vi "TestSequenceSubVI.vi"(0 "GuiRef":T2={"StringOut"=refnum, "AbortOnFail"=refnum, "SN"=refnum, "SN_Length"=refnum, "TestResult"=refnum, "CycleTime"=refnum, "ErrorCode"=refnum, "UUTStatus"=refnum, "DataBaseEnable?"=refnum, "DUTModel"=refnum, "FixtureID"=refnum, "OperatorID"=refnum, "SNReady"=refnum, "StopSlot"=refnum, "NextStep"=refnum, "PassYeild"=refnum, "Failed"=refnum, "Passed"=refnum, "Tested"=refnum, "TestItemsCtl"={"StepName"="", "TestEnable"=FALSE, "LoopCount"=0, "StopOnFail"=FALSE, "Index"=0, "TestName"="", "通道"="", "参数"="", "TimeStart"=0}, "ProcessBar"=refnum, "Slot"=enum."Slot1", "Row"=3, "States"=refnum, "TestMode"=refnum, "循环次数-DUT"=refnum, "波形图"=refnum, "产品型号"=refnum, "子面板"=refnum, "测试失败项目"=refnum, "测试结果"=refnum, "DUT"=refnum, "Starttime"=refnum, "SlotReady"=refnum, "版本信息"=refnum, "WIFI_1"=refnum, "WIFI_2"=refnum, "直通率"=refnum, "卡1开卡结果"=refnum, "卡2开卡结果"=refnum}, 7 "MSComm":refnum<k7>, 11 "error in":errorcluster, 14 "semaphore":T1 caption="信号量") -> (15 "error out":errorcluster)   [LabVIEW 2013]
uses:
  SystemCode/SysControl/Reference.ctl
  SystemCode/SysControl/TestItemsCTL.ctl
  SystemCode/SysControl/Slot.ctl
  SourceCode/PDINFO.ctl
  SystemCode/SysControl/LEDState.ctl
  <vilib>/measure/matone.llb/Extract Single Tone Information 1 Chan.vi
  SourceCode/GlobalValue.vi
  <vilib>/measure/madcrms.llb/Basic Averaged DC-RMS for 1 Chan.vi
  <vilib>/measure/matone.llb/SINAD Analyzer 1 Chan.vi
  <vilib>/addons/Sound and Vibration/svt_Distortion/SVT THD+N (Time) (1 Ch).vi
  <vilib>/ErrorRing/Error Ring.xnode
  <vilib>/measure/NI_MAPro.lvlib
  <vilib>/addons/Sound and Vibration/svt_Distortion/SoundVib_Distortion.lvlib
panel:
  out "错误输出":errorcluster
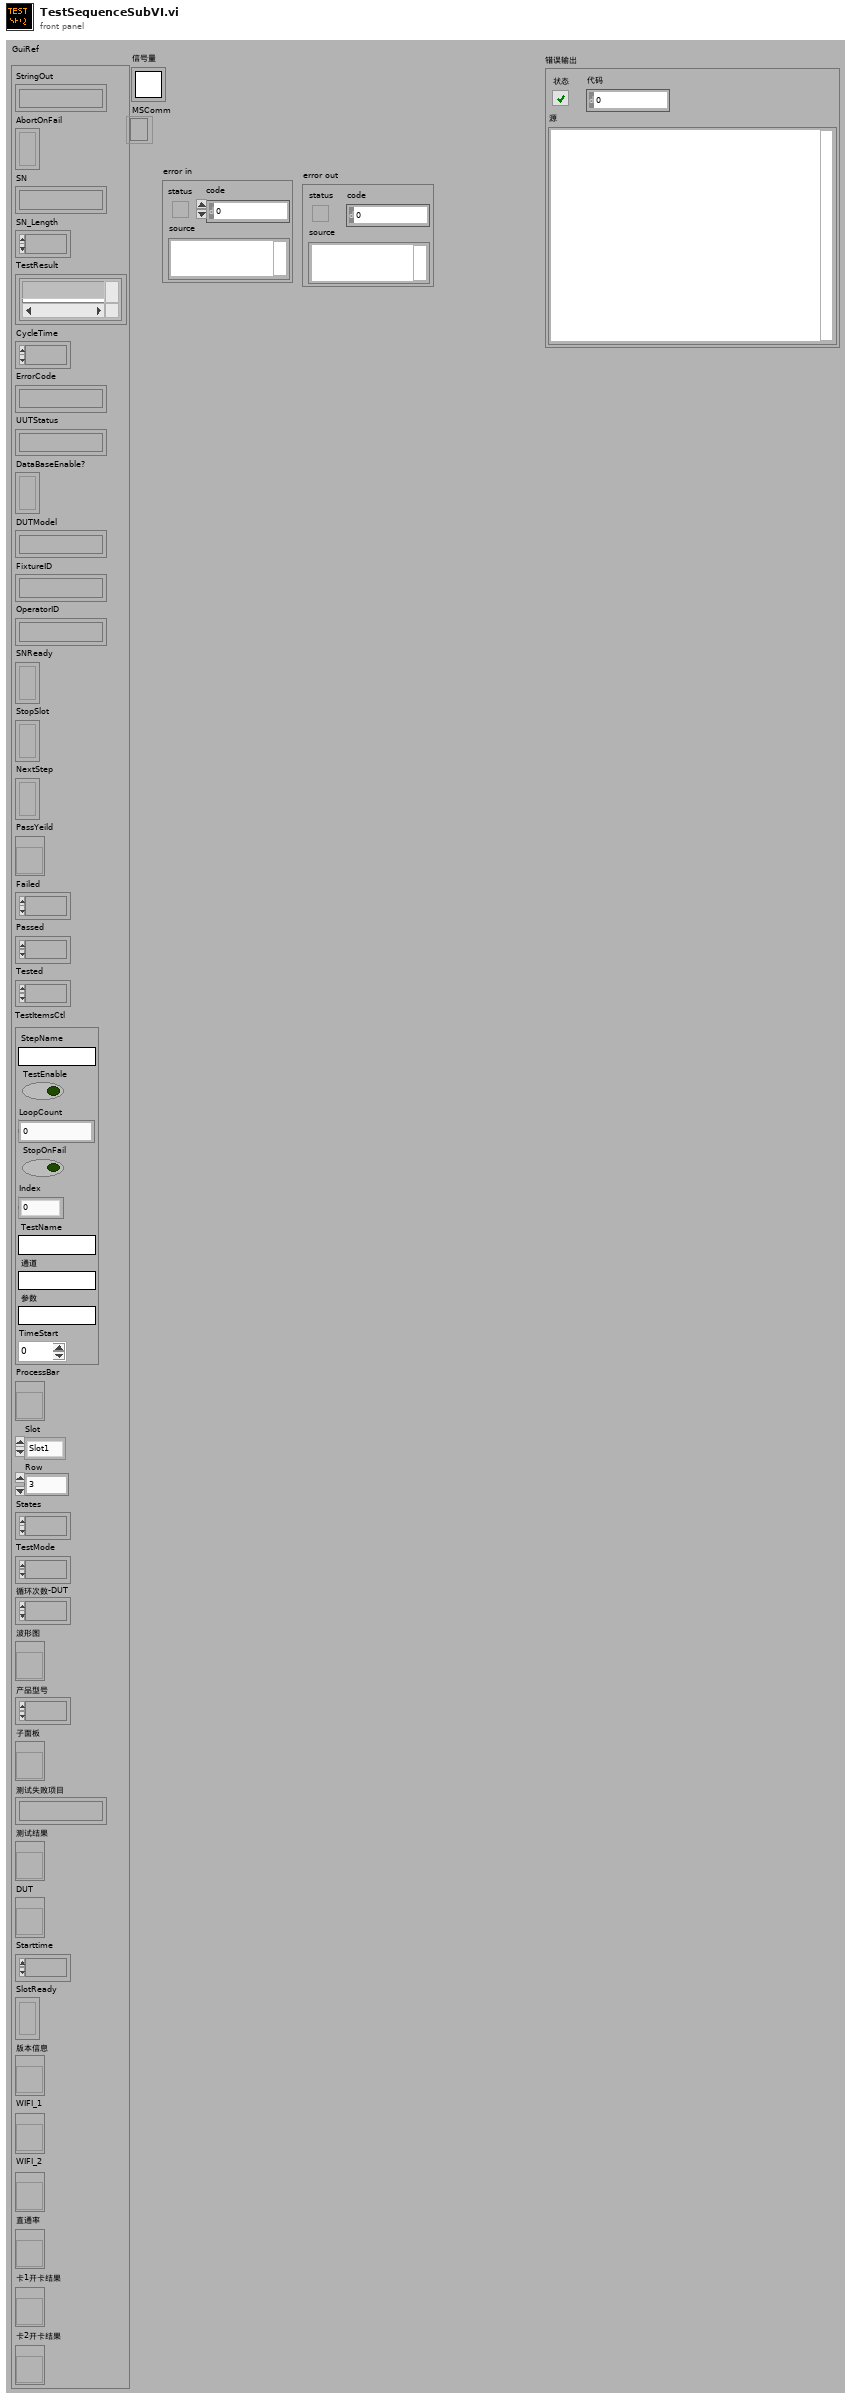
[diagram p1: front panel]
types:
  T1 = typedef "Semaphore RefNum" = refnum<k1>
  T2 = typedef "Reference.ctl" = cluster{"StringOut":refnum<vi>, "AbortOnFail":refnum<vi>, "SN":refnum<vi>, "SN_Length":refnum<vi>, "TestResult":refnum<vi>, "CycleTime":refnum<vi>, "ErrorCode":refnum<vi>, "UUTStatus":refnum<vi>, "DataBaseEnable?":refnum<vi>, "DUTModel":refnum<vi>, "FixtureID":refnum<vi>, "OperatorID":refnum<vi>, "SNReady":refnum<vi>, "StopSlot":refnum<vi>, "NextStep":refnum<vi>, "PassYeild":refnum<vi>, "Failed":refnum<vi>, "Passed":refnum<vi>, "Tested":refnum<vi>, "TestItemsCtl":T3, "ProcessBar":refnum<vi>, "Slot":T4, "Row":u32, "States":refnum<vi>, "TestMode":refnum<vi>, "循环次数-DUT":refnum<vi>, "波形图":refnum<vi>, "产品型号":refnum<vi>, "子面板":refnum<vi>, "测试失败项目":refnum<vi>, "测试结果":refnum<vi>, "DUT":refnum<vi>, "Starttime":refnum<vi>, "SlotReady":refnum<vi>, "版本信息":refnum<vi>, "WIFI_1":refnum<vi>, "WIFI_2":refnum<vi>, "直通率":refnum<vi>, "卡1开卡结果":refnum<vi>, "卡2开卡结果":refnum<vi>}
  T3 = typedef "TestItemsCTL.ctl" = cluster{"StepName":string, "TestEnable":bool, "LoopCount":i32, "StopOnFail":bool, "Index":u32, "TestName":string, "通道":string, "参数":string, "TimeStart":u32}
  T4 = typedef "Slot.ctl" = enum16{"Slot1", "Slot2", "Slot3", "Slot4"}
  T5 = typedef "PDINFO.ctl" = enum16{"Fw Ver", "HW Ver", "CCID", "WiFiName", "DevID", "SN", "TUID", "CertifID", "PdTime", "Provider", "WiFiPassword", "Imei", "AuthCode", "Reserved1", "Reserved2", "Reserved3"}
  T6 = cluster{"THD+N units":enum16{"dB", "linear ratio", "%"}, "detected fundamental amplitude units":enum16{"EU rms", "EU peak", "EU peak-peak"}}
  T7 = typedef "LEDState.ctl" = enum16{"默认", "闪烁", "停止闪烁", "真", "假"}
  T8 = cluster{"ID":u8, u8, u8, u8, "TimeStamp":u32, "TimeFlag":u8, "SendType":u8, "RemoteFlag":u8, "ExternFlag":u8, "DataLen":u8, "Byte0":u8, "Byte1":u8, "Byte2":u8, "Byte3":u8, "Byte4":u8, "Byte5":u8, "Byte6":u8, "Byte7":u8, "Channel":u8, u8, u8}
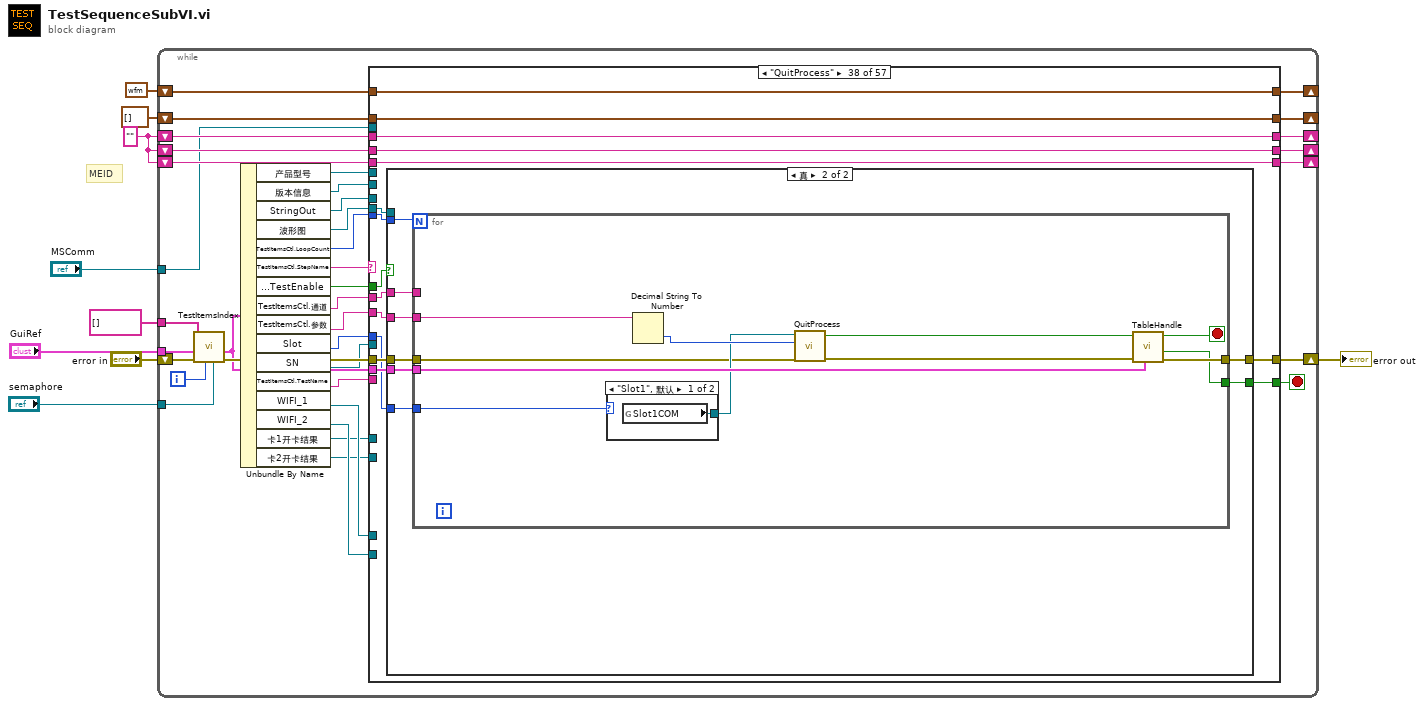
[diagram p0: block diagram]
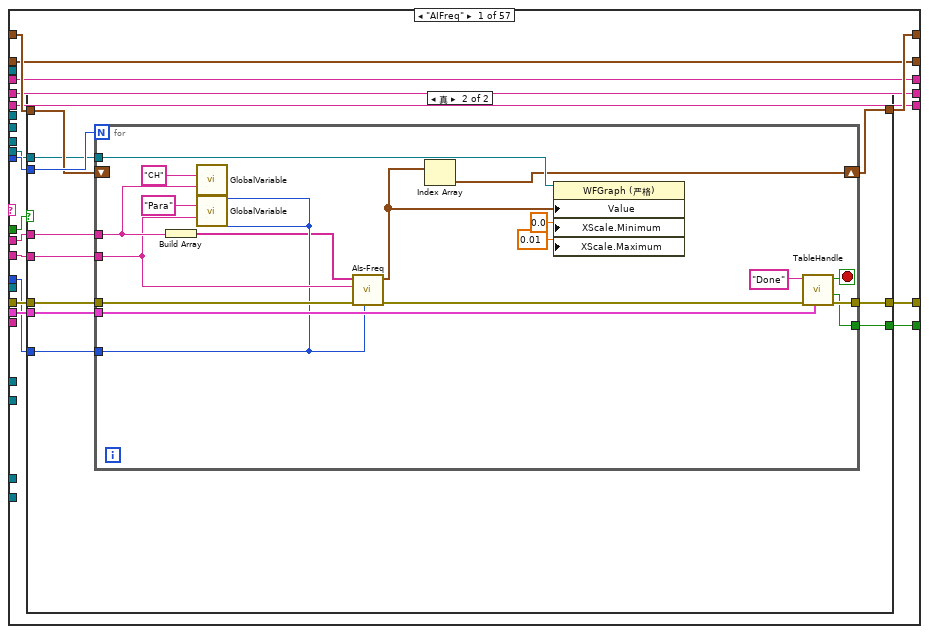
[diagram p2: hidden frame]
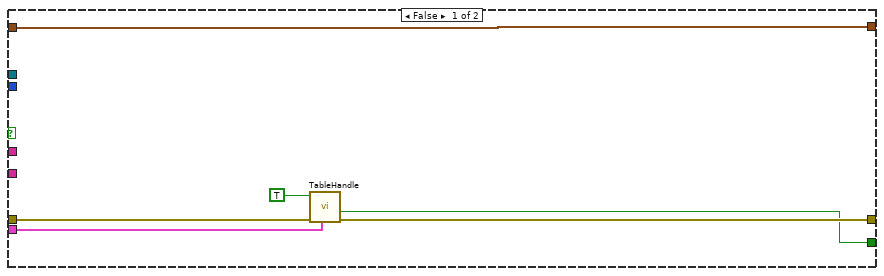
[diagram p3: hidden frame]
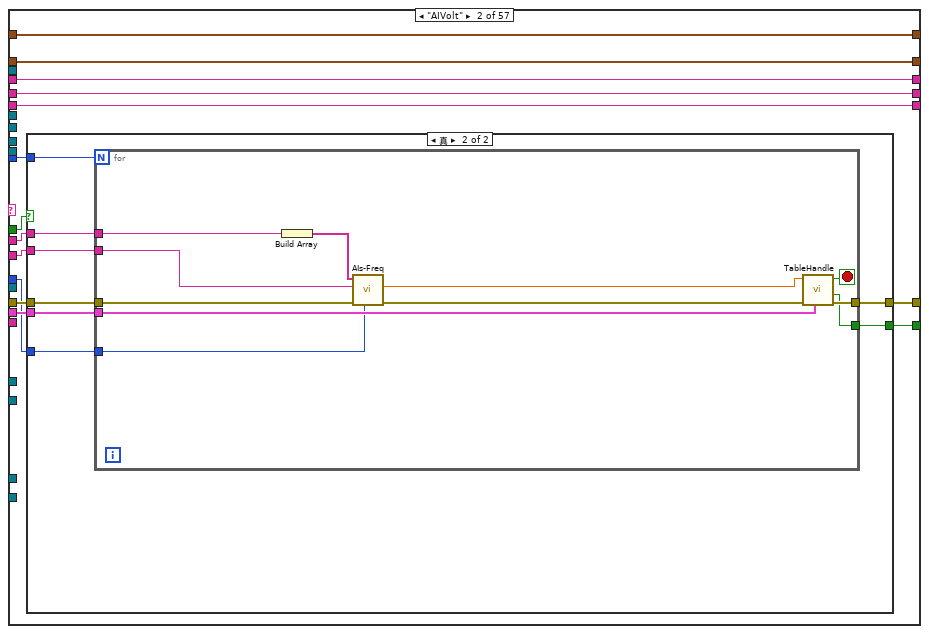
[diagram p4: hidden frame]
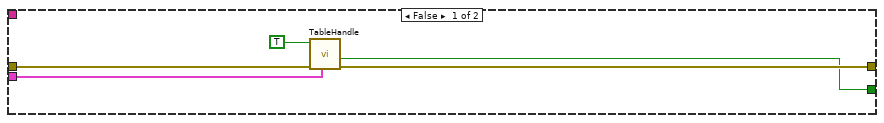
[diagram p5: hidden frame]
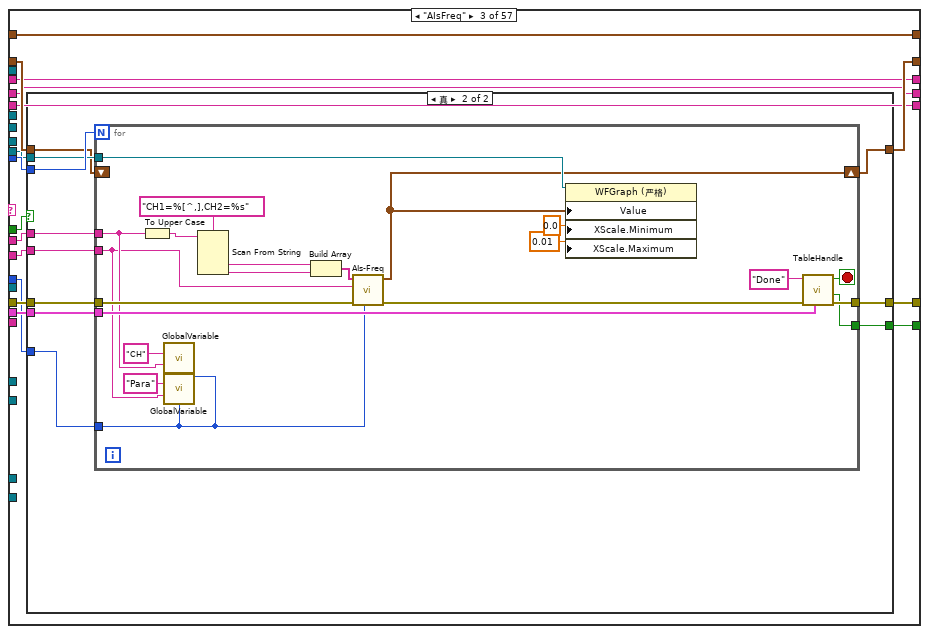
[diagram p6: hidden frame]
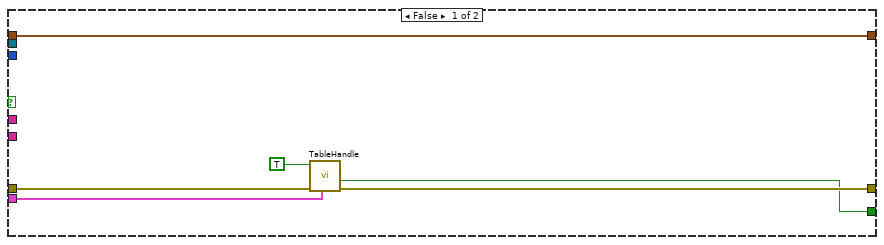
[diagram p7: hidden frame]
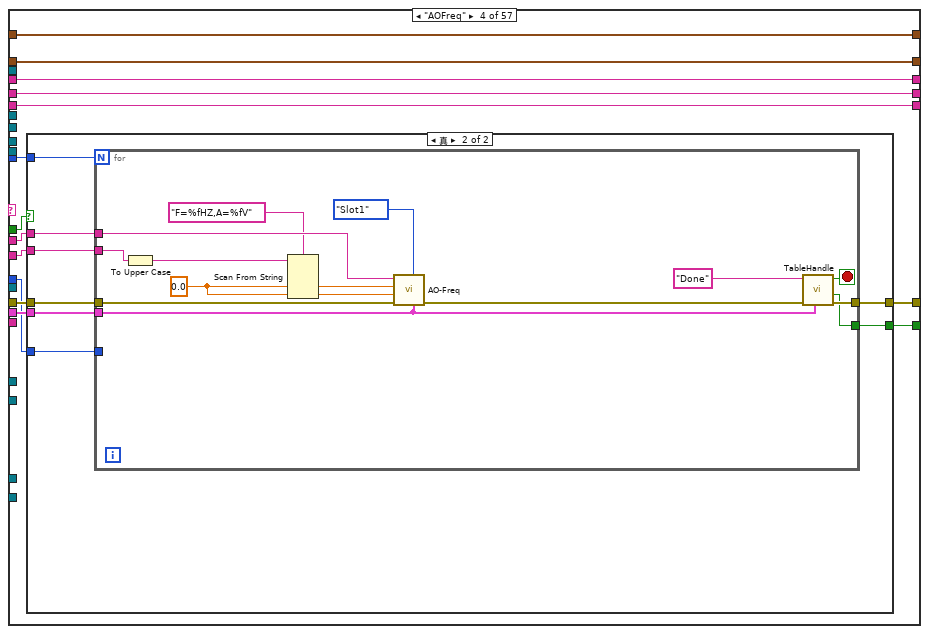
[diagram p8: hidden frame]
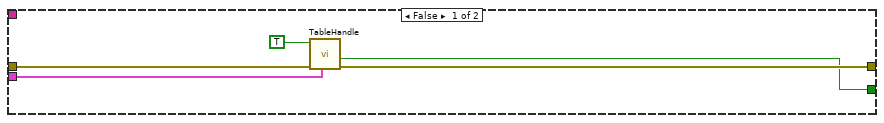
[diagram p9: hidden frame]
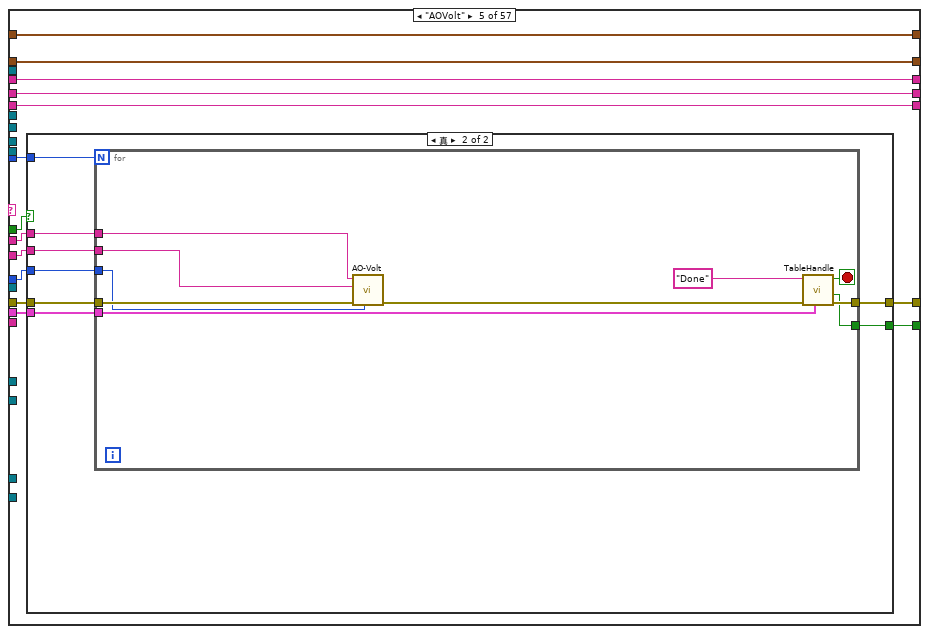
[diagram p10: hidden frame]
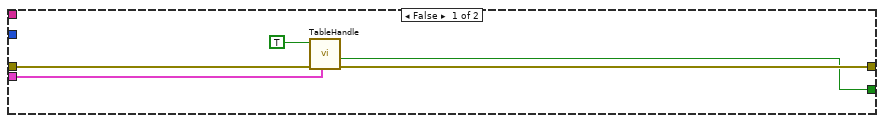
[diagram p11: hidden frame]
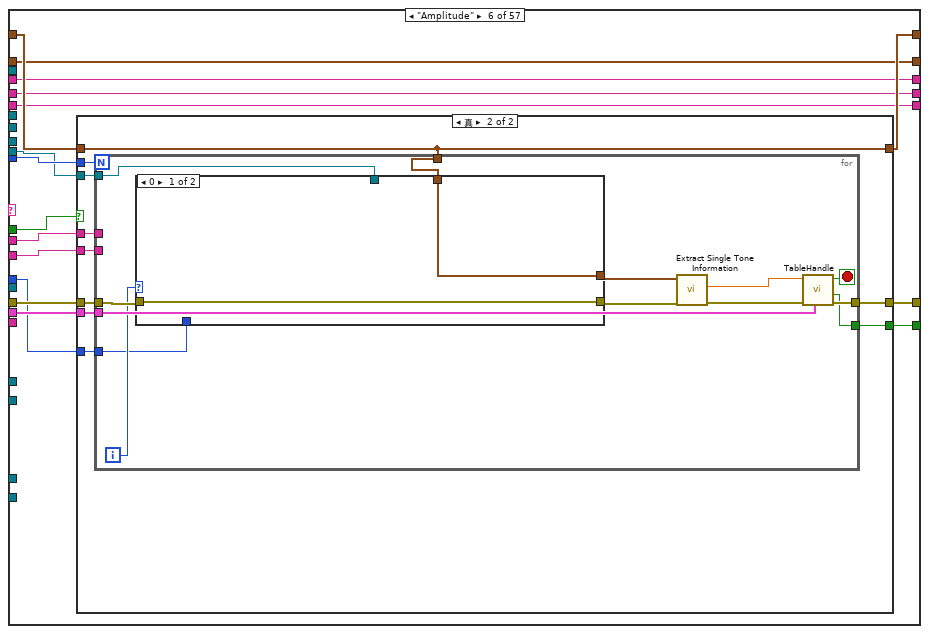
[diagram p12: hidden frame]
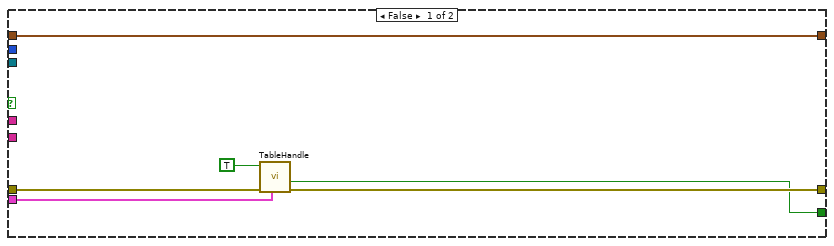
[diagram p13: hidden frame]
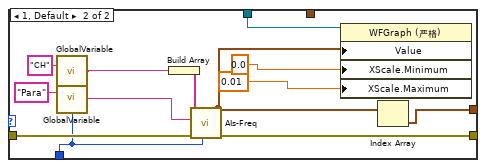
[diagram p14: hidden frame]
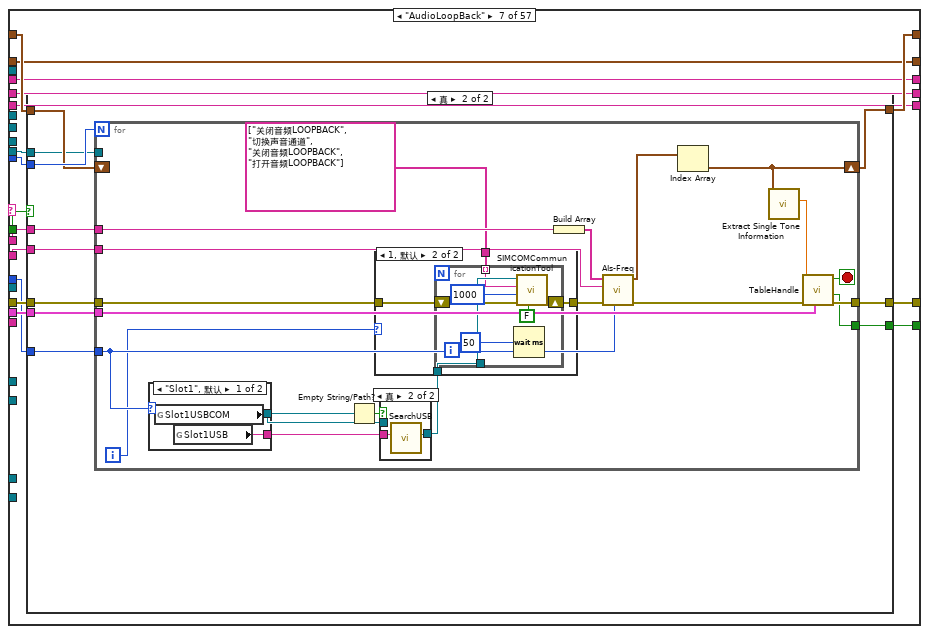
[diagram p15: hidden frame]
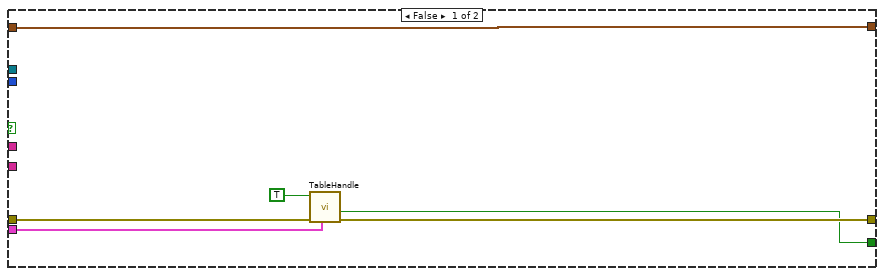
[diagram p16: hidden frame]
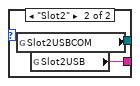
[diagram p19: hidden frame]
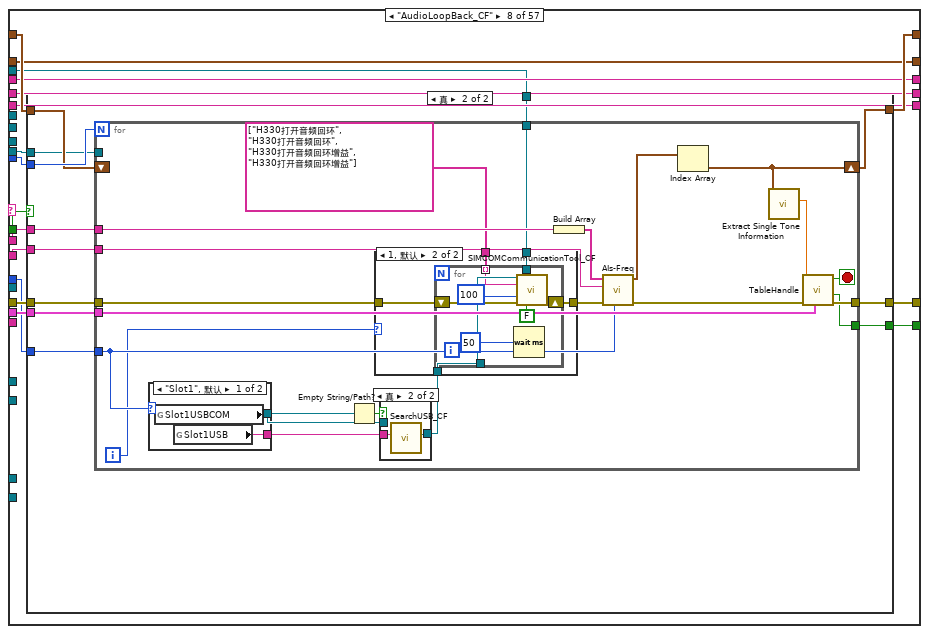
[diagram p20: hidden frame]
diagram:
  w2 = "" ("CMD")
  # "MEID"
  n1 = while {
    shift-right: [w41] -> w9
    shift-left: "error in" -> [w45]
    tunnel: "GuiRef" -> [w39]
    shift-right: [w33] -> _
    shift-left: waveform(dbl) {"t0"=timestamp(0 s since 1904-01-01), "dt"=1.0, "Y"=[]} ("Raw Data 3") -> [w32]
    shift-right: [w31] -> _
    shift-left: waveform(dbl)[] [] ("波形图") -> [w30]
    shift-right: [w27] -> _
    shift-left: w2 -> [w26]
    tunnel: string[] [] ("Fail项目") -> [w25]
    tunnel: "semaphore" -> [w23]
    shift-right: [w22] -> _
    shift-left: w2 -> [w21]
    shift-right: [w19] -> _
    shift-left: w2 -> [w20]
    tunnel: "MSComm" -> [w15]
    i -> [w24]
    stop <- w40 stop-if-true
    n2 = call "TestItemsIndex.vi"("semaphore"=w23, "TestItemIndexIn"=w24, "ErrorIn(NoError)"=w45, "GuiRef"=w39, "Fail项目"=w25) -> ("ErrorOut"=w44:errorcluster, "GuiRefOut"=w38:T2)  [unwired: 5 out]
    n3 = Unbundle By Name(w38) -> ("产品型号"=w16:refnum<vi>, "版本信息"=w18:refnum<vi>, "StringOut"=w28:refnum<vi>, "波形图"=w29:refnum<vi>, "TestItemsCtl.LoopCount"=w34:i32, "TestItemsCtl.StepName"=w43:string, "TestItemsCtl.TestEnable"=w42:bool, "TestItemsCtl.通道"=w35:string, "TestItemsCtl.参数"=w36:string, "Slot"=w37:T4, "SN"=w17:refnum<vi>, "TestItemsCtl.TestName"=w14:string, "WIFI_1"=w13:refnum<vi>, "WIFI_2"=w12:refnum<vi>, "卡1开卡结果"=w11:refnum<vi>, "卡2开卡结果"=w10:refnum<vi>)
    n4 = case shown="\"QuitProcess\"" w43 {
      selector: w43 -> [_ _ _ _ _ _ _ _ _ _ _ _ _ _ _ _ _ _ _ _ _ _ _ _ _ _ _ _ _ _ _ _ _ _ _ _ _ _ _ _ _ _ _ _ _ _ _ _ _ _ _ _ _ _ _ _ w3781]
      tunnel: [w59 w108 w148 w200 w242 w281 w341 w414 w491 w569 w647 w738 w825 w877 w929 w988 w1046 w1122 w1231 w1342 w1390 w1446 w1496 w1540 w1582 w1622 w1658 w1695 w1739 w1814 w1937 w2054 w2101 w2183 w2278 w2315 w2376 w2421 w2463 w2523 w2595 w2657 w2699 w2766 w2817 w2833 w2910 w2972 w3072 w3188 w3286 w3340 w3554 w3665 w3679 w3746 w3785] -> w41
      tunnel: w44 -> [w60 w109 w149 w201 w243 w282 w342 w415 w492 w570 w648 w739 w826 w878 w930 w989 w1047 w1123 w1232 w1343 w1391 w1447 w1497 w1541 w1583 w1623 w1659 w1696 w1740 w1815 w1938 w2055 w2105 w2184 w2279 w2316 w2377 w2422 w2464 w2524 w2596 w2658 w2700 w2770 w2817 w2834 w2911 w2973 w3073 w3189 w3287 w3331 w3555 w3665 w3680 w3747 _]
      tunnel: w38 -> [w61 w110 w150 w202 w244 w283 w343 w416 w493 w571 w649 w740 w827 w879 w931 w990 w1048 w1124 w1233 w1344 w1392 w1448 w1498 w1542 w1584 w1624 w1660 w1697 w1741 w1816 w1939 w2056 w2104 w2185 w2280 w2317 w2378 w2423 w2465 w2525 w2597 w2659 w2701 w2769 _ w2835 w2912 w2974 w3074 w3190 w3288 w3337 w3556 _ w3681 w3748 _]
      tunnel: w42 -> [w58 w107 w147 w199 w241 w280 w340 w413 w490 w568 w646 w737 w824 w876 w928 w987 w1045 w1121 w1230 w1341 w1389 w1445 w1495 w1539 w1581 w1621 w1657 w1694 w1738 w1813 w1936 w2053 w2108 w2182 w2277 w2314 w2375 w2420 w2462 w2522 w2594 w2656 w2698 w2764 _ w2832 w2909 w2971 w3071 w3187 w3285 w3332 w3553 _ w3678 w3745 _]
      tunnel: [w57 w106 w146 w198 w240 w279 w339 w412 w489 w567 w645 w736 w823 w875 w927 w986 w1044 w1120 w1229 w1340 w1388 w1444 w1494 w1538 w1580 w1620 w1656 w1693 w1737 w1812 w1935 w2052 w2100 w2181 w2276 w2313 w2374 w2419 w2461 w2521 w2593 w2655 w2697 w2767 TRUE ("StopOnFail?") w2831 w2908 w2970 w3070 w3186 w3284 w3339 w3552 FALSE ("StopOnFail?") w3677 w3744 TRUE ("StopOnFail?")] -> w40
      tunnel: w37 -> [w56 w105 w145 w197 w239 w278 w338 w411 w488 w566 w644 w735 w822 w874 w926 w985 w1043 w1119 w1228 w1339 w1387 w1443 w1493 w1537 w1579 w1619 w1655 w1692 w1736 w1811 w1934 w2051 w2103 w2180 w2275 w2312 w2373 w2418 w2460 w2520 w2592 w2654 w2696 w2768 _ w2830 w2907 w2969 w3069 w3185 w3283 w3341 w3551 _ w3676 w3743 w3776]
      tunnel: w36 -> [w54 w103 w143 w195 w237 w276 w336 w409 w486 w564 w642 w733 w820 w872 w924 w983 w1041 w1117 w1226 w1337 w1385 w1441 w1491 w1535 w1577 w1617 w1653 w1690 w1734 w1809 w1932 w2049 w2106 w2178 w2273 w2310 w2371 w2416 w2458 w2518 w2590 w2652 w2694 w2771 _ w2828 w2905 w2967 w3067 w3183 w3281 w3334 w3549 _ w3674 w3741 _]
      tunnel: w35 -> [w55 w104 w144 w196 w238 w277 w337 w410 w487 w565 w643 w734 w821 w873 w925 w984 w1042 w1118 w1227 w1338 w1386 w1442 w1492 w1536 w1578 w1618 w1654 w1691 w1735 w1810 w1933 w2050 w2107 w2179 w2274 w2311 w2372 w2417 w2459 w2519 w2591 w2653 w2695 w2772 _ w2829 w2906 w2968 w3068 w3184 w3282 w3342 w3550 _ w3675 w3742 _]
      tunnel: w34 -> [w53 w102 w142 w194 w236 w275 w335 w408 w485 w563 w641 w732 w819 w871 w923 w982 w1040 w1116 w1225 w1336 w1384 w1440 w1490 w1534 w1576 w1616 w1652 w1689 w1733 w1808 w1931 w2048 w2109 w2177 w2272 w2309 w2370 w2415 w2457 w2517 w2589 w2651 w2693 w2773 _ w2827 w2904 w2966 w3066 w3182 w3280 w3328 w3548 _ w3673 w3740 _]
      tunnel: [w52 w101 w141 w193 w235 w273 w334 w407 w484 w562 w640 w731 w818 w870 w922 w981 w1039 w1115 w1224 w1335 w1383 w1438 w1488 w1532 w1574 w1615 w1651 w1688 w1732 w1807 w1930 w2047 w2102 w2176 w2270 w2308 w2369 w2409 w2455 w2515 w2584 w2650 w2688 w2765 w2815 w2826 w2902 w2965 w3065 w3181 w3279 w3338 w3547 w3663 w3672 w3738 w3784] -> w33
      tunnel: w32 -> [w51 w101 w141 w193 w235 w274 w333 w406 w483 w561 w639 w730 w818 w870 w922 w981 w1039 w1115 w1224 w1335 w1383 w1439 w1489 w1533 w1575 w1615 w1651 w1688 w1732 w1807 w1930 w2047 w2102 w2176 w2271 w2308 w2369 w2409 w2456 w2516 w2584 w2650 w2688 w2765 w2815 w2826 w2903 w2965 w3065 w3181 w3279 w3338 w3547 w3663 w3672 w3739 w3784]
      tunnel: [w50 w100 w140 w192 w234 w272 w332 w405 w482 w560 w638 w729 w817 w869 w921 w980 w1038 w1114 w1223 w1334 w1382 w1437 w1487 w1531 w1573 w1614 w1650 w1687 w1731 w1806 w1929 w2046 w2112 w2175 w2269 w2307 w2368 w2414 w2454 w2514 w2588 w2649 w2692 w2777 w2814 w2825 w2901 w2964 w3064 w3180 w3278 w3345 w3546 w3662 w3671 w3737 w3783] -> w31
      tunnel: w30 -> [w50 w100 w139 w192 w234 w272 w332 w405 w482 w560 w638 w729 w817 w869 w921 w980 w1038 w1114 w1223 w1334 w1382 w1437 w1487 w1531 w1573 w1614 w1650 w1687 w1731 w1806 w1929 w2046 w2112 w2175 w2269 w2307 w2368 w2414 w2454 w2514 w2588 w2649 w2692 w2777 w2814 w2825 w2901 w2964 w3064 w3180 w3278 w3345 w3546 w3662 w3671 w3737 w3783]
      tunnel: w29 -> [w49 _ w138 _ _ w270 w331 w404 w481 w559 w637 w728 _ _ _ _ _ _ _ _ _ _ _ _ _ _ _ _ _ _ _ _ _ _ _ _ _ w2412 w2452 w2512 w2587 _ w2691 _ _ _ w2899 _ _ _ _ _ _ _ _ _ _]
      tunnel: w28 -> [_ _ _ _ _ _ _ _ _ _ w631 w722 w813 w868 w920 w979 w1037 w1113 w1222 w1333 w1381 _ _ _ _ _ _ _ w1730 w1805 w1928 _ w2099 _ _ _ _ _ _ _ w2583 _ w2687 _ _ w2824 _ w2963 w3063 w3179 _ w3330 w3542 _ w3667 _ _]
      tunnel: [w48 w97 w137 w191 w233 w271 w330 w403 w480 w558 w630 w721 w812 w867 w919 w978 w1036 w1112 w1221 w1331 w1379 w1436 w1486 w1530 w1572 w1613 w1649 w1686 w1729 w1804 w1927 w2045 w2096 w2174 w2268 w2306 w2367 w2413 w2453 w2513 w2580 w2648 w2684 w2776 w2813 w2823 w2900 w2962 w3062 w3178 w3277 w3329 w3541 w3661 w3666 w3736 w3778] -> w27
      tunnel: w26 -> [w48 w97 w137 w191 w233 w271 w330 w403 w480 w558 w632 w723 w814 w866 w918 w977 w1035 w1111 w1220 w1332 w1380 w1436 w1486 w1530 w1572 w1613 w1649 w1686 w1728 w1803 w1926 w2045 w2097 w2174 w2268 w2306 w2367 w2413 w2453 w2513 w2581 w2648 w2685 w2776 w2813 w2822 w2900 w2961 w3061 w3177 w3277 w3327 w3543 w3661 w3668 w3736 w3778]
      tunnel: [w47 w99 w136 w190 w232 w269 w329 w402 w479 w557 w636 w727 w816 w865 w917 w976 w1034 w1110 w1219 w1330 w1378 w1433 w1485 w1529 w1571 w1612 w1648 w1685 w1727 w1802 w1925 w2044 w2111 w2173 w2267 w2305 w2366 w2411 w2451 w2511 w2586 w2647 w2690 w2775 w2812 w2821 w2898 w2960 w3060 w3176 w3276 w3344 w3545 w3660 w3670 w3735 w3774] -> w22
      tunnel: w21 -> [w47 w99 w136 w190 w232 w269 w329 w402 w479 w557 w636 w727 w816 w865 w917 w976 w1034 w1110 w1219 w1330 w1378 w1433 w1485 w1529 w1571 w1612 w1648 w1685 w1727 w1802 w1925 w2044 w2111 w2173 w2267 w2305 w2366 w2411 w2451 w2511 w2586 w2647 w2690 w2775 w2812 w2821 w2898 w2959 w3059 w3175 w3276 w3344 w3545 w3660 w3670 w3735 w3774]
      tunnel: w20 -> [w46 w98 w135 w189 w231 w268 w328 w401 w478 w556 w635 w726 w815 w864 w916 w975 _ w1109 _ w1329 w1377 w1435 w1484 w1528 w1570 w1611 w1647 w1684 _ _ _ w2043 w2110 w2172 w2266 w2304 w2365 w2410 w2450 w2510 w2585 w2646 w2689 w2774 w2811 _ w2897 w2958 w3058 w3174 w3275 w3343 w3544 w3659 w3669 w3734 w3773]
      tunnel: [w46 w98 w135 w189 w231 w268 w328 w401 w478 w556 w635 w726 w815 w864 w916 w975 w1033 w1109 w1218 w1329 w1377 w1435 w1484 w1528 w1570 w1611 w1647 w1684 w1726 w1801 w1924 w2043 w2110 w2172 w2266 w2304 w2365 w2410 w2450 w2510 w2585 w2646 w2689 w2774 w2811 w2820 w2897 w2958 w3058 w3174 w3275 w3343 w3544 w3659 w3669 w3734 w3773] -> w19
      tunnel: w18 -> [_ _ _ _ _ _ _ _ _ _ _ _ _ _ _ _ w1032 _ w1217 _ _ _ _ _ _ _ _ _ w1725 w1800 w1923 _ _ _ _ _ _ _ _ _ _ _ _ _ _ w2819 _ _ _ _ _ _ _ _ _ _ _]
      tunnel: w17 -> [_ _ _ _ _ _ _ _ _ _ _ _ _ _ _ _ w1031 _ w1216 _ w1375 w1434 w1483 w1527 w1569 _ _ _ w1724 w1799 w1922 _ _ _ _ _ _ _ _ _ _ _ _ _ _ w2818 _ _ _ _ _ w3333 _ _ _ _ _]
      tunnel: w16 -> [_ _ _ _ _ _ _ _ _ w554 w633 w724 _ _ _ _ w1030 _ w1215 _ w1376 _ _ _ _ _ _ _ w1723 _ _ _ _ _ _ _ _ _ _ _ _ _ w2683 _ _ _ _ _ _ _ _ w3336 w3540 _ _ _ _]
      tunnel: w15 -> [_ _ _ _ _ _ _ w400 w477 w555 w634 w725 _ _ _ _ _ _ _ _ _ _ _ _ _ _ _ _ _ _ _ _ _ w2171 _ _ _ _ _ _ _ _ _ _ _ _ _ _ w3057 w3173 _ _ _ _ _ _ _]
      tunnel: w14 -> [_ _ _ _ _ _ _ _ _ _ _ _ _ _ _ _ _ _ _ _ _ _ _ _ _ _ _ _ _ w1798 w1921 _ w2098 _ _ _ _ _ _ _ w2582 _ w2686 _ _ _ _ _ _ _ _ w3335 _ _ _ _ _]
      tunnel: w13 -> [_ _ _ _ _ _ _ _ _ _ _ _ _ _ _ _ _ _ w1214 _ _ _ _ _ _ _ _ _ _ _ _ _ _ _ _ _ _ _ _ _ _ _ _ _ _ _ _ _ _ _ _ _ _ _ _ _ _]
      tunnel: w12 -> [_ _ _ _ _ _ _ _ _ _ _ _ _ _ _ _ _ _ w1213 _ _ _ _ _ _ _ _ _ _ _ _ _ _ _ _ _ _ _ _ _ _ _ _ _ _ _ _ _ _ _ _ _ _ _ _ _ _]
      tunnel: w11 -> [_ _ _ _ _ _ _ _ _ _ _ _ _ _ _ _ _ _ _ _ _ _ _ _ _ _ _ _ _ _ _ _ _ _ _ _ _ _ _ _ _ _ _ _ _ _ _ _ _ _ _ _ w3539 _ _ _ _]
      tunnel: w10 -> [_ _ _ _ _ _ _ _ _ _ _ _ _ _ _ _ _ _ _ _ _ _ _ _ _ _ _ _ _ _ _ _ _ _ _ _ _ _ _ _ _ _ _ _ _ _ _ _ _ _ _ _ w3538 _ _ _ _]
      frame "AIFreq" {
        n5 = case shown="真" w58 {
          tunnel: w61 -> [w65 w76]
          tunnel: w60 -> [w66 w78]
          tunnel: [w67 w77] -> w59
          tunnel: [w64 w75] -> w57
          tunnel: w56 -> [_ w74]
          tunnel: w55 -> [_ w73]
          tunnel: w54 -> [_ w72]
          tunnel: w53 -> [_ w71]
          tunnel: [w62 w70] -> w52
          tunnel: w51 -> [w62 w69]
          tunnel: w49 -> [_ w68]
          frame False {
            n6 = call "TableHandle.vi"("All"=w65, "error in (no error)"=w66, "DataIn"=TRUE) -> ("error out"=w67:errorcluster, "Stop?"=w64:bool)  [unwired: 3 in, 4 out]
          }
          frame True {
            n7 = for "For循环" {
              N: w71 -> [_]
              tunnel: w78 -> [w92]
              tunnel: [w96] -> w77
              tunnel: w76 -> [w93]
              tunnel: [w94] -> w75
              tunnel: w74 -> [w81]
              tunnel: w72 -> [w82]
              tunnel: w73 -> [w84]
              shift-right: [w86] -> w70
              shift-left: w69 -> [_]
              tunnel: w68 -> [w88]
              stop <- w95 stop-if-true
              n8 = Build Array(w84) -> (w80:string[])
              n9 = call "GlobalVariable.vi"("Name"="CH", "ValueIn"=w84, "Slot"=w81) -> ()  [unwired: 9 in, 4 out]
              n10 = call "GlobalVariable.vi"("Name"="Para", "ValueIn"=w82, "Slot"=w81) -> ()  [unwired: 9 in, 4 out]
              n11 = call "AIs-Freq.vi"("Slot"=w81, "error in"=w92, "Mode"=w82, "CHs"=w80) -> ("error out"=w91:errorcluster, "波形图"=w79:waveform(dbl)[])  [unwired: 5 in, 1 out]
              n12 = Index Array(array=w79) -> (element=w86:waveform(dbl))  [unwired: 1 in]
              n13 = property class="WFGraph (严格)"(reference=w88, "Value"=w79, "XScale.Minimum"=0.0 ("X标尺.范围:最小值"), "XScale.Maximum"=0.01 ("X标尺.范围:最大值")) -> ()  [unwired: 1 in, 2 out]
              n14 = call "TableHandle.vi"("All"=w93, "error in (no error)"=w91, "DataIn"="Done") -> ("error out"=w96:errorcluster, "Stop?"=w94:bool, "StopForLoop"=w95:bool)  [unwired: 4 in, 2 out]
            }
          }
        }
      }
      frame "AIVolt" {
        n15 = case shown="真" w107 {
          tunnel: w110 -> [w113 w121]
          tunnel: w109 -> [w114 w123]
          tunnel: [w115 w122] -> w108
          tunnel: [w112 w120] -> w106
          tunnel: w105 -> [_ w119]
          tunnel: w104 -> [_ w118]
          tunnel: w103 -> [_ w117]
          tunnel: w102 -> [_ w116]
          frame False {
            n16 = call "TableHandle.vi"("All"=w113, "error in (no error)"=w114, "DataIn"=TRUE) -> ("error out"=w115:errorcluster, "Stop?"=w112:bool)  [unwired: 3 in, 4 out]
          }
          frame True {
            n17 = for "For循环" {
              N: w116 -> [_]
              tunnel: w123 -> [w130]
              tunnel: [w134] -> w122
              tunnel: w121 -> [w131]
              tunnel: [w132] -> w120
              tunnel: w119 -> [w127]
              tunnel: w117 -> [w128]
              tunnel: w118 -> [w126]
              stop <- w133 stop-if-true
              n18 = Build Array(w126) -> (w125:string[])
              n19 = call "AIs-Freq.vi"("Slot"=w127, "error in"=w130, "Mode"=w128, "CHs"=w125) -> ("error out"=w129:errorcluster, "RMS value"=w124:dbl)  [unwired: 5 in, 1 out]
              n20 = call "TableHandle.vi"("All"=w131, "error in (no error)"=w129, "DataIn"=w124) -> ("error out"=w134:errorcluster, "Stop?"=w132:bool, "StopForLoop"=w133:bool)  [unwired: 4 in, 2 out]
            }
          }
        }
      }
      frame "AIsFreq" {
        n21 = case shown="真" w147 {
          tunnel: w150 -> [w154 w165]
          tunnel: w149 -> [w155 w167]
          tunnel: [w156 w166] -> w148
          tunnel: [w153 w164] -> w146
          tunnel: w145 -> [_ w163]
          tunnel: w144 -> [_ w162]
          tunnel: w143 -> [_ w161]
          tunnel: w142 -> [_ w160]
          tunnel: [w151 w159] -> w140
          tunnel: w139 -> [w151 w157]
          tunnel: w138 -> [_ w158]
          frame False {
            n22 = call "TableHandle.vi"("All"=w154, "error in (no error)"=w155, "DataIn"=TRUE) -> ("error out"=w156:errorcluster, "Stop?"=w153:bool)  [unwired: 3 in, 4 out]
          }
          frame True {
            n23 = for "For循环" {
              N: w160 -> [_]
              tunnel: w167 -> [w184]
              tunnel: [w188] -> w166
              tunnel: w165 -> [w185]
              tunnel: [w186] -> w164
              tunnel: w163 -> [w170]
              tunnel: w161 -> [w171]
              tunnel: w162 -> [w172]
              shift-right: [w168] -> w159
              shift-left: w157 -> [_]
              tunnel: w158 -> [w177]
              stop <- w187 stop-if-true
              n24 = To Upper Case(1:w172) -> (0:w181:string)
              n25 = call "GlobalVariable.vi"("Name"="CH", "ValueIn"=w172, "Slot"=w170) -> ()  [unwired: 9 in, 4 out]
              n26 = call "GlobalVariable.vi"("Name"="Para", "ValueIn"=w171, "Slot"=w170) -> ()  [unwired: 9 in, 4 out]
              n27 = Scan From String(format string="CH1=%[^,],CH2=%s" ("格式字符串"), input string=w181) -> (output 1=w179:string, output 2=w178:string)  [unwired: 4 in, 3 out]
              n28 = Build Array(w179, w178) -> (w169:string[])
              n29 = call "AIs-Freq.vi"("Slot"=w170, "error in"=w184, "Mode"=w171, "CHs"=w169) -> ("error out"=w183:errorcluster, "波形图"=w168:waveform(dbl)[])  [unwired: 5 in, 1 out]
              n30 = property class="WFGraph (严格)"(reference=w177, "Value"=w168, "XScale.Minimum"=0.0 ("X标尺.范围:最小值"), "XScale.Maximum"=0.01 ("X标尺.范围:最大值")) -> ()  [unwired: 1 in, 2 out]
              n31 = call "TableHandle.vi"("All"=w185, "error in (no error)"=w183, "DataIn"="Done") -> ("error out"=w188:errorcluster, "Stop?"=w186:bool, "StopForLoop"=w187:bool)  [unwired: 4 in, 2 out]
            }
          }
        }
      }
      frame "AOFreq" {
        n32 = case shown="真" w199 {
          tunnel: w202 -> [w205 w213]
          tunnel: w201 -> [w206 w215]
          tunnel: [w207 w214] -> w200
          tunnel: [w204 w212] -> w198
          tunnel: w197 -> [_ w211]
          tunnel: w196 -> [_ w210]
          tunnel: w195 -> [_ w209]
          tunnel: w194 -> [_ w208]
          frame False {
            n33 = call "TableHandle.vi"("All"=w205, "error in (no error)"=w206, "DataIn"=TRUE) -> ("error out"=w207:errorcluster, "Stop?"=w204:bool)  [unwired: 3 in, 4 out]
          }
          frame True {
            n34 = for "For循环" {
              N: w208 -> [_]
              tunnel: w215 -> [w227]
              tunnel: [w230] -> w214
              tunnel: w213 -> [w217]
              tunnel: [w228] -> w212
              tunnel: w211 -> [_]
              tunnel: w209 -> [w222]
              tunnel: w210 -> [w225]
              stop <- w229 stop-if-true
              w221 = 0.0 ("默认值 1")
              n35 = To Upper Case(1:w222) -> (0:w220:string)
              n36 = Scan From String(format string="F=%fHZ,A=%fV" ("格式字符串"), input string=w220, default 1=w221, default 2=w221) -> (output 1=w219:dbl, output 2=w218:dbl)  [unwired: 2 in, 3 out]
              n37 = call "AO-Freq.vi"("GuiRef"=w217, "Slot"=Slot."Slot1", "error in"=w227, "AMP"=w218, "Freq"=w219, "CH"=w225) -> ("error out"=w226:errorcluster)  [unwired: 5 in]
              n38 = call "TableHandle.vi"("All"=w217, "error in (no error)"=w226, "DataIn"="Done") -> ("error out"=w230:errorcluster, "Stop?"=w228:bool, "StopForLoop"=w229:bool)  [unwired: 4 in, 2 out]
            }
          }
        }
      }
      frame "AOVolt" {
        n39 = case shown="真" w241 {
          tunnel: w244 -> [w247 w255]
          tunnel: w243 -> [w248 w257]
          tunnel: [w249 w256] -> w242
          tunnel: [w246 w254] -> w240
          tunnel: w239 -> [_ w253]
          tunnel: w238 -> [_ w252]
          tunnel: w237 -> [_ w251]
          tunnel: w236 -> [_ w250]
          frame False {
            n40 = call "TableHandle.vi"("All"=w247, "error in (no error)"=w248, "DataIn"=TRUE) -> ("error out"=w249:errorcluster, "Stop?"=w246:bool)  [unwired: 3 in, 4 out]
          }
          frame True {
            n41 = for "For循环" {
              N: w250 -> [_]
              tunnel: w257 -> [w263]
              tunnel: [w267] -> w256
              tunnel: w255 -> [w264]
              tunnel: [w265] -> w254
              tunnel: w253 -> [w258]
              tunnel: w251 -> [w259]
              tunnel: w252 -> [w261]
              stop <- w266 stop-if-true
              n42 = call "AO-Volt.vi"("Slot"=w258, "error in"=w263, "Value"=w259, "CH"=w261) -> ("error out"=w262:errorcluster)  [unwired: 7 in]
              n43 = call "TableHandle.vi"("All"=w264, "error in (no error)"=w262, "DataIn"="Done") -> ("error out"=w267:errorcluster, "Stop?"=w265:bool, "StopForLoop"=w266:bool)  [unwired: 4 in, 2 out]
            }
          }
        }
      }
      frame "Amplitude" {
        n44 = case shown="真" w280 {
          tunnel: w283 -> [w287 w297]
          tunnel: w282 -> [w288 w299]
          tunnel: [w289 w298] -> w281
          tunnel: [w286 w296] -> w279
          tunnel: w278 -> [_ w295]
          tunnel: w277 -> [_ w294]
          tunnel: w276 -> [_ w293]
          tunnel: w275 -> [_ w292]
          tunnel: w274 -> [w284 w291]
          tunnel: [w284 w291] -> w273
          tunnel: w270 -> [_ w290]
          frame False {
            n45 = call "TableHandle.vi"("All"=w287, "error in (no error)"=w288, "DataIn"=TRUE) -> ("error out"=w289:errorcluster, "Stop?"=w286:bool)  [unwired: 3 in, 4 out]
          }
          frame True {
            n46 = for "For循环" {
              N: w292 -> [_]
              tunnel: w299 -> [w306]
              tunnel: [w312] -> w298
              tunnel: w297 -> [w309]
              tunnel: [w310] -> w296
              tunnel: w295 -> [w300]
              tunnel: w293 -> [_]
              tunnel: w294 -> [_]
              tunnel: w291 -> [w303]
              tunnel: w290 -> [w301]
              i -> [w304]
              stop <- w311 stop-if-true
              n47 = case shown="0" w304 {
                tunnel: w306 -> [w314 w325]
                tunnel: [w314 w324] -> w305
                tunnel: w301 -> [_ w323]
                tunnel: w300 -> [_ w319]
                tunnel: [w313 w320] -> w302
                tunnel: w303 -> [w313 _]
                frame 0 {
                }
                frame 1, Default {
                  n48 = call "GlobalVariable.vi"("Name"="CH", "Slot"=w319) -> ("String"=w318:string)  [unwired: 10 in, 3 out]
                  n49 = call "GlobalVariable.vi"("Name"="Para", "Slot"=w319) -> ("String"=w317:string)  [unwired: 10 in, 3 out]
                  n50 = Build Array(w318) -> (w322:string[])
                  n51 = call "AIs-Freq.vi"("Slot"=w319, "error in"=w325, "Mode"=w317, "CHs"=w322) -> ("error out"=w324:errorcluster, "波形图"=w321:waveform(dbl)[])  [unwired: 5 in, 1 out]
                  n52 = property class="WFGraph (严格)"(reference=w323, "Value"=w321, "XScale.Minimum"=0.0 ("X标尺.范围:最小值"), "XScale.Maximum"=0.01 ("X标尺.范围:最大值")) -> ()  [unwired: 1 in, 2 out]
                  n53 = Index Array(array=w321) -> (element=w320:waveform(dbl))  [unwired: 1 in]
                }
              }
              n54 = call-poly <vilib>:"Extract Single Tone Information.vi"("error in (no error)"=w305, "time signal in"=w302) -> ("error out"=w308:errorcluster, "detected amplitude"=w307:dbl)  [unwired: 4 in, 4 out]
              n55 = call "TableHandle.vi"("All"=w309, "error in (no error)"=w308, "DataIn"=w307) -> ("error out"=w312:errorcluster, "Stop?"=w310:bool, "StopForLoop"=w311:bool)  [unwired: 4 in, 2 out]
            }
          }
        }
      }
      frame "AudioLoopBack" {
        n56 = case shown="真" w340 {
          tunnel: w343 -> [w347 w358]
          tunnel: w342 -> [w348 w360]
          tunnel: [w349 w359] -> w341
          tunnel: [w346 w357] -> w339
          tunnel: w338 -> [_ w356]
          tunnel: w337 -> [_ w355]
          tunnel: w336 -> [_ w354]
          tunnel: w335 -> [_ w353]
          tunnel: [w344 w352] -> w334
          tunnel: w333 -> [w344 w351]
          tunnel: w331 -> [_ w350]
          frame False {
            n57 = call "TableHandle.vi"("All"=w347, "error in (no error)"=w348, "DataIn"=TRUE) -> ("error out"=w349:errorcluster, "Stop?"=w346:bool)  [unwired: 3 in, 4 out]
          }
          frame True {
            n58 = for "For循环" {
              N: w353 -> [_]
              tunnel: w360 -> [w371]
              tunnel: [w380] -> w359
              tunnel: w358 -> [w377]
              tunnel: [w378] -> w357
              tunnel: w356 -> [w367]
              tunnel: w354 -> [w374]
              tunnel: w355 -> [w375]
              shift-right: [w363] -> w352
              shift-left: w351 -> [_]
              tunnel: w350 -> [_]
              i -> [w361]
              stop <- w379 stop-if-true
              n59 = case shown="\"Slot1\", 默认" w367 {
                tunnel: [w396 w399] -> w364
                tunnel: [w397 w398] -> w368
                frame "Slot1", Default {
                  n60 = global read "GlobalValue.vi" "Slot1USBCOM"() -> (w396:refnum<visa-resource-name>)
                  n61 = global read "GlobalValue.vi" "Slot1USB"() -> (w397:string)
                }
                frame "Slot2" {
                  n62 = global read "GlobalValue.vi" "Slot2USBCOM"() -> (w399:refnum<visa-resource-name>)
                  n63 = global read "GlobalValue.vi" "Slot2USB"() -> (w398:string)
                }
              }
              n64 = Empty String/Path?(string/path=w364) -> (empty?=w369:bool)
              n65 = case shown="真" w369 {
                tunnel: [w393 w395] -> w366
                tunnel: w368 -> [_ w394]
                tunnel: w364 -> [w393 _]
                frame False {
                }
                frame True {
                  n66 = call "SearchUSB.vi"("USB"=w394) -> ("USBPort"=w395:refnum<visa-resource-name>)  [unwired: 9 in, 1 out]
                }
              }
              n67 = case shown="1, 默认" w361 {
                tunnel: w371 -> [w381 w385]
                tunnel: [w381 w384] -> w370
                tunnel: w366 -> [_ w383]
                tunnel: string[] ["关闭音频LOOPBACK", "切换声音通道", "关闭音频LOOPBACK", "打开音频LOOPBACK"] -> [_ w382]
                frame 0 {
                }
                frame 1, Default {
                  n68 = for {
                    tunnel: w383 -> [w390]
                    shift-right: [w391] -> w384
                    shift-left: w385 -> [w392]
                    tunnel: w382 -> [w387] mode=indexing
                    n69 = Wait (ms)(milliseconds to wait=u32 50 ("等待时间（毫秒）")) -> ()  [unwired: 1 out]
                    n70 = call "SIMCOMCommunicationTool.vi"("Debug"=FALSE, "error in"=w392, "DelayTime"=u32 1000, "通信协议名称"=w387, "VISA资源名称"=w390) -> ("error out"=w391:errorcluster)  [unwired: 2 in, 4 out]
                  }
                }
              }
              n71 = Build Array(w375) -> (w373:string[])
              n72 = call "AIs-Freq.vi"("Slot"=w367, "error in"=w370, "Mode"=w374, "CHs"=w373) -> ("error out"=w376:errorcluster, "波形图"=w372:waveform(dbl)[])  [unwired: 5 in, 1 out]
              n73 = Index Array(array=w372) -> (element=w363:waveform(dbl))  [unwired: 1 in]
              n74 = call-poly <vilib>:"Extract Single Tone Information.vi"("time signal in"=w363) -> ("detected amplitude"=w362:dbl)  [unwired: 5 in, 5 out]
              n75 = call "TableHandle.vi"("All"=w377, "error in (no error)"=w376, "DataIn"=w362) -> ("error out"=w380:errorcluster, "Stop?"=w378:bool, "StopForLoop"=w379:bool)  [unwired: 4 in, 2 out]
            }
          }
        }
      }
      frame "AudioLoopBack_CF" {
        n76 = case shown="真" w413 {
          tunnel: w416 -> [w420 w432]
          tunnel: w415 -> [w421 w434]
          tunnel: [w422 w433] -> w414
          tunnel: [w419 w431] -> w412
          tunnel: w411 -> [_ w430]
          tunnel: w410 -> [_ w429]
          tunnel: w409 -> [_ w428]
          tunnel: w408 -> [_ w427]
          tunnel: [w417 w426] -> w407
          tunnel: w406 -> [w417 w425]
          tunnel: w404 -> [_ w424]
          tunnel: w400 -> [_ w423]
          frame False {
            n77 = call "TableHandle.vi"("All"=w420, "error in (no error)"=w421, "DataIn"=TRUE) -> ("error out"=w422:errorcluster, "Stop?"=w419:bool)  [unwired: 3 in, 4 out]
          }
          frame True {
            n78 = for "For循环" {
              N: w427 -> [_]
              tunnel: w434 -> [w446]
              tunnel: [w455] -> w433
              tunnel: w432 -> [w452]
              tunnel: [w453] -> w431
              tunnel: w430 -> [w442]
              tunnel: w428 -> [w449]
              tunnel: w429 -> [w450]
              shift-right: [w438] -> w426
              shift-left: w425 -> [_]
              tunnel: w424 -> [_]
              tunnel: w423 -> [w435]
              i -> [w436]
              stop <- w454 stop-if-true
              n79 = case shown="\"Slot1\", 默认" w442 {
                tunnel: [w473 w476] -> w439
                tunnel: [w474 w475] -> w443
                frame "Slot1", Default {
                  n80 = global read "GlobalValue.vi" "Slot1USBCOM"() -> (w473:refnum<visa-resource-name>)
                  n81 = global read "GlobalValue.vi" "Slot1USB"() -> (w474:string)
                }
                frame "Slot2" {
                  n82 = global read "GlobalValue.vi" "Slot2USBCOM"() -> (w476:refnum<visa-resource-name>)
                  n83 = global read "GlobalValue.vi" "Slot2USB"() -> (w475:string)
                }
              }
              n84 = Empty String/Path?(string/path=w439) -> (empty?=w444:bool)
              n85 = case shown="真" w444 {
                tunnel: [w470 w472] -> w441
                tunnel: w443 -> [_ w471]
                tunnel: w439 -> [w470 _]
                frame False {
                }
                frame True {
                  n86 = call "SearchUSB_CF.vi"("USB"=w471) -> ("USBPort"=w472:refnum<visa-resource-name>)  [unwired: 9 in, 1 out]
                }
              }
              n87 = case shown="1, 默认" w436 {
                tunnel: w446 -> [w456 w461]
                tunnel: [w456 w460] -> w445
                tunnel: w441 -> [_ w459]
                tunnel: string[] ["H330打开音频回环", "H330打开音频回环", "H330打开音频回环增益", "H330打开音频回环增益"] -> [_ w458]
                tunnel: w435 -> [_ w457]
                frame 0 {
                }
                frame 1, Default {
                  n88 = for {
                    tunnel: w459 -> [w467]
                    shift-right: [w468] -> w460
                    shift-left: w461 -> [w469]
                    tunnel: w458 -> [w464] mode=indexing
                    tunnel: w457 -> [w462]
                    n89 = Wait (ms)(milliseconds to wait=u32 50 ("等待时间（毫秒）")) -> ()  [unwired: 1 out]
                    n90 = call "SIMCOMCommunicationTool_CF.vi"("VISA资源名称"=w467, "MSComm"=w462, "通信协议名称"=w464, "DelayTime"=u32 100, "error in"=w469, "Debug"=FALSE) -> ("error out"=w468:errorcluster)  [unwired: 5 in, 4 out]
                  }
                }
              }
              n91 = Build Array(w450) -> (w448:string[])
              n92 = call "AIs-Freq.vi"("Slot"=w442, "error in"=w445, "Mode"=w449, "CHs"=w448) -> ("error out"=w451:errorcluster, "波形图"=w447:waveform(dbl)[])  [unwired: 5 in, 1 out]
              n93 = Index Array(array=w447) -> (element=w438:waveform(dbl))  [unwired: 1 in]
              n94 = call-poly <vilib>:"Extract Single Tone Information.vi"("time signal in"=w438) -> ("detected amplitude"=w437:dbl)  [unwired: 5 in, 5 out]
              n95 = call "TableHandle.vi"("All"=w452, "error in (no error)"=w451, "DataIn"=w437) -> ("error out"=w455:errorcluster, "Stop?"=w453:bool, "StopForLoop"=w454:bool)  [unwired: 4 in, 2 out]
            }
          }
        }
      }
      frame "AudioLoopBack_CF_VB" {
        n96 = case shown="真" w490 {
          tunnel: w493 -> [w497 w509]
          tunnel: w492 -> [w498 w511]
          tunnel: [w499 w510] -> w491
          tunnel: [w496 w508] -> w489
          tunnel: w488 -> [_ w507]
          tunnel: w487 -> [_ w506]
          tunnel: w486 -> [_ w505]
          tunnel: w485 -> [_ w504]
          tunnel: [w494 w503] -> w484
          tunnel: w483 -> [w494 w502]
          tunnel: w481 -> [_ w501]
          tunnel: w477 -> [_ w500]
          frame False {
            n97 = call "TableHandle.vi"("All"=w497, "error in (no error)"=w498, "DataIn"=TRUE) -> ("error out"=w499:errorcluster, "Stop?"=w496:bool)  [unwired: 3 in, 4 out]
          }
          frame True {
            n98 = for "For循环" {
              N: w504 -> [_]
              tunnel: w511 -> [w523]
              tunnel: [w532] -> w510
              tunnel: w509 -> [w529]
              tunnel: [w530] -> w508
              tunnel: w507 -> [w519]
              tunnel: w505 -> [w526]
              tunnel: w506 -> [w527]
              shift-right: [w515] -> w503
              shift-left: w502 -> [_]
              tunnel: w501 -> [_]
              tunnel: w500 -> [w512]
              i -> [w513]
              stop <- w531 stop-if-true
              n99 = case shown="\"Slot1\", 默认" w519 {
                tunnel: [w550 w553] -> w516
                tunnel: [w551 w552] -> w520
                frame "Slot1", Default {
                  n100 = global read "GlobalValue.vi" "Slot1USBCOM"() -> (w550:refnum<visa-resource-name>)
                  n101 = global read "GlobalValue.vi" "Slot1USB"() -> (w551:string)
                }
                frame "Slot2" {
                  n102 = global read "GlobalValue.vi" "Slot2USBCOM"() -> (w553:refnum<visa-resource-name>)
                  n103 = global read "GlobalValue.vi" "Slot2USB"() -> (w552:string)
                }
              }
              n104 = Empty String/Path?(string/path=w516) -> (empty?=w521:bool)
              n105 = case shown="真" w521 {
                tunnel: [w547 w549] -> w518
                tunnel: w520 -> [_ w548]
                tunnel: w516 -> [w547 _]
                frame False {
                }
                frame True {
                  n106 = call "SearchUSB_CF.vi"("USB"=w548) -> ("USBPort"=w549:refnum<visa-resource-name>)  [unwired: 9 in, 1 out]
                }
              }
              n107 = case shown="1, 默认" w513 {
                tunnel: w523 -> [w533 w538]
                tunnel: [w533 w537] -> w522
                tunnel: w518 -> [_ w536]
                tunnel: string[] ["H330打开音频回环", "H330打开音频回环", "H330打开音频回环增益", "H330打开音频回环增益"] -> [_ w535]
                tunnel: w512 -> [_ w534]
                frame 0 {
                }
                frame 1, Default {
                  n108 = for {
                    tunnel: w536 -> [w544]
                    shift-right: [w545] -> w537
                    shift-left: w538 -> [w546]
                    tunnel: w535 -> [w541] mode=indexing
                    tunnel: w534 -> [w539]
                    n109 = Wait (ms)(milliseconds to wait=u32 50 ("等待时间（毫秒）")) -> ()  [unwired: 1 out]
                    n110 = call "SIMCOMCommunicationTool_CF_vb.vi"("VISA资源名称"=w544, "MSComm"=w539, "通信协议名称"=w541, "DelayTime"=u32 100, "error in"=w546, "Debug"=FALSE) -> ("error out"=w545:errorcluster)  [unwired: 5 in, 4 out]
                  }
                }
              }
              n111 = Build Array(w527) -> (w525:string[])
              n112 = call "AIs-Freq.vi"("Slot"=w519, "error in"=w522, "Mode"=w526, "CHs"=w525) -> ("error out"=w528:errorcluster, "波形图"=w524:waveform(dbl)[])  [unwired: 5 in, 1 out]
              n113 = Index Array(array=w524) -> (element=w515:waveform(dbl))  [unwired: 1 in]
              n114 = call-poly <vilib>:"Extract Single Tone Information.vi"("time signal in"=w515) -> ("detected amplitude"=w514:dbl)  [unwired: 5 in, 5 out]
              n115 = call "TableHandle.vi"("All"=w529, "error in (no error)"=w528, "DataIn"=w514) -> ("error out"=w532:errorcluster, "Stop?"=w530:bool, "StopForLoop"=w531:bool)  [unwired: 4 in, 2 out]
            }
          }
        }
      }
      frame "AudioLoopBack_JHCA" {
        n116 = case shown="真" w568 {
          tunnel: w571 -> [w575 w587]
          tunnel: w570 -> [w576 w589]
          tunnel: [w577 w588] -> w569
          tunnel: [w574 w586] -> w567
          tunnel: w566 -> [_ w585]
          tunnel: w565 -> [_ w584]
          tunnel: w564 -> [_ w583]
          tunnel: w563 -> [_ w582]
          tunnel: [w572 w581] -> w562
          tunnel: w561 -> [w572 w580]
          tunnel: w559 -> [_ w579]
          tunnel: w555 -> [_ _]
          tunnel: w554 -> [_ w578]
          frame False {
            n117 = call "TableHandle.vi"("All"=w575, "error in (no error)"=w576, "DataIn"=TRUE) -> ("error out"=w577:errorcluster, "Stop?"=w574:bool)  [unwired: 3 in, 4 out]
          }
          frame True {
            n118 = for "For循环" {
              N: w582 -> [_]
              tunnel: w589 -> [w600]
              tunnel: [w609] -> w588
              tunnel: w587 -> [w606]
              tunnel: [w607] -> w586
              tunnel: w585 -> [w591]
              tunnel: w583 -> [w603]
              tunnel: w584 -> [w604]
              shift-right: [w598] -> w581
              shift-left: w580 -> [_]
              tunnel: w579 -> [_]
              tunnel: w578 -> [w593]
              i -> [w596]
              stop <- w608 stop-if-true
              n119 = property class="Ring (严格)"(reference=w593) -> ("RingText.Text"=w592:string)  [unwired: 1 in, 2 out]
              n120 = case shown="\"Slot1\", 默认" w591 {
                tunnel: [w610 w611] -> w590
                frame "Slot1", Default {
                  n121 = global read "GlobalValue.vi" "Slot1COM"() -> (w610:refnum<visa-resource-name>)
                }
                frame "Slot2" {
                  n122 = global read "GlobalValue.vi" "Slot2COM"() -> (w611:refnum<visa-resource-name>)
                }
              }
              n123 = for {
                tunnel: string[] ["关闭测试回环", "启动测试回环Speak\n", "MIC_CTL输出低电平"] -> [w613] mode=indexing
                tunnel: [w612] -> w595 mode=indexing
                n124 = call <vilib>:"Trim Whitespace.vi"("string"=w613) -> ("trimmed string"=w612:string)  [unwired: 1 in]
              }
              n125 = case shown="1, 默认" w596 {
                tunnel: w600 -> [w614 w620]
                tunnel: [w614 w619] -> w599
                tunnel: w590 -> [_ w617]
                tunnel: w595 -> [_ w618]
                tunnel: w591 -> [_ w616]
                tunnel: w592 -> [_ w615]
                frame 0 {
                }
                frame 1, Default {
                  n126 = for {
                    shift-right: [w624] -> w619
                    shift-left: w620 -> [w626]
                    tunnel: w618 -> [w628] mode=indexing
                    tunnel: w617 -> [w627]
                    tunnel: w616 -> [w625]
                    tunnel: w615 -> [w621]
                    n127 = call "CommunicationTool-Ver1.vi"("VISA资源名称"=w627, "ModelNumber"=w621, "通信协议名称"=w628, "Slot"=w625, "DelayTime"=u32 2000 ("等待时间（毫秒）"), "error in"=w626, "Debug"=FALSE) -> ("error out"=w624:errorcluster)  [unwired: 3 in, 5 out]
                    n128 = Wait (ms)(milliseconds to wait=u32 50 ("等待时间（毫秒）")) -> ()  [unwired: 1 out]
                  }
                }
              }
              n129 = Build Array(w604) -> (w602:string[])
              n130 = call "AIs-Freq.vi"("Slot"=w591, "error in"=w599, "Mode"=w603, "CHs"=w602) -> ("error out"=w605:errorcluster, "波形图"=w601:waveform(dbl)[])  [unwired: 5 in, 1 out]
              n131 = Index Array(array=w601) -> (element=w598:waveform(dbl))  [unwired: 1 in]
              n132 = call-poly <vilib>:"Extract Single Tone Information.vi"("time signal in"=w598) -> ("detected amplitude"=w597:dbl)  [unwired: 5 in, 5 out]
              n133 = call "TableHandle.vi"("All"=w606, "error in (no error)"=w605, "DataIn"=w597) -> ("error out"=w609:errorcluster, "Stop?"=w607:bool, "StopForLoop"=w608:bool)  [unwired: 4 in, 2 out]
            }
          }
        }
      }
      frame "AudioLoopBack_JHCA_N_A" {
        n134 = case shown="真" w646 {
          tunnel: w649 -> [w654 w669]
          tunnel: w648 -> [w655 w671]
          tunnel: [w656 w670] -> w647
          tunnel: [w653 w668] -> w645
          tunnel: w644 -> [_ w667]
          tunnel: w643 -> [_ w666]
          tunnel: w642 -> [_ w665]
          tunnel: w641 -> [_ w664]
          tunnel: [w651 w663] -> w640
          tunnel: w639 -> [w651 w662]
          tunnel: w637 -> [_ w661]
          tunnel: w634 -> [_ _]
          tunnel: w633 -> [_ w660]
          tunnel: w632 -> [w650 w659]
          tunnel: w631 -> [_ w658]
          tunnel: [w650 w657] -> w630
          frame False {
            n135 = call "TableHandle.vi"("All"=w654, "error in (no error)"=w655, "DataIn"=TRUE) -> ("error out"=w656:errorcluster, "Stop?"=w653:bool)  [unwired: 3 in, 4 out]
          }
          frame True {
            n136 = for "For循环" {
              N: w664 -> [_]
              tunnel: w671 -> [w692]
              tunnel: [w700] -> w670
              tunnel: w669 -> [w697]
              tunnel: [w698] -> w668
              tunnel: w667 -> [w684]
              tunnel: w665 -> [w695]
              tunnel: w666 -> [w681]
              shift-right: [w690] -> w663
              shift-left: w662 -> [_]
              tunnel: w661 -> [_]
              tunnel: w660 -> [w686]
              shift-right: [w672] -> w657
              shift-left: w659 -> [w676]
              tunnel: w658 -> [w673]
              i -> [w689]
              stop <- w699 stop-if-true
              n137 = property class="Ring (严格)"(reference=w686) -> ("RingText.Text"=w685:string)  [unwired: 1 in, 2 out]
              n138 = case shown="\"Slot1\", 默认" w684 {
                tunnel: [w701 w702] -> w683
                frame "Slot1", Default {
                  n139 = global read "GlobalValue.vi" "Slot1COM"() -> (w701:refnum<visa-resource-name>)
                }
                frame "Slot2" {
                  n140 = global read "GlobalValue.vi" "Slot2COM"() -> (w702:refnum<visa-resource-name>)
                }
              }
              n141 = call "StrDimantle.vi"("StrIn"=w681) -> ("上限值"=w677:dbl, "下限值"=w678:dbl, "循环次数"=w679:i32, "Audio"=w680:string)  [unwired: 7 in]
              n142 = for {
                tunnel: string[] ["关闭测试回环", "MIC_CTL输出高电平\n", "启动测试回环Aux", "MIC_CTL输出低电平"] -> [w704] mode=indexing
                tunnel: [w703] -> w688 mode=indexing
                n143 = call <vilib>:"Trim Whitespace.vi"("string"=w704) -> ("trimmed string"=w703:string)  [unwired: 1 in]
              }
              n144 = case shown="1, 默认" w689 {
                tunnel: w692 -> [w705 w711]
                tunnel: [w705 w710] -> w691
                tunnel: w683 -> [_ w708]
                tunnel: w688 -> [_ w709]
                tunnel: w684 -> [_ w707]
                tunnel: w685 -> [_ w706]
                frame 0 {
                }
                frame 1, Default {
                  n145 = for {
                    shift-right: [w715] -> w710
                    shift-left: w711 -> [w717]
                    tunnel: w709 -> [w719] mode=indexing
                    tunnel: w708 -> [w718]
                    tunnel: w707 -> [w716]
                    tunnel: w706 -> [w712]
                    n146 = call "CommunicationTool-Ver1.vi"("VISA资源名称"=w718, "ModelNumber"=w712, "通信协议名称"=w719, "Slot"=w716, "DelayTime"=u32 2000 ("等待时间（毫秒）"), "error in"=w717, "Debug"=FALSE) -> ("error out"=w715:errorcluster)  [unwired: 3 in, 5 out]
                    n147 = Wait (ms)(milliseconds to wait=u32 50 ("等待时间（毫秒）")) -> ()  [unwired: 1 out]
                  }
                }
              }
              n148 = Build Array(w680) -> (w694:string[])
              n149 = call "AIs-Freq_CA.vi"("下限值"=w678, "Slot"=w684, "上限值"=w677, "error in"=w691, "循环次数"=w679, "Mode"=w695, "CHs"=w694) -> ("error out"=w696:errorcluster, "幅值"=w682:dbl, "波形图"=w693:waveform(dbl)[], "Strout"=w675:string)  [unwired: 1 out]
              n150 = Concatenate Strings(w676, w675) -> (w672:string)
              n151 = Index Array(array=w693) -> (element=w690:waveform(dbl))  [unwired: 1 in]
              n152 = String Length(string=w672) -> (length=w674:i32)
              n153 = property class="Str"(reference=w673, "Text.Text"=w672, "Text.Scroll Position"=w674) -> ()  [unwired: 1 in, 2 out]
              n154 = call "TableHandle.vi"("All"=w697, "error in (no error)"=w696, "DataIn"=w682) -> ("error out"=w700:errorcluster, "Stop?"=w698:bool, "StopForLoop"=w699:bool)  [unwired: 4 in, 2 out]
            }
          }
        }
      }
      frame "AudioLoopBack_JHCA_N" {
        n155 = case shown="真" w737 {
          tunnel: w740 -> [w745 w760]
          tunnel: w739 -> [w746 w762]
          tunnel: [w747 w761] -> w738
          tunnel: [w744 w759] -> w736
          tunnel: w735 -> [_ w758]
          tunnel: w734 -> [_ w757]
          tunnel: w733 -> [_ w756]
          tunnel: w732 -> [_ w755]
          tunnel: [w742 w754] -> w731
          tunnel: w730 -> [w742 w753]
          tunnel: w728 -> [_ w752]
          tunnel: w725 -> [_ _]
          tunnel: w724 -> [_ w751]
          tunnel: w723 -> [w741 w750]
          tunnel: w722 -> [_ w749]
          tunnel: [w741 w748] -> w721
          frame False {
            n156 = call "TableHandle.vi"("All"=w745, "error in (no error)"=w746, "DataIn"=TRUE) -> ("error out"=w747:errorcluster, "Stop?"=w744:bool)  [unwired: 3 in, 4 out]
          }
          frame True {
            n157 = for "For循环" {
              N: w755 -> [_]
              tunnel: w762 -> [w783]
              tunnel: [w791] -> w761
              tunnel: w760 -> [w788]
              tunnel: [w789] -> w759
              tunnel: w758 -> [w775]
              tunnel: w756 -> [w786]
              tunnel: w757 -> [w772]
              shift-right: [w781] -> w754
              shift-left: w753 -> [_]
              tunnel: w752 -> [_]
              tunnel: w751 -> [w777]
              shift-right: [w763] -> w748
              shift-left: w750 -> [w767]
              tunnel: w749 -> [w764]
              i -> [w780]
              stop <- w790 stop-if-true
              n158 = property class="Ring (严格)"(reference=w777) -> ("RingText.Text"=w776:string)  [unwired: 1 in, 2 out]
              n159 = case shown="\"Slot1\", 默认" w775 {
                tunnel: [w792 w793] -> w774
                frame "Slot1", Default {
                  n160 = global read "GlobalValue.vi" "Slot1COM"() -> (w792:refnum<visa-resource-name>)
                }
                frame "Slot2" {
                  n161 = global read "GlobalValue.vi" "Slot2COM"() -> (w793:refnum<visa-resource-name>)
                }
              }
              n162 = call "StrDimantle.vi"("StrIn"=w772) -> ("上限值"=w768:dbl, "下限值"=w769:dbl, "循环次数"=w770:i32, "Audio"=w771:string)  [unwired: 7 in]
              n163 = for {
                tunnel: string[] ["关闭测试回环", "MIC_CTL输出高电平\n", "启动测试回环Speak", "MIC_CTL输出低电平"] -> [w795] mode=indexing
                tunnel: [w794] -> w779 mode=indexing
                n164 = call <vilib>:"Trim Whitespace.vi"("string"=w795) -> ("trimmed string"=w794:string)  [unwired: 1 in]
              }
              n165 = case shown="1, 默认" w780 {
                tunnel: w783 -> [w796 w802]
                tunnel: [w796 w801] -> w782
                tunnel: w774 -> [_ w799]
                tunnel: w779 -> [_ w800]
                tunnel: w775 -> [_ w798]
                tunnel: w776 -> [_ w797]
                frame 0 {
                }
                frame 1, Default {
                  n166 = for {
                    shift-right: [w806] -> w801
                    shift-left: w802 -> [w808]
                    tunnel: w800 -> [w810] mode=indexing
                    tunnel: w799 -> [w809]
                    tunnel: w798 -> [w807]
                    tunnel: w797 -> [w803]
                    n167 = call "CommunicationTool-Ver1.vi"("VISA资源名称"=w809, "ModelNumber"=w803, "通信协议名称"=w810, "Slot"=w807, "DelayTime"=u32 2000 ("等待时间（毫秒）"), "error in"=w808, "Debug"=FALSE) -> ("error out"=w806:errorcluster)  [unwired: 3 in, 5 out]
                    n168 = Wait (ms)(milliseconds to wait=u32 50 ("等待时间（毫秒）")) -> ()  [unwired: 1 out]
                  }
                }
              }
              n169 = Build Array(w771) -> (w785:string[])
              n170 = call "AIs-Freq_CA.vi"("下限值"=w769, "Slot"=w775, "上限值"=w768, "error in"=w782, "循环次数"=w770, "Mode"=w786, "CHs"=w785) -> ("error out"=w787:errorcluster, "幅值"=w773:dbl, "波形图"=w784:waveform(dbl)[], "Strout"=w766:string)  [unwired: 1 out]
              n171 = Concatenate Strings(w767, w766) -> (w763:string)
              n172 = Index Array(array=w784) -> (element=w781:waveform(dbl))  [unwired: 1 in]
              n173 = String Length(string=w763) -> (length=w765:i32)
              n174 = property class="Str"(reference=w764, "Text.Text"=w763, "Text.Scroll Position"=w765) -> ()  [unwired: 1 in, 2 out]
              n175 = call "TableHandle.vi"("All"=w788, "error in (no error)"=w787, "DataIn"=w773) -> ("error out"=w791:errorcluster, "Stop?"=w789:bool, "StopForLoop"=w790:bool)  [unwired: 4 in, 2 out]
            }
          }
        }
      }
      frame "AutoRecord" {
        n176 = case shown="真" w824 {
          tunnel: w827 -> [w831 w842]
          tunnel: w826 -> [w832 w844]
          tunnel: [w833 w843] -> w825
          tunnel: [w830 w841] -> w823
          tunnel: w822 -> [_ w840]
          tunnel: w821 -> [_ w839]
          tunnel: w820 -> [_ w838]
          tunnel: w819 -> [_ w837]
          tunnel: w814 -> [w828 w836]
          tunnel: w813 -> [_ w835]
          tunnel: [w828 w834] -> w812
          frame False {
            n177 = call "TableHandle.vi"("All"=w831, "error in (no error)"=w832, "DataIn"=TRUE) -> ("error out"=w833:errorcluster, "Stop?"=w830:bool)  [unwired: 3 in, 4 out]
          }
          frame True {
            n178 = for "For循环" {
              N: w837 -> [_]
              tunnel: w844 -> [w859]
              tunnel: [w863] -> w843
              tunnel: w842 -> [w860]
              tunnel: [w861] -> w841
              tunnel: w840 -> [w856]
              tunnel: w838 -> [w851]
              tunnel: w839 -> [_]
              shift-right: [w846] -> w834
              shift-left: w836 -> [w852]
              tunnel: w835 -> [w848]
              stop <- w862 stop-if-true
              n179 = Decimal String To Number(string=w851) -> (number=w850:i32)  [unwired: 2 in, 1 out]
              n180 = call "ccidinfo-r.vi"("Data Type"=PDINFO."WiFiName", "Slot"=w856) -> ("Data"=w855:string)
              n181 = call "ccidinfo-r.vi"("Data Type"=PDINFO."WiFiPassword", "Slot"=w856) -> ("Data"=w854:string)
              n182 = call "web.vi"("error in"=w859, "Password"=w854, "Delay"=w850, "WIFIName"=w855) -> ("错误输出"=w845:errorcluster, "TotalOut"=w849:string, "PASS？"=w853:bool)  [unwired: 4 in, 1 out]
              n183 = Concatenate Strings(w852, w849) -> (w846:string)
              n184 = String Length(string=w846) -> (length=w847:i32)
              n185 = property class="Str"(reference=w848, "Text.Text"=w846, "Text.Scroll Position"=w847) -> ()  [unwired: 1 in, 2 out]
              n186 = call "TableHandle.vi"("All"=w860, "error in (no error)"=w845, "DataIn"=w853) -> ("error out"=w863:errorcluster, "Stop?"=w861:bool, "StopForLoop"=w862:bool)  [unwired: 4 in, 2 out]
            }
          }
        }
      }
      frame "CANReceive" {
        n187 = case shown="真" w876 {
          tunnel: w879 -> [w883 w894]
          tunnel: w878 -> [w884 w896]
          tunnel: [w885 w895] -> w877
          tunnel: [w882 w893] -> w875
          tunnel: w874 -> [_ w886]
          tunnel: w873 -> [_ w887]
          tunnel: w872 -> [_ w892]
          tunnel: w871 -> [_ w891]
          tunnel: w868 -> [_ w890]
          tunnel: [w880 w889] -> w867
          tunnel: w866 -> [w880 w888]
          frame False {
            n188 = call "TableHandle.vi"("All"=w883, "error in (no error)"=w884, "DataIn"=TRUE) -> ("error out"=w885:errorcluster, "Stop?"=w882:bool)  [unwired: 3 in, 4 out]
          }
          frame True {
            n189 = for "For循环" {
              N: w891 -> [_]
              tunnel: w896 -> [w902]
              tunnel: [w913] -> w895
              tunnel: w894 -> [w910]
              tunnel: [w911] -> w893
              tunnel: w892 -> [w897]
              tunnel: w887 -> [w899]
              tunnel: w890 -> [w909]
              shift-right: [w907] -> w889
              shift-left: w888 -> [w908]
              tunnel: w886 -> [w905]
              stop <- w912 stop-if-true
              n190 = case shown="\"Slot2\"" w905 {
                tunnel: [u32 0 ("CANChannel") u32 1 ("CANChannel")] -> w904
                frame "Slot1", Default {
                }
                frame "Slot2" {
                }
              }
              n191 = call "Clear-Receive.vi"("错误输入"=w902, "CANChannel"=w904) -> ("错误输出"=w903:errorcluster)  [unwired: 2 in, 7 out]
              n192 = Concatenate Strings(w908, "CAN接收:" ("字符串"), "ID:" ("字符串"), w899, "DATA:" ("字符串"), w897) -> (w907:string)
              n193 = String Length(string=w907) -> (length=w906:i32)
              n194 = call "TableHandle.vi"("All"=w910, "error in (no error)"=w903) -> ("error out"=w913:errorcluster, "Stop?"=w911:bool, "StopForLoop"=w912:bool)  [unwired: 5 in, 2 out]
              n195 = property class="Str"(reference=w909, "Text.Text"=w907, "Text.Scroll Position"=w906) -> ()  [unwired: 1 in, 2 out]
            }
          }
        }
      }
      frame "CANTest" {
        n196 = case shown="真" w928 {
          tunnel: w931 -> [w935 w946]
          tunnel: w930 -> [w936 w948]
          tunnel: [w937 w947] -> w929
          tunnel: [w934 w945] -> w927
          tunnel: w926 -> [_ w938]
          tunnel: w925 -> [_ w939]
          tunnel: w924 -> [_ w944]
          tunnel: w923 -> [_ w943]
          tunnel: w920 -> [_ w942]
          tunnel: [w932 w941] -> w919
          tunnel: w918 -> [w932 w940]
          frame False {
            n197 = call "TableHandle.vi"("All"=w935, "error in (no error)"=w936, "DataIn"=TRUE) -> ("error out"=w937:errorcluster, "Stop?"=w934:bool)  [unwired: 3 in, 4 out]
          }
          frame True {
            n198 = for "For循环" {
              N: w943 -> [_]
              tunnel: w948 -> [w958]
              tunnel: [w972] -> w947
              tunnel: w946 -> [w969]
              tunnel: [w970] -> w945
              tunnel: w944 -> [w959]
              tunnel: w939 -> [w961]
              tunnel: w942 -> [w968]
              shift-right: [w966] -> w941
              shift-left: w940 -> [w967]
              tunnel: w938 -> [w964]
              stop <- w971 stop-if-true
              w949 = "\r\n"
              n199 = call "WaitTimes.vi"("WaitTimes"=u32 1000, "error in (no error)"=w958) -> ("error out"=w956:errorcluster)  [unwired: 9 in]
              n200 = case shown="\"Slot2\"" w964 {
                tunnel: [u32 0 ("CANChannel") u32 1 ("CANChannel")] -> w955
                frame "Slot1", Default {
                }
                frame "Slot2" {
                }
              }
              n201 = call "CANTEST.vi"("Data Input(Hex)"=w959, "错误输入"=w956, "ID(Hex 高位有效)"=w961, "CANChannel"=w955) -> ("错误输出"=w954:errorcluster, "ErrorSource"=w950:string, "帧数据"=w952:string)  [unwired: 5 in]
              n202 = Concatenate Strings(w967, "CAN发送:" ("字符串"), "ID:" ("字符串"), w961, "DATA:" ("字符串"), w959, w949, "CAN接收:" ("字符串"), w952, w949, "错误报告:" ("字符串"), w950, w949) -> (w966:string)
              n203 = String Length(string=w966) -> (length=w965:i32)
              n204 = call "TableHandle.vi"("All"=w969, "error in (no error)"=w954, "DataIn"=w952) -> ("error out"=w972:errorcluster, "Stop?"=w970:bool, "StopForLoop"=w971:bool)  [unwired: 4 in, 2 out]
              n205 = property class="Str"(reference=w968, "Text.Text"=w966, "Text.Scroll Position"=w965) -> ()  [unwired: 1 in, 2 out]
            }
          }
        }
      }
      frame "CANTransmit" {
        n206 = case shown="真" w987 {
          tunnel: w990 -> [w994 w1005]
          tunnel: w989 -> [w995 w1007]
          tunnel: [w996 w1006] -> w988
          tunnel: [w993 w1004] -> w986
          tunnel: w985 -> [_ w997]
          tunnel: w984 -> [_ w998]
          tunnel: w983 -> [_ w1003]
          tunnel: w982 -> [_ w1002]
          tunnel: w979 -> [_ w1001]
          tunnel: [w991 w1000] -> w978
          tunnel: w977 -> [w991 w999]
          frame False {
            n207 = call "TableHandle.vi"("All"=w994, "error in (no error)"=w995, "DataIn"=TRUE) -> ("error out"=w996:errorcluster, "Stop?"=w993:bool)  [unwired: 3 in, 4 out]
          }
          frame True {
            n208 = for "For循环" {
              N: w1002 -> [_]
              tunnel: w1007 -> [w1010]
              tunnel: [w1027] -> w1006
              tunnel: w1005 -> [w1024]
              tunnel: [w1025] -> w1004
              tunnel: w1003 -> [w1011]
              tunnel: w998 -> [w1013]
              tunnel: w1001 -> [w1023]
              shift-right: [w1021] -> w1000
              shift-left: w999 -> [w1022]
              tunnel: w997 -> [w1019]
              stop <- w1026 stop-if-true
              n209 = case shown="\"Slot2\"" w1019 {
                tunnel: [u32 0 ("CANChannel") u32 1 ("CANChannel")] -> w1018
                frame "Slot1", Default {
                }
                frame "Slot2" {
                }
              }
              n210 = call "WaitTimes.vi"("WaitTimes"=u32 1000, "error in (no error)"=w1010) -> ("error out"=w1008:errorcluster)  [unwired: 9 in]
              n211 = Concatenate Strings(w1022, "CAN发送:" ("字符串"), "ID:" ("字符串"), w1013, "DATA:" ("字符串"), w1011) -> (w1021:string)
              n212 = call "T.vi"("Data Input(Hex)"=w1011, "错误输入（无错误）"=w1008, "ID(Hex 高位有效)"=w1013, "CANChannel"=w1018) -> ("错误输出"=w1017:errorcluster, "Result"=w1016:bool)  [unwired: 6 in]
              n213 = String Length(string=w1021) -> (length=w1020:i32)
              n214 = call "TableHandle.vi"("All"=w1024, "error in (no error)"=w1017, "DataIn"=w1016) -> ("error out"=w1027:errorcluster, "Stop?"=w1025:bool, "StopForLoop"=w1026:bool)  [unwired: 4 in, 2 out]
              n215 = property class="Str"(reference=w1023, "Text.Text"=w1021, "Text.Scroll Position"=w1020) -> ()  [unwired: 1 in, 2 out]
            }
          }
        }
      }
      frame "CMD" {
        n216 = case shown="真" w1045 {
          tunnel: w1048 -> [w1052 w1068]
          tunnel: w1047 -> [w1053 w1070]
          tunnel: [w1054 w1069] -> w1046
          tunnel: [w1051 w1067] -> w1044
          tunnel: w1043 -> [_ w1060]
          tunnel: w1042 -> [_ w1061]
          tunnel: w1041 -> [_ w1066]
          tunnel: w1040 -> [_ w1065]
          tunnel: w1037 -> [_ w1064]
          tunnel: [w1049 w1063] -> w1036
          tunnel: w1035 -> [w1049 w1062]
          tunnel: [w1049 w1059] -> w1033
          tunnel: w1032 -> [_ w1058]
          tunnel: w1031 -> [_ w1057]
          tunnel: w1030 -> [_ w1056]
          frame False {
            n217 = call "TableHandle.vi"("All"=w1052, "error in (no error)"=w1053, "DataIn"=TRUE) -> ("error out"=w1054:errorcluster, "Stop?"=w1051:bool)  [unwired: 3 in, 4 out]
          }
          frame True {
            n218 = property class="Ring (严格)"(reference=w1056) -> ("RingText.Text"=w1055:string)  [unwired: 1 in, 2 out]
            n219 = for "For循环" {
              N: w1065 -> [_]
              tunnel: w1070 -> [w1083]
              tunnel: [w1096] -> w1069
              tunnel: w1068 -> [w1093]
              tunnel: [w1094] -> w1067
              tunnel: w1066 -> [w1091]
              tunnel: w1061 -> [w1071]
              tunnel: w1064 -> [w1089]
              shift-right: [w1087] -> w1063
              shift-left: w1062 -> [w1088]
              tunnel: w1060 -> [w1073]
              tunnel: [w1071] -> w1059
              tunnel: w1058 -> [w1077]
              tunnel: w1057 -> [w1075]
              tunnel: w1055 -> [w1072]
              i -> [w1084]
              stop <- w1095 stop-if-true
              n220 = Decimal String To Number(string=w1091, default (0L)=u32 0 ("默认(0 I32)")) -> (number=w1081:u32)  [unwired: 1 in, 1 out]
              n221 = property class="Str"(reference=w1075) -> ("Value"=w1074:string)  [unwired: 1 in, 2 out]
              n222 = case shown="\"Slot2\"" w1073 {
                tunnel: [w1103 w1104] -> w1080
                frame "Slot1", Default {
                  n223 = global read "GlobalValue.vi" "Slot1COM"() -> (w1103:refnum<visa-resource-name>)
                }
                frame "Slot2" {
                  n224 = global read "GlobalValue.vi" "Slot2COM"() -> (w1104:refnum<visa-resource-name>)
                }
              }
              n225 = case shown="1, 默认" w1084 {
                tunnel: w1083 -> [w1105 w1108]
                tunnel: [w1105 w1107] -> w1082
                tunnel: w1081 -> [_ w1106]
                frame 0 {
                }
                frame 1, Default {
                  n226 = call "WaitTimes.vi"("WaitTimes"=w1106, "error in (no error)"=w1108) -> ("error out"=w1107:errorcluster)  [unwired: 9 in]
                }
              }
              n227 = call "CommunicationTool.vi"("VISA资源名称"=w1080, "SN"=w1074, "ModelNumber"=w1072, "通信协议名称"=w1071, "Slot"=w1073, "DelayTime"=w1081, "error in"=w1082, "Debug"=FALSE) -> ("字符串数值"=w1078:bool, "CMD"=w1079:string, "data"=w1076:string, "error out"=w1092:errorcluster)  [unwired: 2 in, 2 out]
              n228 = Concatenate Strings(w1088, w1079) -> (w1087:string)
              n229 = String Length(string=w1087) -> (length=w1086:i32)
              n230 = call "TableHandle.vi"("All"=w1093, "error in (no error)"=w1092, "字符串数值"=w1078, "DataIn"=w1076) -> ("error out"=w1096:errorcluster, "Stop?"=w1094:bool, "StopForLoop"=w1095:bool)  [unwired: 3 in, 2 out]
              n231 = case shown="\"查询版本\", \"查询版本(长丰)\"" w1071 {
                tunnel: w1077 -> [_ w1098 _]
                tunnel: w1076 -> [_ w1097 w1099]
                tunnel: w1073 -> [_ _ w1100]
                frame "假", Default {
                }
                frame "查询版本", "查询版本(长丰)" {
                  n232 = property class="Str"(reference=w1098, "Value"=w1097) -> ()  [unwired: 1 in, 2 out]
                }
                frame "查询CCID" {
                  n233 = case shown="\"Slot2\"" w1100 {
                    tunnel: w1099 -> [w1101 w1102]
                    frame "Slot1", Default {
                      n234 = global write "GlobalValue.vi" "Slot1CCID"(w1101) -> ()
                    }
                    frame "Slot2" {
                      n235 = global write "GlobalValue.vi" "Slot2CCID"(w1102) -> ()
                    }
                  }
                }
              }
              n236 = property class="Str"(reference=w1089, "Text.Text"=w1087, "Text.Scroll Position"=w1086) -> ()  [unwired: 1 in, 2 out]
            }
          }
        }
      }
      frame "CMD-CAN" {
        n237 = case shown="真" w1121 {
          tunnel: w1124 -> [w1128 w1139]
          tunnel: w1123 -> [w1129 w1141]
          tunnel: [w1130 w1140] -> w1122
          tunnel: [w1127 w1138] -> w1120
          tunnel: w1119 -> [_ w1131]
          tunnel: w1118 -> [_ w1132]
          tunnel: w1117 -> [_ w1137]
          tunnel: w1116 -> [_ w1136]
          tunnel: w1113 -> [_ w1135]
          tunnel: [w1125 w1134] -> w1112
          tunnel: w1111 -> [w1125 w1133]
          frame False {
            n238 = call "TableHandle.vi"("All"=w1128, "error in (no error)"=w1129, "DataIn"=TRUE) -> ("error out"=w1130:errorcluster, "Stop?"=w1127:bool)  [unwired: 3 in, 4 out]
          }
          frame True {
            n239 = for "For循环" {
              N: w1136 -> [_]
              tunnel: w1141 -> [w1174]
              tunnel: [w1186] -> w1140
              tunnel: w1139 -> [w1183]
              tunnel: [w1184] -> w1138
              tunnel: w1137 -> [w1145]
              tunnel: w1132 -> [w1152]
              tunnel: w1135 -> [w1180]
              shift-right: [w1177] -> w1134
              shift-left: w1133 -> [w1179]
              tunnel: w1131 -> [w1173]
              i -> [w1175]
              stop <- w1185 stop-if-true
              w1156 = i16 2 ("宽度(-)")
              n240 = Match Pattern(string=w1145, regular expression=";" ("正则表达式")) -> (before substring=w1143:string, after substring=w1142:string)  [unwired: 1 in, 2 out]
              n241 = Decimal String To Number(string=w1142, default (0L)=u32 0 ("默认(0 I32)")) -> (number=w1150:u32)  [unwired: 1 in, 1 out]
              n242 = case shown="\"Slot1\", 默认" w1173 {
                tunnel: [w1207 w1208] -> w1153
                frame "Slot1", Default {
                  n243 = global read "GlobalValue.vi" "Slot1COM"() -> (w1207:refnum<visa-resource-name>)
                }
                frame "Slot2" {
                  n244 = global read "GlobalValue.vi" "Slot2COM"() -> (w1208:refnum<visa-resource-name>)
                }
              }
              n245 = case shown="1, 默认" w1175 {
                tunnel: w1174 -> [w1209 w1212]
                tunnel: [w1209 w1211] -> w1149
                tunnel: w1150 -> [_ w1210]
                frame 0 {
                }
                frame 1, Default {
                  n246 = call "WaitTimes.vi"("WaitTimes"=w1210, "error in (no error)"=w1212) -> ("error out"=w1211:errorcluster)  [unwired: 9 in]
                }
              }
              n247 = case shown="\"Slot2\"" w1173 {
                tunnel: [u32 0 ("CANChannel") u32 1 ("CANChannel")] -> w1151
                frame "Slot1", Default {
                }
                frame "Slot2" {
                }
              }
              n248 = call "R.vi"("ID(Hex 高位有效)"=w1143, "通信协议名称"=w1152, "错误输入（无错误）"=w1149, "DelayTime"=w1150, "CANChannel"=w1151, "VISA资源名称"=w1153) -> ("错误输出"=w1147:errorcluster, "VCI_CAN_OBJ_R"=w1146:T8, "CMD"=w1148:string)  [unwired: 3 in]
              n249 = disable-structure shown="启用" {
                disable-tunnel: [w1188 w1195] -> w1154
                disable-tunnel: w1151 -> [w1187 _]
                disable-tunnel: w1146 -> [_ w1195]
                frame Disabled {
                  n250 = for {
                    N: 100 -> [_]
                    tunnel: w1187 -> [w1194]
                    tunnel: _ -> [w1193]
                    tunnel: [w1191] -> w1188
                    tunnel: [w1190] -> _
                    stop <- w1192 stop-if-true
                    n251 = call "Clear-Receive.vi"("错误输入"=w1193, "CANChannel"=w1194) -> ("错误输出"=w1190:errorcluster, "VCI_CAN_OBJ_R"=w1191:T8, "Result"=w1192:bool)  [unwired: 2 in, 5 out]
                  }
                }
                frame Enabled {
                }
              }
              n252 = disable-structure shown="禁用" {
                disable-tunnel: [w1202 w1203] -> w1182
                disable-tunnel: [w1201 w1204] -> w1178
                disable-tunnel: w1153 -> [w1199 _]
                disable-tunnel: w1152 -> [w1198 _]
                disable-tunnel: w1150 -> [w1197 _]
                disable-tunnel: w1149 -> [w1196 _]
                disable-tunnel: w1148 -> [_ w1204]
                disable-tunnel: w1147 -> [_ w1203]
                frame Disabled {
                  n253 = call "CommunicationTool.vi"("VISA资源名称"=w1199, "通信协议名称"=w1198, "DelayTime"=w1197, "error in"=w1196, "Debug"=FALSE) -> ("CMD"=w1201:string, "error out"=w1202:errorcluster)  [unwired: 5 in, 4 out]
                }
                frame Enabled {
                }
              }
              n254 = Concatenate Strings(w1179, w1178) -> (w1177:string)
              n255 = Unbundle By Name(w1154) -> ("Byte0"=w1171:u8, "Byte1"=w1172:u8, "Byte2"=w1170:u8, "Byte3"=w1169:u8, "Byte4"=w1168:u8, "Byte5"=w1167:u8, "Byte6"=w1166:u8, "Byte7"=w1165:u8)
              n256 = String Length(string=w1177) -> (length=w1176:i32)
              n257 = Number To Hexadecimal String(1:w1156, 2:w1171) -> (0:w1164:string)
              n258 = Number To Hexadecimal String(1:w1156, 2:w1172) -> (0:w1163:string)
              n259 = Number To Hexadecimal String(1:w1156, 2:w1170) -> (0:w1162:string)
              n260 = Number To Hexadecimal String(1:w1156, 2:w1169) -> (0:w1161:string)
              n261 = Number To Hexadecimal String(1:w1156, 2:w1168) -> (0:w1160:string)
              n262 = Number To Hexadecimal String(1:w1156, 2:w1167) -> (0:w1159:string)
              n263 = Number To Hexadecimal String(1:w1156, 2:w1166) -> (0:w1158:string)
              n264 = Number To Hexadecimal String(1:w1156, 2:w1165) -> (0:w1157:string)
              n265 = property class="Str"(reference=w1180, "Text.Text"=w1177, "Text.Scroll Position"=w1176) -> ()  [unwired: 1 in, 2 out]
              n266 = Concatenate Strings(w1164, w1163, w1162, w1161, w1160, w1159, w1158, w1157) -> (w1155:string)
              n267 = call "TableHandle.vi"("All"=w1183, "error in (no error)"=w1182, "DataIn"=w1155) -> ("error out"=w1186:errorcluster, "Stop?"=w1184:bool, "StopForLoop"=w1185:bool)  [unwired: 4 in, 2 out]
            }
          }
        }
      }
      frame "CMD_CF" {
        n268 = case shown="真" w1230 {
          tunnel: w1233 -> [w1237 w1255]
          tunnel: w1232 -> [w1238 w1257]
          tunnel: [w1239 w1256] -> w1231
          tunnel: [w1236 w1254] -> w1229
          tunnel: w1228 -> [_ w1247]
          tunnel: w1227 -> [_ w1248]
          tunnel: w1226 -> [_ w1253]
          tunnel: w1225 -> [_ w1252]
          tunnel: w1222 -> [_ w1251]
          tunnel: [w1234 w1250] -> w1221
          tunnel: w1220 -> [w1234 w1249]
          tunnel: [w1234 w1246] -> w1218
          tunnel: w1217 -> [_ w1245]
          tunnel: w1216 -> [_ w1244]
          tunnel: w1215 -> [_ w1243]
          tunnel: w1214 -> [_ w1241]
          tunnel: w1213 -> [_ w1240]
          frame False {
            n269 = call "TableHandle.vi"("All"=w1237, "error in (no error)"=w1238, "DataIn"=TRUE) -> ("error out"=w1239:errorcluster, "Stop?"=w1236:bool)  [unwired: 3 in, 4 out]
          }
          frame True {
            n270 = property class="Ring (严格)"(reference=w1243) -> ("RingText.Text"=w1242:string)  [unwired: 1 in, 2 out]
            n271 = for "For循环" {
              N: w1252 -> [_]
              tunnel: w1257 -> [w1278]
              tunnel: [w1290] -> w1256
              tunnel: w1255 -> [w1287]
              tunnel: [w1288] -> w1254
              tunnel: w1253 -> [w1286]
              tunnel: w1248 -> [w1268]
              tunnel: w1251 -> [w1284]
              shift-right: [w1282] -> w1250
              shift-left: w1249 -> [w1283]
              tunnel: w1247 -> [w1264]
              tunnel: [w1268] -> w1246
              tunnel: w1245 -> [w1272]
              tunnel: w1244 -> [w1270]
              tunnel: w1242 -> [w1261]
              tunnel: w1241 -> [w1267]
              tunnel: w1240 -> [w1266]
              i -> [w1279]
              stop <- w1289 stop-if-true
              n272 = Decimal String To Number(string=w1286, default (0L)=u32 0 ("默认(0 I32)")) -> (number=w1276:u32)  [unwired: 1 in, 1 out]
              n273 = property class="Str"(reference=w1270) -> ("Value"=w1269:string)  [unwired: 1 in, 2 out]
              n274 = case shown="\"Slot2\"" w1264 {
                tunnel: [w1323 w1324] -> w1275
                frame "Slot1", Default {
                  n275 = global read "GlobalValue.vi" "Slot1COM"() -> (w1323:refnum<visa-resource-name>)
                }
                frame "Slot2" {
                  n276 = global read "GlobalValue.vi" "Slot2COM"() -> (w1324:refnum<visa-resource-name>)
                }
              }
              n277 = case shown="1, 默认" w1279 {
                tunnel: w1278 -> [w1325 w1328]
                tunnel: [w1325 w1327] -> w1277
                tunnel: w1276 -> [_ w1326]
                frame 0 {
                }
                frame 1, Default {
                  n278 = call "WaitTimes.vi"("WaitTimes"=w1326, "error in (no error)"=w1328) -> ("error out"=w1327:errorcluster)  [unwired: 9 in]
                }
              }
              n279 = call "CommunicationTool-Ver1.vi"("VISA资源名称"=w1275, "SN"=w1269, "ModelNumber"=w1261, "通信协议名称"=w1268, "Slot"=w1264, "DelayTime"=w1276, "error in"=w1277, "Debug"=FALSE) -> ("字符串数值"=w1273:bool, "响应"=w1265:string, "CMD"=w1274:string, "data"=w1271:string, "error out"=w1263:errorcluster)  [unwired: 2 in, 1 out]
              n280 = case shown="\"写入WIFI名称\"" w1268 {
                tunnel: w1264 -> [_ w1304]
                tunnel: w1267 -> [_ w1303]
                tunnel: w1263 -> [w1299 w1302]
                tunnel: [w1299 w1301] -> w1258
                tunnel: w1266 -> [_ w1300]
                frame "假", Default {
                }
                frame "写入WIFI名称" {
                  n281 = case shown="\"Slot2\"" w1304 {
                    selector: w1304 -> [w1309 w1315]
                    tunnel: w1303 -> [w1308 _]
                    tunnel: w1302 -> [w1306 w1313]
                    tunnel: [w1305 w1312] -> w1301
                    tunnel: w1300 -> [_ w1311]
                    frame "Slot1", Default {
                      n282 = call "ccidinfo-r.vi"("Data Type"=PDINFO."WiFiName", "Slot"=w1309) -> ("Data"=w1307:string)
                      n283 = property class="Str"(reference=w1308, error in=w1306, "Value"=w1307) -> (error out=w1305:errorcluster)  [unwired: 1 out]
                    }
                    frame "Slot2" {
                      n284 = call "ccidinfo-r.vi"("Data Type"=PDINFO."WiFiName", "Slot"=w1315) -> ("Data"=w1314:string)
                      n285 = property class="Str"(reference=w1311, error in=w1313, "Value"=w1314) -> (error out=w1312:errorcluster)  [unwired: 1 out]
                    }
                  }
                }
              }
              n286 = case shown="\"1878\", \"1892\"" w1261 {
                tunnel: w1265 -> [_ w1297]
                tunnel: w1264 -> [_ w1296]
                tunnel: w1263 -> [w1291 w1295]
                tunnel: ["" w1294] -> w1262
                tunnel: [w1291 w1293] -> w1260
                frame "假", Default {
                }
                frame "1878", "1892" {
                  n287 = call "SpecialProcess.vi"("error in"=w1295, "Slot"=w1296, "StrIn"=w1297, "N"=2) -> ("error out"=w1293:errorcluster, "data"=w1294:string)  [unwired: 6 in]
                }
              }
              n288 = Concatenate Strings(w1283, w1274, w1262) -> (w1282:string)
              n289 = String Length(string=w1282) -> (length=w1281:i32)
              n290 = Merge Errors(w1260, w1258) -> (w1259:errorcluster)
              n291 = case shown="\"假\", 默认" w1268 {
                tunnel: w1272 -> [_ w1318 _]
                tunnel: w1271 -> [_ w1317 w1319]
                tunnel: w1264 -> [_ _ w1320]
                frame "假", Default {
                }
                frame "查询版本", "查询版本(长丰)" {
                  n292 = property class="Str"(reference=w1318, "Value"=w1317) -> ()  [unwired: 1 in, 2 out]
                }
                frame "查询CCID" {
                  n293 = case shown="\"Slot2\"" w1320 {
                    tunnel: w1319 -> [w1321 w1322]
                    frame "Slot1", Default {
                      n294 = global write "GlobalValue.vi" "Slot1CCID"(w1321) -> ()
                    }
                    frame "Slot2" {
                      n295 = global write "GlobalValue.vi" "Slot2CCID"(w1322) -> ()
                    }
                  }
                }
              }
              n296 = property class="Str"(reference=w1284, "Text.Text"=w1282, "Text.Scroll Position"=w1281) -> ()  [unwired: 1 in, 2 out]
              n297 = call "TableHandle.vi"("All"=w1287, "error in (no error)"=w1259, "字符串数值"=w1273, "DataIn"=w1271) -> ("error out"=w1290:errorcluster, "Stop?"=w1288:bool, "StopForLoop"=w1289:bool)  [unwired: 3 in, 2 out]
            }
          }
        }
      }
      frame "Check" {
        n298 = case shown="真" w1341 {
          tunnel: w1344 -> [w1348 w1359]
          tunnel: w1343 -> [w1349 w1361]
          tunnel: [w1350 w1360] -> w1342
          tunnel: [w1347 w1358] -> w1340
          tunnel: w1339 -> [_ w1357]
          tunnel: w1338 -> [_ w1356]
          tunnel: w1337 -> [_ w1355]
          tunnel: w1336 -> [_ w1354]
          tunnel: w1333 -> [_ w1353]
          tunnel: w1332 -> [w1345 w1352]
          tunnel: [w1345 w1351] -> w1331
          frame False {
            n299 = call "TableHandle.vi"("All"=w1348, "error in (no error)"=w1349, "DataIn"=TRUE) -> ("error out"=w1350:errorcluster, "Stop?"=w1347:bool)  [unwired: 3 in, 4 out]
          }
          frame True {
            n300 = for "For循环" {
              N: w1354 -> [_]
              tunnel: w1361 -> [w1367]
              tunnel: [w1374] -> w1360
              tunnel: w1359 -> [w1365]
              tunnel: [w1372] -> w1358
              tunnel: w1357 -> [_]
              tunnel: w1355 -> [_]
              tunnel: w1356 -> [w1364]
              tunnel: w1353 -> [w1370]
              shift-right: [w1368] -> w1351
              shift-left: w1352 -> [w1369]
              stop <- w1373 stop-if-true
              n301 = call "VisualCheckSubPanel.vi"("GuiRef"=w1365, "error in (no error)"=w1367, "测试项"=w1364) -> ("error out"=w1366:errorcluster, "StringOut"=w1362:string, "Result"=w1363:bool)  [unwired: 6 in]
              n302 = Concatenate Strings(w1369, w1362) -> (w1368:string)
              n303 = String Length(string=w1368) -> (length=w1371:i32)
              n304 = property class="Str"(reference=w1370, "Text.Text"=w1368, "Text.Scroll Position"=w1371) -> ()  [unwired: 1 in, 2 out]
              n305 = call "TableHandle.vi"("All"=w1365, "error in (no error)"=w1366, "DataIn"=w1363) -> ("error out"=w1374:errorcluster, "Stop?"=w1372:bool, "StopForLoop"=w1373:bool)  [unwired: 4 in, 2 out]
            }
          }
        }
      }
      frame "CheckDB" {
        n306 = case shown="真" w1389 {
          tunnel: w1392 -> [w1396 w1409]
          tunnel: w1391 -> [w1397 w1411]
          tunnel: [w1398 w1410] -> w1390
          tunnel: [w1395 w1408] -> w1388
          tunnel: w1387 -> [_ w1407]
          tunnel: w1386 -> [_ w1406]
          tunnel: w1385 -> [_ w1405]
          tunnel: w1384 -> [_ w1404]
          tunnel: w1381 -> [_ w1403]
          tunnel: w1380 -> [w1393 w1402]
          tunnel: [w1393 w1401] -> w1379
          tunnel: w1376 -> [_ w1400]
          tunnel: w1375 -> [_ w1399]
          frame False {
            n307 = call "TableHandle.vi"("All"=w1396, "error in (no error)"=w1397, "DataIn"=TRUE) -> ("error out"=w1398:errorcluster, "Stop?"=w1395:bool)  [unwired: 3 in, 4 out]
          }
          frame True {
            n308 = for "For循环" {
              N: w1404 -> [_]
              tunnel: w1411 -> [w1428]
              tunnel: [w1432] -> w1410
              tunnel: w1409 -> [w1429]
              tunnel: [w1430] -> w1408
              tunnel: w1407 -> [_]
              tunnel: w1405 -> [_]
              tunnel: w1406 -> [_]
              tunnel: w1403 -> [w1417]
              shift-right: [w1412] -> w1401
              shift-left: w1402 -> [w1416]
              tunnel: w1400 -> [w1425]
              tunnel: w1399 -> [w1423]
              stop <- w1431 stop-if-true
              w1420 = ","
              w1421 = "'"
              n309 = property class="Str"(reference=w1423) -> ("Value"=w1422:string)  [unwired: 1 in, 2 out]
              n310 = property class="Ring (严格)"(reference=w1425) -> ("RingText.Text"=w1424:string)  [unwired: 1 in, 2 out]
              n311 = Concatenate Strings(w1421, w1424, w1421, w1420, w1421, w1422, w1421, w1420, "@b") -> (w1418:string)
              n312 = call "WtriteDataTOCheckSNTab.vi"("error in"=w1428, "SQL"=w1418) -> ("error out"=w1427:errorcluster, "DataOut"=w1414:string)  [unwired: 8 in]
              n313 = Concatenate Strings(w1416, "短路检测结果：", w1414) -> (w1412:string)
              n314 = String Length(string=w1412) -> (length=w1413:i32)
              n315 = property class="Str"(reference=w1417, "Text.Text"=w1412, "Text.Scroll Position"=w1413) -> ()  [unwired: 1 in, 2 out]
              n316 = call "TableHandle.vi"("All"=w1429, "error in (no error)"=w1427, "字符串数值"=FALSE, "DataIn"=w1414) -> ("error out"=w1432:errorcluster, "Stop?"=w1430:bool, "StopForLoop"=w1431:bool)  [unwired: 3 in, 2 out]
            }
          }
        }
      }
      frame "CheckMEID" {
        n317 = case shown="真" w1445 {
          tunnel: w1448 -> [w1452 w1463]
          tunnel: w1447 -> [w1453 w1465]
          tunnel: [w1454 w1464] -> w1446
          tunnel: [w1451 w1462] -> w1444
          tunnel: w1443 -> [_ w1461]
          tunnel: w1442 -> [_ w1460]
          tunnel: w1441 -> [_ w1459]
          tunnel: w1440 -> [_ w1458]
          tunnel: w1439 -> [w1449 w1457]
          tunnel: [w1449 w1457] -> w1438
          tunnel: w1434 -> [_ w1456]
          tunnel: w1433 -> [_ w1455]
          frame False {
            n318 = call "TableHandle.vi"("All"=w1452, "error in (no error)"=w1453, "DataIn"=TRUE) -> ("error out"=w1454:errorcluster, "Stop?"=w1451:bool)  [unwired: 3 in, 4 out]
          }
          frame True {
            n319 = for "For循环" {
              N: w1458 -> [_]
              tunnel: w1465 -> [w1469]
              tunnel: [w1476] -> w1464
              tunnel: w1463 -> [w1473]
              tunnel: [w1474] -> w1462
              tunnel: w1461 -> [w1466]
              tunnel: w1459 -> [_]
              tunnel: w1460 -> [_]
              tunnel: w1457 -> [_]
              tunnel: w1456 -> [_]
              tunnel: w1455 -> [w1472]
              stop <- w1475 stop-if-true
              n320 = case shown="\"Slot2\"" w1466 {
                tunnel: ["左" ("消息") "右" ("消息")] -> w1467
                frame "Slot1", Default {
                }
                frame "Slot2" {
                }
              }
              n321 = global read "GlobalValue.vi" "Data"() -> (w1471:string[][])
              n322 = call "GetSimInfo.vi"("Slot"=w1466, "error in (no error)"=w1469, "MEID"=w1472, "Data"=w1471) -> ("error out"=w1470:errorcluster, "Result"=w1468:bool)  [unwired: 5 in, 1 out]
              n323 = case shown="假" w1468 {
                tunnel: w1467 -> [w1482 _]
                frame False {
                  n324 = Concatenate Strings("当前电信5码信息中不存在" ("消息"), w1482, "侧MEID" ("字符串")) -> (w1479:string)
                  n325 = One Button Dialog(message=w1479) -> ()  [unwired: 1 in, 1 out]
                }
                frame True {
                }
              }
              n326 = call "TableHandle.vi"("All"=w1473, "error in (no error)"=w1470, "DataIn"=w1468) -> ("error out"=w1476:errorcluster, "Stop?"=w1474:bool, "StopForLoop"=w1475:bool)  [unwired: 4 in, 2 out]
            }
          }
        }
      }
      frame "CheckSN" {
        n327 = case shown="真" w1495 {
          tunnel: w1498 -> [w1502 w1512]
          tunnel: w1497 -> [w1503 w1514]
          tunnel: [w1504 w1513] -> w1496
          tunnel: [w1501 w1511] -> w1494
          tunnel: w1493 -> [_ w1510]
          tunnel: w1492 -> [_ w1509]
          tunnel: w1491 -> [_ w1508]
          tunnel: w1490 -> [_ w1507]
          tunnel: w1489 -> [w1499 w1506]
          tunnel: [w1499 w1506] -> w1488
          tunnel: w1483 -> [_ w1505]
          frame False {
            n328 = call "TableHandle.vi"("All"=w1502, "error in (no error)"=w1503, "DataIn"=TRUE) -> ("error out"=w1504:errorcluster, "Stop?"=w1501:bool)  [unwired: 3 in, 4 out]
          }
          frame True {
            n329 = for "For循环" {
              N: w1507 -> [_]
              tunnel: w1514 -> [w1519]
              tunnel: [w1524] -> w1513
              tunnel: w1512 -> [w1521]
              tunnel: [w1522] -> w1511
              tunnel: w1510 -> [w1515]
              tunnel: w1508 -> [_]
              tunnel: w1509 -> [_]
              tunnel: w1506 -> [_]
              tunnel: w1505 -> [w1518]
              stop <- w1523 stop-if-true
              n330 = property class="Str"(reference=w1518) -> ("Value"=w1517:string)  [unwired: 1 in, 2 out]
              n331 = call "CheckSN.vi"("Slot"=w1515, "error out"=w1519, "SN"=w1517) -> ("错误输出"=w1520:errorcluster, "比对结果"=w1516:bool)  [unwired: 7 in]
              n332 = case shown="\"Slot1\", 默认" w1515 {
                tunnel: w1516 -> [w1525 w1526]
                frame "Slot1", Default {
                  n333 = global write "GlobalValue.vi" "SN1 Result"(w1525) -> ()
                }
                frame "Slot2" {
                  n334 = global write "GlobalValue.vi" "SN2 Result"(w1526) -> ()
                }
              }
              n335 = call "TableHandle.vi"("All"=w1521, "error in (no error)"=w1520, "DataIn"=w1516) -> ("error out"=w1524:errorcluster, "Stop?"=w1522:bool, "StopForLoop"=w1523:bool)  [unwired: 4 in, 2 out]
            }
          }
        }
      }
      frame "CheckWiFiName" {
        n336 = case shown="真" w1539 {
          tunnel: w1542 -> [w1546 w1556]
          tunnel: w1541 -> [w1547 w1558]
          tunnel: [w1548 w1557] -> w1540
          tunnel: [w1545 w1555] -> w1538
          tunnel: w1537 -> [_ w1554]
          tunnel: w1536 -> [_ w1553]
          tunnel: w1535 -> [_ w1552]
          tunnel: w1534 -> [_ w1551]
          tunnel: w1533 -> [w1543 w1550]
          tunnel: [w1543 w1550] -> w1532
          tunnel: w1527 -> [_ w1549]
          frame False {
            n337 = call "TableHandle.vi"("All"=w1546, "error in (no error)"=w1547, "DataIn"=TRUE) -> ("error out"=w1548:errorcluster, "Stop?"=w1545:bool)  [unwired: 3 in, 4 out]
          }
          frame True {
            n338 = for "For循环" {
              N: w1551 -> [_]
              tunnel: w1558 -> [w1563]
              tunnel: [w1568] -> w1557
              tunnel: w1556 -> [w1565]
              tunnel: [w1566] -> w1555
              tunnel: w1554 -> [w1559]
              tunnel: w1552 -> [_]
              tunnel: w1553 -> [_]
              tunnel: w1550 -> [_]
              tunnel: w1549 -> [_]
              stop <- w1567 stop-if-true
              n339 = call "ccidinfo-r.vi"("Data Type"=PDINFO."WiFiName", "Slot"=w1559) -> ("Data"=w1560:string)
              n340 = call "CheckWIFIName.vi"("Slot"=w1559, "error out"=w1563, "WIFI"=w1560) -> ("错误输出"=w1564:errorcluster, "比对结果"=w1562:bool)  [unwired: 6 in]
              n341 = call "TableHandle.vi"("All"=w1565, "error in (no error)"=w1564, "DataIn"=w1562) -> ("error out"=w1568:errorcluster, "Stop?"=w1566:bool, "StopForLoop"=w1567:bool)  [unwired: 4 in, 2 out]
            }
          }
        }
      }
      frame "ConnectWifi" {
        n342 = case shown="真" w1581 {
          tunnel: w1584 -> [w1588 w1598]
          tunnel: w1583 -> [w1589 w1600]
          tunnel: [w1590 w1599] -> w1582
          tunnel: [w1587 w1597] -> w1580
          tunnel: w1579 -> [_ w1596]
          tunnel: w1578 -> [_ w1595]
          tunnel: w1577 -> [_ w1594]
          tunnel: w1576 -> [_ w1593]
          tunnel: w1575 -> [w1585 w1592]
          tunnel: [w1585 w1592] -> w1574
          tunnel: w1569 -> [_ w1591]
          frame False {
            n343 = call "TableHandle.vi"("All"=w1588, "error in (no error)"=w1589, "DataIn"=TRUE) -> ("error out"=w1590:errorcluster, "Stop?"=w1587:bool)  [unwired: 3 in, 4 out]
          }
          frame True {
            n344 = for "For循环" {
              N: w1593 -> [_]
              tunnel: w1600 -> [w1605]
              tunnel: [w1610] -> w1599
              tunnel: w1598 -> [w1607]
              tunnel: [w1608] -> w1597
              tunnel: w1596 -> [w1601]
              tunnel: w1594 -> [_]
              tunnel: w1595 -> [_]
              tunnel: w1592 -> [_]
              tunnel: w1591 -> [_]
              stop <- w1609 stop-if-true
              n345 = call "ccidinfo-r.vi"("Data Type"=PDINFO."WiFiName", "Slot"=w1601) -> ("Data"=w1602:string)
              n346 = call "ConnectWifiMention.vi"("Slot"=w1601, "error out"=w1605, "WIFI"=w1602) -> ("错误输出"=w1606:errorcluster, "连接结果"=w1604:bool)  [unwired: 6 in]
              n347 = call "TableHandle.vi"("All"=w1607, "error in (no error)"=w1606, "DataIn"=w1604) -> ("error out"=w1610:errorcluster, "Stop?"=w1608:bool, "StopForLoop"=w1609:bool)  [unwired: 4 in, 2 out]
            }
          }
        }
      }
      frame "DIAction" {
        n348 = case shown="真" w1621 {
          tunnel: w1624 -> [w1627 w1635]
          tunnel: w1623 -> [w1628 w1637]
          tunnel: [w1629 w1636] -> w1622
          tunnel: [w1626 w1634] -> w1620
          tunnel: w1619 -> [_ w1633]
          tunnel: w1618 -> [_ w1632]
          tunnel: w1617 -> [_ w1631]
          tunnel: w1616 -> [_ w1630]
          frame False {
            n349 = call "TableHandle.vi"("All"=w1627, "error in (no error)"=w1628, "DataIn"=TRUE) -> ("error out"=w1629:errorcluster, "Stop?"=w1626:bool)  [unwired: 3 in, 4 out]
          }
          frame True {
            n350 = for "For循环" {
              N: w1630 -> [_]
              tunnel: w1637 -> [w1642]
              tunnel: [w1646] -> w1636
              tunnel: w1635 -> [w1643]
              tunnel: [w1644] -> w1634
              tunnel: w1633 -> [w1638]
              tunnel: w1631 -> [_]
              tunnel: w1632 -> [w1640]
              stop <- w1645 stop-if-true
              n351 = call "DIAction.vi"("Slot"=w1638, "error in"=w1642, "CH"=w1640) -> ("error out"=w1641:errorcluster, "Status"=w1639:bool)  [unwired: 7 in]
              n352 = call "TableHandle.vi"("All"=w1643, "error in (no error)"=w1641, "DataIn"=w1639) -> ("error out"=w1646:errorcluster, "Stop?"=w1644:bool, "StopForLoop"=w1645:bool)  [unwired: 4 in, 2 out]
            }
          }
        }
      }
      frame "DOAction" {
        n353 = case shown="真" w1657 {
          tunnel: w1660 -> [w1663 w1671]
          tunnel: w1659 -> [w1664 w1673]
          tunnel: [w1665 w1672] -> w1658
          tunnel: [w1662 w1670] -> w1656
          tunnel: w1655 -> [_ w1669]
          tunnel: w1654 -> [_ w1668]
          tunnel: w1653 -> [_ w1667]
          tunnel: w1652 -> [_ w1666]
          frame False {
            n354 = call "TableHandle.vi"("All"=w1663, "error in (no error)"=w1664, "DataIn"=TRUE) -> ("error out"=w1665:errorcluster, "Stop?"=w1662:bool)  [unwired: 3 in, 4 out]
          }
          frame True {
            n355 = for "For循环" {
              N: w1666 -> [_]
              tunnel: w1673 -> [w1679]
              tunnel: [w1683] -> w1672
              tunnel: w1671 -> [w1680]
              tunnel: [w1681] -> w1670
              tunnel: w1669 -> [w1674]
              tunnel: w1667 -> [w1676]
              tunnel: w1668 -> [w1677]
              stop <- w1682 stop-if-true
              n356 = call "DOAction.vi"("Slot"=w1674, "error in"=w1679, "State"=w1676, "CH"=w1677) -> ("error out"=w1678:errorcluster)  [unwired: 7 in]
              n357 = call "TableHandle.vi"("All"=w1680, "error in (no error)"=w1678, "DataIn"="Done") -> ("error out"=w1683:errorcluster, "Stop?"=w1681:bool, "StopForLoop"=w1682:bool)  [unwired: 4 in, 2 out]
            }
          }
        }
      }
      frame "Delay" {
        n358 = case shown="真" w1694 {
          tunnel: w1697 -> [w1700 w1708]
          tunnel: w1696 -> [w1701 w1710]
          tunnel: [w1702 w1709] -> w1695
          tunnel: [w1699 w1707] -> w1693
          tunnel: w1692 -> [_ w1706]
          tunnel: w1691 -> [_ w1705]
          tunnel: w1690 -> [_ w1704]
          tunnel: w1689 -> [_ w1703]
          frame False {
            n359 = call "TableHandle.vi"("All"=w1700, "error in (no error)"=w1701, "DataIn"=TRUE) -> ("error out"=w1702:errorcluster, "Stop?"=w1699:bool)  [unwired: 3 in, 4 out]
          }
          frame True {
            n360 = for "For循环" {
              N: w1703 -> [_]
              tunnel: w1710 -> [w1718]
              tunnel: [w1722] -> w1709
              tunnel: w1708 -> [w1719]
              tunnel: [w1720] -> w1707
              tunnel: w1706 -> [_]
              tunnel: w1704 -> [w1714]
              tunnel: w1705 -> [_]
              stop <- w1721 stop-if-true
              n361 = Fract/Exp String To Number(string=w1714) -> (number=w1713:dbl)  [unwired: 3 in, 1 out]
              n362 = Multiply(x=w1713, y=1000.0) -> (x*y=w1712:dbl)
              n363 = To Unsigned Long Integer(number=w1712) -> (unsigned 32bit integer=w1711:u32)
              n364 = call "WaitTimes.vi"("WaitTimes"=w1711, "error in (no error)"=w1718) -> ("error out"=w1717:errorcluster)  [unwired: 9 in]
              n365 = call "TableHandle.vi"("All"=w1719, "error in (no error)"=w1717, "DataIn"="Done") -> ("error out"=w1722:errorcluster, "Stop?"=w1720:bool, "StopForLoop"=w1721:bool)  [unwired: 4 in, 2 out]
            }
          }
        }
      }
      frame "E_CALL测试" {
        n366 = case shown="真" w1738 {
          tunnel: w1741 -> [w1745 w1761]
          tunnel: w1740 -> [w1746 w1763]
          tunnel: [w1747 w1762] -> w1739
          tunnel: [w1744 w1760] -> w1737
          tunnel: w1736 -> [_ w1753]
          tunnel: w1735 -> [_ w1754]
          tunnel: w1734 -> [_ w1759]
          tunnel: w1733 -> [_ w1758]
          tunnel: w1730 -> [_ w1757]
          tunnel: [w1742 w1756] -> w1729
          tunnel: w1728 -> [w1742 w1755]
          tunnel: [w1742 w1752] -> w1726
          tunnel: w1725 -> [_ w1751]
          tunnel: w1724 -> [_ w1750]
          tunnel: w1723 -> [_ w1749]
          frame False {
            n367 = call "TableHandle.vi"("All"=w1745, "error in (no error)"=w1746, "DataIn"=TRUE) -> ("error out"=w1747:errorcluster, "Stop?"=w1744:bool)  [unwired: 3 in, 4 out]
          }
          frame True {
            n368 = property class="Ring (严格)"(reference=w1749) -> ("RingText.Text"=w1748:string)  [unwired: 1 in, 2 out]
            n369 = for "For循环" {
              N: w1758 -> [_]
              tunnel: w1763 -> [w1776]
              tunnel: [w1795] -> w1762
              tunnel: w1761 -> [w1792]
              tunnel: [w1793] -> w1760
              tunnel: w1759 -> [w1769]
              tunnel: w1754 -> [w1773]
              tunnel: w1757 -> [w1789]
              shift-right: [w1787] -> w1756
              shift-left: w1755 -> [w1788]
              tunnel: w1753 -> [w1774]
              tunnel: [w1771] -> w1752
              tunnel: w1751 -> [_]
              tunnel: w1750 -> [w1779]
              tunnel: w1748 -> [w1777]
              stop <- w1794 stop-if-true
              n370 = Match Pattern(string=w1769, regular expression=";" ("正则表达式")) -> (before substring=w1768:string, after substring=w1766:string)  [unwired: 1 in, 2 out]
              n371 = property class="Str"(reference=w1779) -> ("Value"=w1778:string)  [unwired: 1 in, 2 out]
              n372 = Decimal String To Number(string=w1768, default (0L)=u32 0 ("默认(0 I32)")) -> (number=w1784:u32)  [unwired: 1 in, 1 out]
              n373 = Match Pattern(string=w1773, regular expression=";" ("正则表达式")) -> (before substring=w1771:string, after substring=w1770:string)  [unwired: 1 in, 2 out]
              n374 = call "DOAction.vi"("Slot"=w1774, "error in"=w1776, "State"=w1766, "CH"=w1770) -> ("error out"=w1775:errorcluster)  [unwired: 7 in]
              n375 = case shown="\"Slot1\", 默认" w1774 {
                tunnel: [w1796 w1797] -> w1783
                frame "Slot1", Default {
                  n376 = global read "GlobalValue.vi" "Slot1COM"() -> (w1796:refnum<visa-resource-name>)
                }
                frame "Slot2" {
                  n377 = global read "GlobalValue.vi" "Slot2COM"() -> (w1797:refnum<visa-resource-name>)
                }
              }
              n378 = call "时间延迟"("error in (no error)"=w1775, "Delay Time (s)"=4.0) -> ("error out"=w1765:errorcluster)  [unwired: 9 in]
              n379 = call "CommunicationTool-Ver1.vi"("VISA资源名称"=w1783, "SN"=w1778, "ModelNumber"=w1777, "通信协议名称"=w1771, "Slot"=w1774, "DelayTime"=w1784, "error in"=w1765, "Debug"=FALSE) -> ("字符串数值"=w1781:bool, "CMD"=w1782:string, "data"=w1780:string, "error out"=w1791:errorcluster)  [unwired: 2 in, 2 out]
              n380 = Concatenate Strings(w1788, w1782) -> (w1787:string)
              n381 = String Length(string=w1787) -> (length=w1786:i32)
              n382 = property class="Str"(reference=w1789, "Text.Text"=w1787, "Text.Scroll Position"=w1786) -> ()  [unwired: 1 in, 2 out]
              n383 = call "TableHandle.vi"("All"=w1792, "error in (no error)"=w1791, "字符串数值"=w1781, "DataIn"=w1780) -> ("error out"=w1795:errorcluster, "Stop?"=w1793:bool, "StopForLoop"=w1794:bool)  [unwired: 3 in, 2 out]
            }
          }
        }
      }
      frame "FileReceive" {
        n384 = case shown="真" w1813 {
          tunnel: w1816 -> [w1820 w1835]
          tunnel: w1815 -> [w1821 w1837]
          tunnel: [w1822 w1836] -> w1814
          tunnel: [w1819 w1834] -> w1812
          tunnel: w1811 -> [_ w1827]
          tunnel: w1810 -> [_ w1828]
          tunnel: w1809 -> [_ w1833]
          tunnel: w1808 -> [_ w1832]
          tunnel: w1805 -> [_ w1831]
          tunnel: [w1817 w1830] -> w1804
          tunnel: w1803 -> [w1817 w1829]
          tunnel: [w1817 w1826] -> w1801
          tunnel: w1800 -> [_ w1825]
          tunnel: w1799 -> [_ w1824]
          tunnel: w1798 -> [_ w1823]
          frame False {
            n385 = call "TableHandle.vi"("All"=w1820, "error in (no error)"=w1821, "DataIn"=TRUE) -> ("error out"=w1822:errorcluster, "Stop?"=w1819:bool)  [unwired: 3 in, 4 out]
          }
          frame True {
            n386 = for "For循环" {
              N: w1832 -> [_]
              tunnel: w1837 -> [w1864]
              tunnel: [w1872] -> w1836
              tunnel: w1835 -> [w1869]
              tunnel: [w1870] -> w1834
              tunnel: w1833 -> [w1859]
              tunnel: w1828 -> [w1852]
              tunnel: w1831 -> [w1867]
              shift-right: [w1847] -> w1830
              shift-left: w1829 -> [w1848]
              tunnel: w1827 -> [w1851]
              tunnel: [w1852] -> w1826
              tunnel: w1825 -> [_]
              tunnel: w1824 -> [_]
              tunnel: w1823 -> [w1846]
              i -> [w1865]
              stop <- w1871 stop-if-true
              w1838 = "\n"
              n387 = Decimal String To Number(string=w1859, default (0L)=u32 0 ("默认(0 I32)")) -> (number=w1863:u32)  [unwired: 1 in, 1 out]
              n388 = case shown="1, 默认" w1865 {
                tunnel: w1864 -> [w1917 w1920]
                tunnel: [w1917 w1919] -> w1860
                tunnel: w1863 -> [_ w1918]
                frame 0 {
                }
                frame 1, Default {
                  n389 = call "WaitTimes.vi"("WaitTimes"=w1918, "error in (no error)"=w1920) -> ("error out"=w1919:errorcluster)  [unwired: 9 in]
                }
              }
              n390 = case shown="\"Slot1\", 默认" w1851 {
                tunnel: [w1915 w1916] -> w1862
                frame "Slot1", Default {
                  n391 = global read "GlobalValue.vi" "Slot1COM"() -> (w1915:refnum<visa-resource-name>)
                }
                frame "Slot2" {
                  n392 = global read "GlobalValue.vi" "Slot2COM"() -> (w1916:refnum<visa-resource-name>)
                }
              }
              n393 = case shown="\"上传秘钥文件并比较\"" w1846 {
                tunnel: [w1894 "上传证书文件通道参数错误！\n" ("消息") "上传证书文件通道参数错误！\n" ("消息")] -> w1853
                tunnel: w1851 -> [_ w1899 w1909]
                tunnel: [w1894 w1900 w1910] -> w1850
                tunnel: [w1894 w1895 w1905] -> w1849
                frame "假", Default {
                  w1894 = ""
                }
                frame "上传证书文件并比较" {
                  n394 = call "ccidinfo-r.vi"("Data Type"=PDINFO."CertifID", "Slot"=w1899) -> ("Data"=w1902:string)
                  n395 = call "ccidinfo-r.vi"("Data Type"=PDINFO."Reserved1", "Slot"=w1899) -> ("Data"=w1897:string)
                  n396 = call <vilib>:"Trim Whitespace.vi"("string"=w1902) -> ("trimmed string"=w1896:string)  [unwired: 1 in]
                  n397 = call <vilib>:"Trim Whitespace.vi"("string"=w1897) -> ("trimmed string"=w1895:string)  [unwired: 1 in]
                  n398 = Concatenate Strings(w1896, ".cer") -> (w1900:string)
                }
                frame "上传秘钥文件并比较" {
                  n399 = call "ccidinfo-r.vi"("Data Type"=PDINFO."CertifID", "Slot"=w1909) -> ("Data"=w1912:string)
                  n400 = call "ccidinfo-r.vi"("Data Type"=PDINFO."Reserved2", "Slot"=w1909) -> ("Data"=w1907:string)
                  n401 = call <vilib>:"Trim Whitespace.vi"("string"=w1912) -> ("trimmed string"=w1906:string)  [unwired: 1 in]
                  n402 = call <vilib>:"Trim Whitespace.vi"("string"=w1907) -> ("trimmed string"=w1905:string)  [unwired: 1 in]
                  n403 = Concatenate Strings(w1906, ".key") -> (w1910:string)
                }
              }
              n404 = Match Pattern(string=w1852, regular expression=";") -> (before substring=w1857:string, after substring=w1856:string, offset past match=w1855:i32)  [unwired: 1 in, 1 out]
              n405 = Greater Than 0?(x=w1855) -> (x > 0?=w1854:bool)
              n406 = call "StrTo16.vi"("StrIn"=w1849) -> ("StrOut"=w1840:string)
              n407 = case shown="假" w1854 {
                tunnel: w1862 -> [_ w1893]
                tunnel: [FALSE w1885] -> w1845
                tunnel: [w1875 w1892] -> w1861
                tunnel: w1860 -> [w1878 w1891]
                tunnel: w1857 -> [_ w1889]
                tunnel: w1856 -> [_ w1890]
                tunnel: w1853 -> [w1876 _]
                tunnel: w1852 -> [w1874 _]
                tunnel: w1850 -> [_ w1886]
                tunnel: w1840 -> [_ w1883]
                tunnel: [w1873 w1880] -> w1839
                frame False {
                  n408 = Concatenate Strings(w1876, w1874) -> (w1873:string)
                  n409 = call <vilib>:"Clear Errors.vi"("error in (no error)"=w1878) -> ("error out"=w1875:errorcluster)  [unwired: 6 in]
                  n410 = disable-structure shown="禁用" {
                    disable-tunnel: w1873 -> [w1879 _]
                    frame Disabled {
                      n411 = One Button Dialog(message=w1879) -> ()  [unwired: 1 in, 1 out]
                    }
                    frame Enabled {
                    }
                  }
                }
                frame True {
                  n412 = Concatenate Strings(w1889, "/", w1886) -> (w1887:string)
                  n413 = call "FilePackageReceive.vi"("error in"=w1891, "PCFileLocation"=w1890, "PdFileLocation"=w1887, "ComIn"=w1893) -> ("error out"=w1892:errorcluster, "MD5"=w1884:string, "Result"=w1881:bool, "FileText"=w1880:string)  [unwired: 2 in, 2 out]
                  n414 = Equal?(x=w1884, y=w1883) -> (x = y?=w1882:bool)
                  n415 = And(x=w1881, y=w1882) -> (x .and. y?=w1885:bool)
                }
              }
              n416 = Select(t="PASS", s=w1845, f="FAIL") -> (s? t:f=w1842:string)
              n417 = Concatenate Strings(w1848, w1846, ":  " ("字符串"), w1842, w1838, w1839, w1838) -> (w1847:string)
              n418 = String Length(string=w1847) -> (length=w1866:i32)
              n419 = property class="Str"(reference=w1867, "Text.Text"=w1847, "Text.Scroll Position"=w1866) -> ()  [unwired: 1 in, 2 out]
              n420 = call "TableHandle.vi"("All"=w1869, "error in (no error)"=w1861, "DataIn"=w1845) -> ("error out"=w1872:errorcluster, "Stop?"=w1870:bool, "StopForLoop"=w1871:bool)  [unwired: 4 in, 2 out]
            }
          }
        }
      }
      frame "FileTransfer" {
        n421 = case shown="真" w1936 {
          tunnel: w1939 -> [w1943 w1958]
          tunnel: w1938 -> [w1944 w1960]
          tunnel: [w1945 w1959] -> w1937
          tunnel: [w1942 w1957] -> w1935
          tunnel: w1934 -> [_ w1950]
          tunnel: w1933 -> [_ w1951]
          tunnel: w1932 -> [_ w1956]
          tunnel: w1931 -> [_ w1955]
          tunnel: w1928 -> [_ w1954]
          tunnel: [w1940 w1953] -> w1927
          tunnel: w1926 -> [w1940 w1952]
          tunnel: [w1940 w1949] -> w1924
          tunnel: w1923 -> [_ w1948]
          tunnel: w1922 -> [_ w1947]
          tunnel: w1921 -> [_ w1946]
          frame False {
            n422 = call "TableHandle.vi"("All"=w1943, "error in (no error)"=w1944, "DataIn"=TRUE) -> ("error out"=w1945:errorcluster, "Stop?"=w1942:bool)  [unwired: 3 in, 4 out]
          }
          frame True {
            n423 = for "For循环" {
              N: w1955 -> [_]
              tunnel: w1960 -> [w1993]
              tunnel: [w2001] -> w1959
              tunnel: w1958 -> [w1998]
              tunnel: [w1999] -> w1957
              tunnel: w1956 -> [w1984]
              tunnel: w1951 -> [w1978]
              tunnel: w1954 -> [w1996]
              shift-right: [w1968] -> w1953
              shift-left: w1952 -> [w1970]
              tunnel: w1950 -> [w1975]
              tunnel: [w1978] -> w1949
              tunnel: w1948 -> [_]
              tunnel: w1947 -> [_]
              tunnel: w1946 -> [w1973]
              i -> [w1994]
              stop <- w2000 stop-if-true
              w1961 = "\n"
              n424 = Match Pattern(string=w1984, regular expression=";") -> (before substring=w1983:string, after substring=w1980:string)  [unwired: 1 in, 2 out]
              n425 = Decimal String To Number(string=w1980, default (0L)=u32 0 ("默认(0 I32)")) -> (number=w1979:u32)  [unwired: 1 in, 1 out]
              n426 = Decimal String To Number(string=w1983, default (0L)=u32 0 ("默认(0 I32)")) -> (number=w1992:u32)  [unwired: 1 in, 1 out]
              n427 = case shown="\"下载秘钥文件\"" w1973 {
                tunnel: [w2002 "证书文件未找到！\n" ("消息") "秘钥文件未找到！\n" ("消息")] -> w1985
                tunnel: w1975 -> [_ w2009 w2016]
                tunnel: [w2002 w2005 w2012] -> w1976
                tunnel: [_ PDINFO."Reserved1" ("Data Type") PDINFO."Reserved2" ("Data Type")] -> w1974
                frame "假", Default {
                  w2002 = ""
                }
                frame "下载证书文件" {
                  n428 = call "ccidinfo-r.vi"("Data Type"=PDINFO."CertifID", "Slot"=w2009) -> ("Data"=w2007:string)
                  n429 = call <vilib>:"Trim Whitespace.vi"("string"=w2007) -> ("trimmed string"=w2003:string)  [unwired: 1 in]
                  n430 = Concatenate Strings(w2003, ".cer") -> (w2005:string)
                }
                frame "下载秘钥文件" {
                  n431 = call "ccidinfo-r.vi"("Data Type"=PDINFO."CertifID", "Slot"=w2016) -> ("Data"=w2014:string)
                  n432 = Concatenate Strings(w2014, ".key") -> (w2012:string)
                }
              }
              n433 = case shown="\"Slot1\", 默认" w1975 {
                tunnel: [w2037 w2038] -> w1991
                frame "Slot1", Default {
                  n434 = global read "GlobalValue.vi" "Slot1COM"() -> (w2037:refnum<visa-resource-name>)
                }
                frame "Slot2" {
                  n435 = global read "GlobalValue.vi" "Slot2COM"() -> (w2038:refnum<visa-resource-name>)
                }
              }
              n436 = case shown="1, 默认" w1994 {
                tunnel: w1993 -> [w2039 w2042]
                tunnel: [w2039 w2041] -> w1989
                tunnel: w1992 -> [_ w2040]
                frame 0 {
                }
                frame 1, Default {
                  n437 = call "WaitTimes.vi"("WaitTimes"=w2040, "error in (no error)"=w2042) -> ("error out"=w2041:errorcluster)  [unwired: 9 in]
                }
              }
              n438 = Concatenate Strings(w1978, "\\", w1976) -> (w1963:string)
              n439 = String To Path(string=w1963) -> (path=w1988:path)
              n440 = call <vilib>:"Check if File or Folder Exists.vi"("error in (no error)"=w1989, "path"=w1988) -> ("error out"=w1986:errorcluster, "file or folder exists?"=w1987:bool)  [unwired: 7 in, 1 out]
              n441 = case shown="假" w1987 {
                tunnel: w1991 -> [_ w2036]
                tunnel: [FALSE ("Result") w2035] -> w1964
                tunnel: [w2022 w2034] -> w1990
                tunnel: w1986 -> [w2021 w2033]
                tunnel: w1985 -> [w2020 _]
                tunnel: w1979 -> [_ w2031]
                tunnel: w1975 -> [_ w2030]
                tunnel: w1974 -> [_ w2029]
                tunnel: [_ w2028] -> w1969
                tunnel: w1963 -> [w2019 w2027]
                tunnel: [w2018 w2025] -> w1962
                frame False {
                  n442 = call <vilib>:"Clear Errors.vi"("error in (no error)"=w2021) -> ("error out"=w2022:errorcluster)  [unwired: 6 in]
                  n443 = Concatenate Strings(w2020, w2019) -> (w2018:string)
                  n444 = disable-structure shown="禁用" {
                    disable-tunnel: w2018 -> [w2024 _]
                    frame Disabled {
                      n445 = One Button Dialog(message=w2024) -> ()  [unwired: 1 in, 1 out]
                    }
                    frame Enabled {
                    }
                  }
                }
                frame True {
                  n446 = call <vilib>:"Clear Errors.vi"("error in (no error)"=w2033) -> ("error out"=w2032:errorcluster)  [unwired: 6 in]
                  n447 = call "FliePackageTransfer.vi"("TransferMode"=w2031, "error in"=w2032, "TbcFilePath"=w2027, "ComIn"=w2036) -> ("error out"=w2034:errorcluster, "MD5"=w2028:string, "FeedBack"=w2026:string[], "Result"=w2035:bool)  [unwired: 4 in]
                  n448 = Index Array(array=w2026) -> (element=w2025:string)  [unwired: 1 in]
                  n449 = call "ccidinfo-w.vi"("Data"=w2028, "Data Type"=w2029, "Slot"=w2030) -> ()  [unwired: 1 in]
                }
              }
              n450 = Select(t="PASS", s=w1964, f="FAIL") -> (s? t:f=w1967:string)
              n451 = Concatenate Strings(w1970, w1973, ": ", "MD5值", w1961, w1969, w1961, w1967, w1961, w1962, w1961) -> (w1968:string)
              n452 = String Length(string=w1968) -> (length=w1995:i32)
              n453 = property class="Str"(reference=w1996, "Text.Text"=w1968, "Text.Scroll Position"=w1995) -> ()  [unwired: 1 in, 2 out]
              n454 = call "TableHandle.vi"("All"=w1998, "error in (no error)"=w1990, "DataIn"=w1964) -> ("error out"=w2001:errorcluster, "Stop?"=w1999:bool, "StopForLoop"=w2000:bool)  [unwired: 4 in, 2 out]
            }
          }
        }
      }
      frame "FindSIMCOMETH" {
        n455 = case shown="真" w2053 {
          tunnel: w2056 -> [w2059 w2067]
          tunnel: w2055 -> [w2060 w2069]
          tunnel: [w2061 w2068] -> w2054
          tunnel: [w2058 w2066] -> w2052
          tunnel: w2051 -> [_ w2065]
          tunnel: w2050 -> [_ w2064]
          tunnel: w2049 -> [_ w2063]
          tunnel: w2048 -> [_ w2062]
          frame False {
            n456 = call "TableHandle.vi"("All"=w2059, "error in (no error)"=w2060, "DataIn"=TRUE) -> ("error out"=w2061:errorcluster, "Stop?"=w2058:bool)  [unwired: 3 in, 4 out]
          }
          frame True {
            n457 = for "For循环" {
              N: w2062 -> [_]
              tunnel: w2069 -> [w2079]
              tunnel: [w2083] -> w2068
              tunnel: w2067 -> [w2080]
              tunnel: [w2081] -> w2066
              tunnel: w2065 -> [w2070]
              tunnel: w2063 -> [w2076]
              tunnel: w2064 -> [_]
              stop <- w2082 stop-if-true
              n458 = case shown="\"Slot1\", 默认" w2070 {
                tunnel: [w2087 w2090] -> w2072
                tunnel: [w2088 w2089] -> w2073
                frame "Slot1", Default {
                  n459 = global read "GlobalValue.vi" "Slot1USBCOM"() -> (w2087:refnum<visa-resource-name>)
                  n460 = global read "GlobalValue.vi" "Slot1USB"() -> (w2088:string)
                }
                frame "Slot2" {
                  n461 = global read "GlobalValue.vi" "Slot2USBCOM"() -> (w2090:refnum<visa-resource-name>)
                  n462 = global read "GlobalValue.vi" "Slot2USB"() -> (w2089:string)
                }
              }
              n463 = Decimal String To Number(string=w2076) -> (number=w2075:i32)  [unwired: 2 in, 1 out]
              n464 = Empty String/Path?(string/path=w2072) -> (empty?=w2074:bool)
              n465 = case shown="真" w2074 {
                tunnel: [w2084 w2086] -> w2071
                tunnel: w2073 -> [_ w2085]
                tunnel: w2072 -> [w2084 _]
                frame False {
                }
                frame True {
                  n466 = call "SearchUSB.vi"("USB"=w2085) -> ("USBPort"=w2086:refnum<visa-resource-name>)  [unwired: 9 in, 1 out]
                }
              }
              n467 = for {
                N: w2075 -> [_]
                tunnel: [w2093] -> w2077
                shift-right: [w2094] -> w2078
                shift-left: w2079 -> [w2095]
                tunnel: w2071 -> [w2092]
                stop <- w2093 stop-if-true
                n468 = call "FindSimETH.vi"("COM"=w2092, "error in (no error)"=w2095) -> ("error out"=w2094:errorcluster, "Pass"=w2093:bool)  [unwired: 7 in, 1 out]
                n469 = Wait (ms)(milliseconds to wait=u32 500 ("等待时间（毫秒）")) -> ()  [unwired: 1 out]
              }
              n470 = call "TableHandle.vi"("All"=w2080, "error in (no error)"=w2078, "DataIn"=w2077) -> ("error out"=w2083:errorcluster, "Stop?"=w2081:bool, "StopForLoop"=w2082:bool)  [unwired: 4 in, 2 out]
            }
          }
        }
      }
      frame "FindSIMCOMETH_CAn" {
        n471 = case shown="真" w2108 {
          tunnel: w2104 -> [w2116 w2128]
          tunnel: w2105 -> [w2117 w2130]
          tunnel: [w2118 w2129] -> w2101
          tunnel: [w2115 w2127] -> w2100
          tunnel: w2103 -> [_ w2126]
          tunnel: w2107 -> [_ w2125]
          tunnel: w2106 -> [_ w2124]
          tunnel: w2109 -> [_ w2123]
          tunnel: w2099 -> [_ w2122]
          tunnel: w2098 -> [_ w2121]
          tunnel: w2097 -> [w2113 w2120]
          tunnel: [w2113 w2119] -> w2096
          frame False {
            n472 = call "TableHandle.vi"("All"=w2116, "error in (no error)"=w2117, "DataIn"=TRUE) -> ("error out"=w2118:errorcluster, "Stop?"=w2115:bool)  [unwired: 3 in, 4 out]
          }
          frame True {
            n473 = for "For循环" {
              N: w2123 -> [_]
              tunnel: w2130 -> [w2154]
              tunnel: [w2158] -> w2129
              tunnel: w2128 -> [w2155]
              tunnel: [w2156] -> w2127
              tunnel: w2126 -> [w2146]
              tunnel: w2124 -> [w2151]
              tunnel: w2125 -> [_]
              tunnel: w2122 -> [w2145]
              tunnel: w2121 -> [w2143]
              shift-right: [w2131] -> w2119
              shift-left: w2120 -> [w2144]
              stop <- w2157 stop-if-true
              n474 = case shown="\"Slot1\", 默认" w2146 {
                tunnel: [w2162 w2165] -> w2142
                tunnel: [w2163 w2164] -> w2148
                frame "Slot1", Default {
                  n475 = global read "GlobalValue.vi" "Slot1USBCOM"() -> (w2162:refnum<visa-resource-name>)
                  n476 = global read "GlobalValue.vi" "Slot1USB"() -> (w2163:string)
                }
                frame "Slot2" {
                  n477 = global read "GlobalValue.vi" "Slot2USBCOM"() -> (w2165:refnum<visa-resource-name>)
                  n478 = global read "GlobalValue.vi" "Slot2USB"() -> (w2164:string)
                }
              }
              n479 = Decimal String To Number(string=w2151) -> (number=w2150:i32)  [unwired: 2 in, 1 out]
              n480 = To Variant(anything=w2142) -> (Variant=w2141:variant)
              n481 = Empty String/Path?(string/path=w2142) -> (empty?=w2149:bool)
              n482 = Variant To Flattened String(Variant=w2141) -> (data string=w2140:string)  [unwired: 1 out]
              n483 = case shown="假" w2149 {
                tunnel: [w2159 w2161] -> w2147
                tunnel: w2148 -> [_ w2160]
                tunnel: w2142 -> [w2159 _]
                frame False {
                }
                frame True {
                  n484 = call "SearchUSB.vi"("USB"=w2160) -> ("USBPort"=w2161:refnum<visa-resource-name>)  [unwired: 9 in, 1 out]
                }
              }
              n485 = String Length(string=w2140) -> (length=w2139:i32)
              n486 = Subtract(x=w2139, y=4) -> (x-y=w2137:i32)
              n487 = String Subset(string=w2140, offset (0)=4, length (rest)=w2137) -> (substring=w2134:string)
              n488 = for {
                N: w2150 -> [_]
                tunnel: [w2166] -> w2152
                shift-right: [w2167] -> w2153
                shift-left: w2154 -> [w2169]
                tunnel: w2147 -> [w2168]
                stop <- w2166 stop-if-true
                n489 = call "FindSimETH_CAn.vi"("COM"=w2168, "error in"=w2169) -> ("error out"=w2167:errorcluster, "Pass"=w2166:bool)  [unwired: 7 in, 1 out]
                n490 = Wait (ms)(milliseconds to wait=u32 500 ("等待时间（毫秒）")) -> ()  [unwired: 1 out]
              }
              n491 = Concatenate Strings(w2144, w2143, ": " ("字符串"), w2134, "\n") -> (w2131:string)
              n492 = String Length(string=w2131) -> (length=w2132:i32)
              n493 = property class="Str"(reference=w2145, "Text.Text"=w2131, "Text.Scroll Position"=w2132) -> ()  [unwired: 1 in, 2 out]
              n494 = call "TableHandle.vi"("All"=w2155, "error in (no error)"=w2153, "DataIn"=w2152) -> ("error out"=w2158:errorcluster, "Stop?"=w2156:bool, "StopForLoop"=w2157:bool)  [unwired: 4 in, 2 out]
            }
          }
        }
      }
      frame "FindSIMCOMETH_CF" {
        n495 = case shown="真" w2182 {
          tunnel: w2185 -> [w2188 w2197]
          tunnel: w2184 -> [w2189 w2199]
          tunnel: [w2190 w2198] -> w2183
          tunnel: [w2187 w2196] -> w2181
          tunnel: w2180 -> [_ w2195]
          tunnel: w2179 -> [_ w2194]
          tunnel: w2178 -> [_ w2193]
          tunnel: w2177 -> [_ w2192]
          tunnel: w2171 -> [_ w2191]
          frame False {
            n496 = call "TableHandle.vi"("All"=w2188, "error in (no error)"=w2189, "DataIn"=TRUE) -> ("error out"=w2190:errorcluster, "Stop?"=w2187:bool)  [unwired: 3 in, 4 out]
          }
          frame True {
            n497 = for "For循环" {
              N: w2192 -> [_]
              tunnel: w2199 -> [w2208]
              tunnel: [w2212] -> w2198
              tunnel: w2197 -> [w2209]
              tunnel: [w2210] -> w2196
              tunnel: w2195 -> [w2205]
              tunnel: w2193 -> [w2206]
              tunnel: w2194 -> [w2200]
              tunnel: w2191 -> [w2201]
              stop <- w2211 stop-if-true
              n498 = Decimal String To Number(string=w2206) -> (number=w2203:i32)  [unwired: 2 in, 1 out]
              n499 = for {
                N: 2 -> [_]
                tunnel: w2205 -> [w2215]
                tunnel: [w2213] -> w2204
                tunnel: w2203 -> [w2225]
                shift-right: [w2217] -> w2207
                shift-left: w2208 -> [w2224]
                tunnel: w2201 -> [w2221]
                tunnel: w2200 -> [w2219]
                i -> [w2216]
                stop <- w2213 stop-if-true
                n500 = case shown="0, 默认" w2216 {
                  tunnel: [w2256 w2259] -> w2228
                  tunnel: [w2257 w2258] -> w2226
                  frame 0, Default {
                    n501 = global read "GlobalValue.vi" "Slot1USBCOM"() -> (w2256:refnum<visa-resource-name>)
                    n502 = global read "GlobalValue.vi" "Slot1USB"() -> (w2257:string)
                  }
                  frame 1 {
                    n503 = global read "GlobalValue.vi" "Slot2USBCOM"() -> (w2259:refnum<visa-resource-name>)
                    n504 = global read "GlobalValue.vi" "Slot2USB"() -> (w2258:string)
                  }
                }
                n505 = call <vilib>:"Clear Errors.vi"("error in (no error)"=w2224) -> ("error out"=w2223:errorcluster)  [unwired: 6 in]
                n506 = Empty String/Path?(string/path=w2228) -> (empty?=w2227:bool)
                n507 = case shown="假" w2227 {
                  tunnel: [w2253 w2255] -> w2214
                  tunnel: w2226 -> [_ w2254]
                  tunnel: w2228 -> [w2253 _]
                  frame False {
                  }
                  frame True {
                    n508 = call "SearchUSB_CF.vi"("USB"=w2254) -> ("USBPort"=w2255:refnum<visa-resource-name>)  [unwired: 9 in, 1 out]
                  }
                }
                n509 = for {
                  N: w2225 -> [_]
                  tunnel: [w2263] -> w2222
                  shift-right: [w2264] -> w2218
                  shift-left: w2223 -> [w2265]
                  tunnel: w2214 -> [w2260]
                  tunnel: [w2261] -> _
                  tunnel: [w2260] -> w2220
                  stop <- w2263 stop-if-true
                  n510 = call "FindSimETH_CF.vi"("COM"=w2260, "error in (no error)"=w2265) -> ("error out"=w2264:errorcluster, "Pass"=w2263:bool, "CmdOut"=w2261:string)  [unwired: 7 in]
                  n511 = Wait (ms)(milliseconds to wait=u32 500 ("等待时间（毫秒）")) -> ()  [unwired: 1 out]
                }
                n512 = case shown="真" w2222 {
                  tunnel: w2221 -> [_ w2250]
                  tunnel: w2220 -> [_ w2249]
                  tunnel: w2219 -> [_ w2248]
                  tunnel: w2218 -> [w2232 w2246]
                  tunnel: [w2232 w2245] -> w2217
                  tunnel: [FALSE w2236] -> w2213
                  tunnel: w2216 -> [_ w2244]
                  tunnel: w2215 -> [w2230 w2241]
                  tunnel: w2214 -> [_ w2242]
                  frame False {
                    n513 = case shown="\"Slot2\"" w2230 {
                      tunnel: "" -> [w2233 w2234]
                      frame "Slot1", Default {
                        n514 = global write "GlobalValue.vi" "Slot1USBCOM DY"(w2233) -> ()
                      }
                      frame "Slot2" {
                        n515 = global write "GlobalValue.vi" "Slot2USBCOM DY"(w2234) -> ()
                      }
                    }
                  }
                  frame True {
                    n516 = case shown="\"Slot2\"" w2241 {
                      tunnel: w2242 -> [w2251 w2252]
                      frame "Slot1", Default {
                        n517 = global write "GlobalValue.vi" "Slot1USBCOM DY"(w2251) -> ()
                      }
                      frame "Slot2" {
                        n518 = global write "GlobalValue.vi" "Slot2USBCOM DY"(w2252) -> ()
                      }
                    }
                    n519 = call "SIMCOMCommunicationTool_CF.vi"("VISA资源名称"=w2249, "MSComm"=w2250, "通信协议名称"=w2248, "DelayTime"=u32 500, "error in"=w2246, "Debug"=FALSE, "Slot"=w2244) -> ("反馈结果"=w2235:bool, "ReturnData"=w2238:string, "error out"=w2245:errorcluster)  [unwired: 4 in, 2 out]
                    n520 = call "ccidinfo-r.vi"("Data Type"=PDINFO."CCID", "Slot"=w2241) -> ("Data"=w2239:string)
                    n521 = Equal?(x=w2238, y=w2239) -> (x = y?=w2237:bool)
                    n522 = And(x=w2235, y=w2237) -> (x .and. y?=w2236:bool)
                  }
                }
              }
              n523 = call "TableHandle.vi"("All"=w2209, "error in (no error)"=w2207, "DataIn"=w2204) -> ("error out"=w2212:errorcluster, "Stop?"=w2210:bool, "StopForLoop"=w2211:bool)  [unwired: 4 in, 2 out]
            }
          }
        }
      }
      frame "Frequency" {
        n524 = case shown="真" w2277 {
          tunnel: w2280 -> [w2284 w2293]
          tunnel: w2279 -> [w2285 w2295]
          tunnel: [w2286 w2294] -> w2278
          tunnel: [w2283 w2292] -> w2276
          tunnel: w2275 -> [_ w2291]
          tunnel: w2274 -> [_ w2290]
          tunnel: w2273 -> [_ w2289]
          tunnel: w2272 -> [_ w2288]
          tunnel: w2271 -> [w2281 w2287]
          tunnel: [w2281 w2287] -> w2270
          frame False {
            n525 = call "TableHandle.vi"("All"=w2284, "error in (no error)"=w2285, "DataIn"=TRUE) -> ("error out"=w2286:errorcluster, "Stop?"=w2283:bool)  [unwired: 3 in, 4 out]
          }
          frame True {
            n526 = for "For循环" {
              N: w2288 -> [_]
              tunnel: w2295 -> [w2299]
              tunnel: [w2303] -> w2294
              tunnel: w2293 -> [w2300]
              tunnel: [w2301] -> w2292
              tunnel: w2291 -> [_]
              tunnel: w2289 -> [_]
              tunnel: w2290 -> [_]
              tunnel: w2287 -> [w2297]
              stop <- w2302 stop-if-true
              n527 = call-poly <vilib>:"Extract Single Tone Information.vi"("error in (no error)"=w2299, "time signal in"=w2297) -> ("error out"=w2298:errorcluster, "detected frequency"=w2296:dbl)  [unwired: 4 in, 4 out]
              n528 = call "TableHandle.vi"("All"=w2300, "error in (no error)"=w2298, "DataIn"=w2296) -> ("error out"=w2303:errorcluster, "Stop?"=w2301:bool, "StopForLoop"=w2302:bool)  [unwired: 4 in, 2 out]
            }
          }
        }
      }
      frame "MeaCurrent" {
        n529 = case shown="真" w2314 {
          tunnel: w2317 -> [w2320 w2329]
          tunnel: w2316 -> [w2321 w2331]
          tunnel: [w2322 w2330] -> w2315
          tunnel: [w2319 w2328] -> w2313
          tunnel: w2312 -> [_ w2327]
          tunnel: w2311 -> [_ w2326]
          tunnel: w2310 -> [_ w2325]
          tunnel: w2309 -> [_ w2324]
          tunnel: w2304 -> [_ w2323]
          frame False {
            n530 = call "TableHandle.vi"("All"=w2320, "error in (no error)"=w2321, "DataIn"=TRUE) -> ("error out"=w2322:errorcluster, "Stop?"=w2319:bool)  [unwired: 3 in, 4 out]
          }
          frame True {
            n531 = for "For循环" {
              N: w2324 -> [_]
              tunnel: w2331 -> [w2341]
              tunnel: [w2348] -> w2330
              tunnel: w2329 -> [w2345]
              tunnel: [w2346] -> w2328
              tunnel: w2327 -> [w2342]
              tunnel: w2325 -> [w2344]
              tunnel: w2326 -> [w2343]
              tunnel: w2323 -> [w2339]
              i -> [w2338]
              stop <- w2347 stop-if-true
              w2334 = 3
              n532 = case shown="\"Slot1\", 默认" w2342 {
                tunnel: [w2363 w2364] -> w2340
                frame "Slot1", Default {
                  n533 = global read "GlobalValue.vi" "Slot1COM"() -> (w2363:refnum<visa-resource-name>)
                }
                frame "Slot2" {
                  n534 = global read "GlobalValue.vi" "Slot2COM"() -> (w2364:refnum<visa-resource-name>)
                }
              }
              n535 = case shown="1, 默认" w2338 {
                tunnel: w2341 -> [w2356 w2361]
                tunnel: [w2356 w2360] -> w2332
                tunnel: w2340 -> [_ w2359]
                tunnel: w2339 -> [_ w2358]
                frame 0 {
                }
                frame 1, Default {
                  n536 = call "CommunicationTool.vi"("VISA资源名称"=w2359, "通信协议名称"=w2358, "DelayTime"=u32 1000, "error in"=w2361, "Debug"=FALSE) -> ("error out"=w2360:errorcluster)  [unwired: 5 in, 5 out]
                }
              }
              n537 = for {
                N: w2334 -> [_]
                tunnel: w2344 -> [w2355]
                tunnel: w2343 -> [w2354]
                tunnel: w2342 -> [w2353]
                tunnel: [w2350] -> w2336 mode=indexing
                shift-right: [w2352] -> w2337
                shift-left: w2332 -> [w2349]
                n538 = Build Array(w2354) -> (w2351:string[])
                n539 = call "AIs-Freq.vi"("Slot"=w2353, "error in"=w2349, "Mode"=w2355, "CHs"=w2351) -> ("error out"=w2352:errorcluster, "RMS value"=w2350:dbl)  [unwired: 5 in, 1 out]
              }
              n540 = Add Array Elements(numeric array=w2336) -> (sum=w2335:dbl)
              n541 = Divide(x=w2335, y=w2334) -> (x/y=w2333:dbl)
              n542 = call "TableHandle.vi"("All"=w2345, "error in (no error)"=w2337, "DataIn"=w2333) -> ("error out"=w2348:errorcluster, "Stop?"=w2346:bool, "StopForLoop"=w2347:bool)  [unwired: 4 in, 2 out]
            }
          }
        }
      }
      frame "Ping" {
        n543 = case shown="真" w2375 {
          tunnel: w2378 -> [w2381 w2389]
          tunnel: w2377 -> [w2382 w2391]
          tunnel: [w2383 w2390] -> w2376
          tunnel: [w2380 w2388] -> w2374
          tunnel: w2373 -> [_ w2387]
          tunnel: w2372 -> [_ w2386]
          tunnel: w2371 -> [_ w2385]
          tunnel: w2370 -> [_ w2384]
          frame False {
            n544 = call "TableHandle.vi"("All"=w2381, "error in (no error)"=w2382, "DataIn"=TRUE) -> ("error out"=w2383:errorcluster, "Stop?"=w2380:bool)  [unwired: 3 in, 4 out]
          }
          frame True {
            n545 = for "For循环" {
              N: w2384 -> [_]
              tunnel: w2391 -> [w2404]
              tunnel: [w2408] -> w2390
              tunnel: w2389 -> [w2405]
              tunnel: [w2406] -> w2388
              tunnel: w2387 -> [_]
              tunnel: w2385 -> [w2402]
              tunnel: w2386 -> [w2398]
              stop <- w2407 stop-if-true
              n546 = Fract/Exp String To Number(string=w2402) -> (number=w2401:dbl)  [unwired: 3 in, 1 out]
              n547 = Multiply(x=w2401, y=1000.0) -> (x*y=w2400:dbl)
              n548 = To Unsigned Long Integer(number=w2400) -> (unsigned 32bit integer=w2399:u32)
              n549 = call "WaitTimes.vi"("WaitTimes"=w2399, "error in (no error)"=w2404) -> ("error out"=w2396:errorcluster)  [unwired: 9 in]
              n550 = call "Ping.vi"("error in"=w2396, "NetAdress"=w2398) -> ("error out"=w2395:errorcluster, "Acess"=w2397:bool)
              n551 = Select(t="PASS", s=w2397, f="FAIL") -> (s? t:f=w2394:string)
              n552 = call "TableHandle.vi"("All"=w2405, "error in (no error)"=w2395, "DataIn"=w2394) -> ("error out"=w2408:errorcluster, "Stop?"=w2406:bool, "StopForLoop"=w2407:bool)  [unwired: 4 in, 2 out]
            }
          }
        }
      }
      frame "QuitProcess" {
        n553 = case shown="真" w2420 {
          tunnel: w2423 -> [w2426 w2434]
          tunnel: w2422 -> [w2427 w2436]
          tunnel: [w2428 w2435] -> w2421
          tunnel: [w2425 w2433] -> w2419
          tunnel: w2418 -> [_ w2432]
          tunnel: w2417 -> [_ w2431]
          tunnel: w2416 -> [_ w2430]
          tunnel: w2415 -> [_ w2429]
          tunnel: w2412 -> [_ _]
          frame False {
            n554 = call "TableHandle.vi"("All"=w2426, "error in (no error)"=w2427, "DataIn"=TRUE) -> ("error out"=w2428:errorcluster, "Stop?"=w2425:bool)  [unwired: 3 in, 4 out]
          }
          frame True {
            n555 = for "For循环" {
              N: w2429 -> [_]
              tunnel: w2436 -> [w2438]
              tunnel: [w2447] -> w2435
              tunnel: w2434 -> [w2444]
              tunnel: [w2445] -> w2433
              tunnel: w2432 -> [w2443]
              tunnel: w2430 -> [w2442]
              tunnel: w2431 -> [_]
              stop <- w2446 stop-if-true
              n556 = case shown="\"Slot1\", 默认" w2443 {
                tunnel: [w2448 w2449] -> w2440
                frame "Slot1", Default {
                  n557 = global read "GlobalValue.vi" "Slot1COM"() -> (w2448:refnum<visa-resource-name>)
                }
                frame "Slot2" {
                  n558 = global read "GlobalValue.vi" "Slot2COM"() -> (w2449:refnum<visa-resource-name>)
                }
              }
              n559 = Decimal String To Number(string=w2442) -> (number=w2441:i32)  [unwired: 2 in, 1 out]
              n560 = call "QuitProcess.vi"("error in"=w2438, "WDelay"=w2441, "ComIn"=w2440) -> ("error out"=w2437:errorcluster, "OK？"=w2439:bool)  [unwired: 6 in, 1 out]
              n561 = call "TableHandle.vi"("All"=w2444, "error in (no error)"=w2437, "DataIn"=w2439) -> ("error out"=w2447:errorcluster, "Stop?"=w2445:bool, "StopForLoop"=w2446:bool)  [unwired: 4 in, 2 out]
            }
          }
        }
      }
      frame "RMS" {
        n562 = case shown="真" w2462 {
          tunnel: w2465 -> [w2469 w2479]
          tunnel: w2464 -> [w2470 w2481]
          tunnel: [w2471 w2480] -> w2463
          tunnel: [w2468 w2478] -> w2461
          tunnel: w2460 -> [_ w2477]
          tunnel: w2459 -> [_ w2476]
          tunnel: w2458 -> [_ w2475]
          tunnel: w2457 -> [_ w2474]
          tunnel: w2456 -> [w2466 w2473]
          tunnel: [w2466 w2473] -> w2455
          tunnel: w2452 -> [_ w2472]
          frame False {
            n563 = call "TableHandle.vi"("All"=w2469, "error in (no error)"=w2470, "DataIn"=TRUE) -> ("error out"=w2471:errorcluster, "Stop?"=w2468:bool)  [unwired: 3 in, 4 out]
          }
          frame True {
            n564 = for "For循环" {
              N: w2474 -> [_]
              tunnel: w2481 -> [w2488]
              tunnel: [w2494] -> w2480
              tunnel: w2479 -> [w2491]
              tunnel: [w2492] -> w2478
              tunnel: w2477 -> [w2482]
              tunnel: w2475 -> [_]
              tunnel: w2476 -> [_]
              tunnel: w2473 -> [w2485]
              tunnel: w2472 -> [w2484]
              i -> [w2483]
              stop <- w2493 stop-if-true
              n565 = case shown="1, 默认" w2483 {
                tunnel: w2488 -> [w2496 w2507]
                tunnel: [w2496 w2506] -> w2487
                tunnel: w2484 -> [_ w2505]
                tunnel: w2482 -> [_ w2501]
                tunnel: [w2495 w2502] -> w2486
                tunnel: w2485 -> [w2495 _]
                frame 0 {
                }
                frame 1, Default {
                  n566 = call "GlobalVariable.vi"("Name"="CH", "Slot"=w2501) -> ("String"=w2500:string)  [unwired: 10 in, 3 out]
                  n567 = call "GlobalVariable.vi"("Name"="Para", "Slot"=w2501) -> ("String"=w2497:string)  [unwired: 10 in, 3 out]
                  n568 = Build Array(w2500) -> (w2504:string[])
                  n569 = call "AIs-Freq.vi"("Slot"=w2501, "error in"=w2507, "Mode"=w2497, "CHs"=w2504) -> ("error out"=w2506:errorcluster, "波形图"=w2503:waveform(dbl)[])  [unwired: 5 in, 1 out]
                  n570 = property class="WFGraph (严格)"(reference=w2505, "Value"=w2503, "XScale.Minimum"=0.0 ("X标尺.范围:最小值"), "XScale.Maximum"=0.01 ("X标尺.范围:最大值")) -> ()  [unwired: 1 in, 2 out]
                  n571 = Index Array(array=w2503) -> (element=w2502:waveform(dbl))  [unwired: 1 in]
                }
              }
              n572 = call-poly <vilib>:"Basic Averaged DC-RMS.vi"("error in (no error)"=w2487, "signal in"=w2486) -> ("error out"=w2490:errorcluster, "RMS value"=w2489:dbl)  [unwired: 6 in, 2 out]
              n573 = call "TableHandle.vi"("All"=w2491, "error in (no error)"=w2490, "DataIn"=w2489) -> ("error out"=w2494:errorcluster, "Stop?"=w2492:bool, "StopForLoop"=w2493:bool)  [unwired: 4 in, 2 out]
            }
          }
        }
      }
      frame "SNR" {
        n574 = case shown="真" w2522 {
          tunnel: w2525 -> [w2529 w2539]
          tunnel: w2524 -> [w2530 w2541]
          tunnel: [w2531 w2540] -> w2523
          tunnel: [w2528 w2538] -> w2521
          tunnel: w2520 -> [_ w2537]
          tunnel: w2519 -> [_ w2536]
          tunnel: w2518 -> [_ w2535]
          tunnel: w2517 -> [_ w2534]
          tunnel: w2516 -> [w2526 w2533]
          tunnel: [w2526 w2533] -> w2515
          tunnel: w2512 -> [_ w2532]
          frame False {
            n575 = call "TableHandle.vi"("All"=w2529, "error in (no error)"=w2530, "DataIn"=TRUE) -> ("error out"=w2531:errorcluster, "Stop?"=w2528:bool)  [unwired: 3 in, 4 out]
          }
          frame True {
            n576 = for "For循环" {
              N: w2534 -> [_]
              tunnel: w2541 -> [w2548]
              tunnel: [w2554] -> w2540
              tunnel: w2539 -> [w2551]
              tunnel: [w2552] -> w2538
              tunnel: w2537 -> [w2543]
              tunnel: w2535 -> [_]
              tunnel: w2536 -> [_]
              tunnel: w2533 -> [w2545]
              tunnel: w2532 -> [w2544]
              i -> [w2542]
              stop <- w2553 stop-if-true
              n577 = case shown="1, 默认" w2542 {
                tunnel: w2548 -> [w2566 w2577]
                tunnel: [w2566 w2576] -> w2547
                tunnel: w2544 -> [_ w2575]
                tunnel: w2543 -> [_ w2567]
                tunnel: [w2565 w2573] -> w2546
                tunnel: w2545 -> [w2565 _]
                frame 0 {
                }
                frame 1, Default {
                  n578 = call "GlobalVariable.vi"("Name"="CH", "Slot"=w2567) -> ("String"=w2569:string)  [unwired: 10 in, 3 out]
                  n579 = call "GlobalVariable.vi"("Name"="Para", "Slot"=w2567) -> ("String"=w2568:string)  [unwired: 10 in, 3 out]
                  n580 = Build Array(w2569) -> (w2574:string[])
                  n581 = call "AIs-Freq.vi"("Slot"=w2567, "error in"=w2577, "Mode"=w2568, "CHs"=w2574) -> ("error out"=w2576:errorcluster, "波形图"=w2572:waveform(dbl)[])  [unwired: 5 in, 1 out]
                  n582 = property class="WFGraph (严格)"(reference=w2575, "Value"=w2572, "XScale.Minimum"=0.0 ("X标尺.范围:最小值"), "XScale.Maximum"=0.01 ("X标尺.范围:最大值")) -> ()  [unwired: 1 in, 2 out]
                  n583 = Index Array(array=w2572) -> (element=w2573:waveform(dbl))  [unwired: 1 in]
                }
              }
              n584 = disable-structure shown="启用" {
                disable-tunnel: [w2560 w2564] -> w2550
                disable-tunnel: [w2558 w2562] -> w2549
                disable-tunnel: w2547 -> [w2556 w2564]
                disable-tunnel: w2546 -> [w2555 w2563]
                frame Disabled {
                  n585 = call-poly <vilib>:"Basic Averaged DC-RMS.vi"("reset"=TRUE, "error in (no error)"=w2556, "signal in"=w2555) -> ("error out"=w2560:errorcluster, "RMS value"=w2561:dbl)  [unwired: 5 in, 2 out]
                  n586 = expression code="20*log(x)"(w2561) -> (w2559:dbl)
                  n587 = Absolute Value(x=w2559) -> (abs(x)=w2558:dbl)
                }
                frame Enabled {
                  n588 = call-poly <vilib>:"SINAD Analyzer.vi"("signal in"=w2563) -> ("SINAD (dB)"=w2562:dbl)  [unwired: 5 in, 5 out]
                }
              }
              n589 = call "TableHandle.vi"("All"=w2551, "error in (no error)"=w2550, "DataIn"=w2549) -> ("error out"=w2554:errorcluster, "Stop?"=w2552:bool, "StopForLoop"=w2553:bool)  [unwired: 4 in, 2 out]
            }
          }
        }
      }
      frame "SRSTest" {
        n590 = case shown="真" w2594 {
          tunnel: w2597 -> [w2601 w2613]
          tunnel: w2596 -> [w2602 w2615]
          tunnel: [w2603 w2614] -> w2595
          tunnel: [w2600 w2612] -> w2593
          tunnel: w2592 -> [_ w2611]
          tunnel: w2591 -> [_ w2610]
          tunnel: w2590 -> [_ w2609]
          tunnel: w2589 -> [_ w2608]
          tunnel: w2587 -> [_ _]
          tunnel: w2583 -> [_ w2605]
          tunnel: w2581 -> [w2598 w2607]
          tunnel: w2582 -> [_ w2606]
          tunnel: [w2598 w2604] -> w2580
          frame False {
            n591 = call "TableHandle.vi"("All"=w2601, "error in (no error)"=w2602, "DataIn"=TRUE) -> ("error out"=w2603:errorcluster, "Stop?"=w2600:bool)  [unwired: 3 in, 4 out]
          }
          frame True {
            n592 = for "For循环" {
              N: w2608 -> [_]
              tunnel: w2615 -> [w2625]
              tunnel: [w2643] -> w2614
              tunnel: w2613 -> [w2640]
              tunnel: [w2641] -> w2612
              tunnel: w2611 -> [w2629]
              tunnel: w2609 -> [w2622]
              tunnel: w2610 -> [w2628]
              shift-right: [w2635] -> w2604
              shift-left: w2607 -> [w2638]
              tunnel: w2606 -> [_]
              tunnel: w2605 -> [w2637]
              stop <- w2642 stop-if-true
              n593 = Match Pattern(string=w2622, regular expression=";") -> (before substring=w2619:string, after substring=w2617:string)  [unwired: 1 in, 2 out]
              n594 = Fract/Exp String To Number(string=w2619) -> (number=w2618:dbl)  [unwired: 3 in, 1 out]
              n595 = Fract/Exp String To Number(string=w2617) -> (number=w2616:dbl)  [unwired: 3 in, 1 out]
              n596 = Match Pattern(string=w2628, regular expression=";") -> (before substring=w2627:string, after substring=w2626:string)  [unwired: 1 in, 2 out]
              n597 = case shown="\"Slot2\"" w2629 {
                tunnel: [w2644 w2645] -> w2634
                frame "Slot1", Default {
                  n598 = global read "GlobalValue.vi" "Slot1COM"() -> (w2644:refnum<visa-resource-name>)
                }
                frame "Slot2" {
                  n599 = global read "GlobalValue.vi" "Slot2COM"() -> (w2645:refnum<visa-resource-name>)
                }
              }
              n600 = call "DOWaveAction.vi"("Slot"=w2629, "循环次数"=u32 50, "error in"=w2625, "后段延时"=w2616, "前段延时"=w2618, "CH"=w2626) -> ("error out"=w2624:errorcluster)  [unwired: 5 in]
              n601 = call "CommunicationTool-Ver1.vi"("VISA资源名称"=w2634, "通信协议名称"=w2627, "Slot"=w2629, "error in"=w2624, "Debug"=FALSE) -> ("字符串数值"=w2632:bool, "CMD"=w2630:string, "data"=w2631:string, "error out"=w2633:errorcluster)  [unwired: 5 in, 2 out]
              n602 = Concatenate Strings(w2638, w2630) -> (w2635:string)
              n603 = String Length(string=w2635) -> (length=w2636:i32)
              n604 = property class="Str"(reference=w2637, "Text.Text"=w2635, "Text.Scroll Position"=w2636) -> ()  [unwired: 1 in, 2 out]
              n605 = call "TableHandle.vi"("All"=w2640, "error in (no error)"=w2633, "字符串数值"=w2632, "DataIn"=w2631) -> ("error out"=w2643:errorcluster, "Stop?"=w2641:bool, "StopForLoop"=w2642:bool)  [unwired: 3 in, 2 out]
            }
          }
        }
      }
      frame "Signal" {
        n606 = case shown="真" w2656 {
          tunnel: w2659 -> [w2662 w2670]
          tunnel: w2658 -> [w2663 w2672]
          tunnel: [w2664 w2671] -> w2657
          tunnel: [w2661 w2669] -> w2655
          tunnel: w2654 -> [_ w2668]
          tunnel: w2653 -> [_ w2667]
          tunnel: w2652 -> [_ w2666]
          tunnel: w2651 -> [_ w2665]
          frame False {
            n607 = call "TableHandle.vi"("All"=w2662, "error in (no error)"=w2663, "DataIn"=TRUE) -> ("error out"=w2664:errorcluster, "Stop?"=w2661:bool)  [unwired: 3 in, 4 out]
          }
          frame True {
            n608 = for "For循环" {
              N: w2665 -> [_]
              tunnel: w2672 -> [w2678]
              tunnel: [w2682] -> w2671
              tunnel: w2670 -> [w2679]
              tunnel: [w2680] -> w2669
              tunnel: w2668 -> [w2673]
              tunnel: w2666 -> [w2675]
              tunnel: w2667 -> [w2676]
              stop <- w2681 stop-if-true
              n609 = call "DOFreq.vi"("Slot"=w2673, "error in"=w2678, "State"=w2675, "CH"=w2676) -> ("error out"=w2677:errorcluster)  [unwired: 7 in]
              n610 = call "TableHandle.vi"("All"=w2679, "error in (no error)"=w2677, "DataIn"="Done") -> ("error out"=w2682:errorcluster, "Stop?"=w2680:bool, "StopForLoop"=w2681:bool)  [unwired: 4 in, 2 out]
            }
          }
        }
      }
      frame "StartProcess" {
        n611 = case shown="真" w2698 {
          tunnel: w2701 -> [w2705 w2718]
          tunnel: w2700 -> [w2706 w2720]
          tunnel: [w2707 w2719] -> w2699
          tunnel: [w2704 w2717] -> w2697
          tunnel: w2696 -> [_ w2716]
          tunnel: w2695 -> [_ w2715]
          tunnel: w2694 -> [_ w2714]
          tunnel: w2693 -> [_ w2713]
          tunnel: w2691 -> [_ _]
          tunnel: w2687 -> [_ w2710]
          tunnel: w2685 -> [w2702 w2712]
          tunnel: w2686 -> [_ w2711]
          tunnel: [w2702 w2709] -> w2684
          tunnel: w2683 -> [_ w2708]
          frame False {
            n612 = call "TableHandle.vi"("All"=w2705, "error in (no error)"=w2706, "DataIn"=TRUE) -> ("error out"=w2707:errorcluster, "Stop?"=w2704:bool)  [unwired: 3 in, 4 out]
          }
          frame True {
            n613 = for "For循环" {
              N: w2713 -> [_]
              tunnel: w2720 -> [w2729]
              tunnel: [w2752] -> w2719
              tunnel: w2718 -> [w2749]
              tunnel: [w2750] -> w2717
              tunnel: w2716 -> [w2747]
              tunnel: w2714 -> [w2745]
              tunnel: w2715 -> [w2728]
              shift-right: [w2731] -> w2709
              shift-left: w2712 -> [w2739]
              tunnel: w2711 -> [w2738]
              tunnel: w2710 -> [w2737]
              tunnel: w2708 -> [w2723]
              i -> [w2727]
              stop <- w2751 stop-if-true
              w2724 = "\n"
              n614 = Greater Than 0?(x=w2727) -> (x > 0?=w2726:bool)
              n615 = property class="Ring (严格)"(reference=w2723) -> ("RingText.Text"=w2722:string)  [unwired: 1 in, 2 out]
              n616 = case shown="真" w2726 {
                tunnel: [w2755 w2759] -> w2730
                tunnel: w2729 -> [w2755 w2758]
                tunnel: w2728 -> [_ w2757]
                frame False {
                }
                frame True {
                  n617 = Decimal String To Number(string=w2757) -> (number=w2756:i32)  [unwired: 2 in, 1 out]
                  n618 = flat-sequence {
                    tunnel: [w2761] -> w2759
                    tunnel: w2758 -> [w2761]
                    tunnel: w2756 -> [w2760]
                    frame #0 {
                      n619 = Wait (ms)(milliseconds to wait=w2760) -> ()  [unwired: 1 out]
                    }
                  }
                }
              }
              n620 = case shown="\"1805\", \"1878\", \"1892\"" w2722 {
                tunnel: [enum16{"长安", "江淮"}."长安" ("型号") enum16{"长安", "江淮"}."江淮" ("型号")] -> w2721
                frame "1805", "1878", "1892" {
                }
                frame "1830", "1831", "1832", Default {
                }
              }
              n621 = case shown="\"Slot2\"" w2747 {
                tunnel: [w2762 w2763] -> w2746
                frame "Slot1", Default {
                  n622 = global read "GlobalValue.vi" "Slot1COM"() -> (w2762:refnum<visa-resource-name>)
                }
                frame "Slot2" {
                  n623 = global read "GlobalValue.vi" "Slot2COM"() -> (w2763:refnum<visa-resource-name>)
                }
              }
              n624 = Match Pattern(string=w2745, regular expression=";") -> (before substring=w2743:string, after substring=w2742:string)  [unwired: 1 in, 2 out]
              n625 = Decimal String To Number(string=w2742) -> (number=w2740:i32)  [unwired: 2 in, 1 out]
              n626 = Decimal String To Number(string=w2743) -> (number=w2741:i32)  [unwired: 2 in, 1 out]
              n627 = call "StartProcess.vi"("型号"=w2721, "error in"=w2730, "延时"=w2740, "Cycles"=w2741, "COMIn"=w2746) -> ("error out"=w2748:errorcluster, "连接的字符串"=w2725:string, "OK？"=w2735:bool)  [unwired: 3 in, 1 out]
              n628 = Select(t="：PASS", s=w2735, f="：FAIL") -> (s? t:f=w2732:string)
              n629 = Concatenate Strings(w2739, w2738, w2732, w2724, w2725, w2724) -> (w2731:string)
              n630 = String Length(string=w2731) -> (length=w2736:i32)
              n631 = property class="Str"(reference=w2737, "Text.Text"=w2731, "Text.Scroll Position"=w2736) -> ()  [unwired: 1 in, 2 out]
              n632 = call "TableHandle.vi"("All"=w2749, "error in (no error)"=w2748, "DataIn"=w2735) -> ("error out"=w2752:errorcluster, "Stop?"=w2750:bool, "StopForLoop"=w2751:bool)  [unwired: 4 in, 2 out]
            }
          }
        }
      }
      frame "Static Current" {
        n633 = case shown="真" w2764 {
          tunnel: w2769 -> [w2780 w2788]
          tunnel: w2770 -> [w2781 w2790]
          tunnel: [w2782 w2789] -> w2766
          tunnel: [w2779 w2787] -> w2767
          tunnel: w2768 -> [_ w2786]
          tunnel: w2772 -> [_ w2785]
          tunnel: w2771 -> [_ w2784]
          tunnel: w2773 -> [_ w2783]
          frame False {
            n634 = call "TableHandle.vi"("All"=w2780, "error in (no error)"=w2781, "DataIn"=TRUE) -> ("error out"=w2782:errorcluster, "Stop?"=w2779:bool)  [unwired: 3 in, 4 out]
          }
          frame True {
            n635 = for "For循环" {
              N: w2783 -> [_]
              tunnel: w2790 -> [_]
              tunnel: [w2800] -> w2789
              tunnel: w2788 -> [w2797]
              tunnel: [w2798] -> w2787
              tunnel: w2786 -> [w2796]
              tunnel: w2784 -> [_]
              tunnel: w2785 -> [w2791]
              stop <- w2799 stop-if-true
              w2794 = u16 2 items=["DCV", "ACV", "DCI", "ACI", "OHM", "RST", "CAP", "FRQ", "AUTO"] ("测试类型")
              n636 = case shown="\"Slot1\", 默认" w2796 {
                tunnel: [w2809 w2810] -> w2795
                frame "Slot1", Default {
                  n637 = global read "GlobalValue.vi" "Slot1QCCOM"() -> (w2809:refnum<visa-resource-name>)
                }
                frame "Slot2" {
                  n638 = global read "GlobalValue.vi" "Slot2QCCOM"() -> (w2810:refnum<visa-resource-name>)
                }
              }
              n639 = case shown="\"UT805A\"" w2791 {
                tunnel: w2795 -> [w2804 w2808]
                tunnel: w2794 -> [w2803 w2807]
                tunnel: [w2802 w2806] -> w2793
                tunnel: [w2801 w2805] -> w2792
                frame "GDM8341", Default {
                  n640 = call "Meacurrent8341.vi"("测试类型"=w2803, "VISA资源名称"=w2804) -> ("错误输出"=w2801:errorcluster, "数值"=w2802:dbl)  [unwired: 8 in]
                }
                frame "UT805A" {
                  n641 = call "Meacurrent.vi"("测试类型"=w2807, "VISA资源名称"=w2808) -> ("错误输出"=w2805:errorcluster, "数值"=w2806:dbl)  [unwired: 8 in]
                }
              }
              "错误输出" <- w2792
              n642 = call "TableHandle.vi"("All"=w2797, "DataIn"=w2793) -> ("error out"=w2800:errorcluster, "Stop?"=w2798:bool, "StopForLoop"=w2799:bool)  [unwired: 5 in, 2 out]
            }
          }
        }
      }
      frame "StopTest" {
        # "此步骤不能删除"
      }
      frame "TBD Downloader" {
        n643 = case shown="真" w2832 {
          tunnel: w2835 -> [w2839 w2853]
          tunnel: w2834 -> [w2840 w2855]
          tunnel: [w2841 w2854] -> w2833
          tunnel: [w2838 w2852] -> w2831
          tunnel: w2830 -> [_ w2845]
          tunnel: w2829 -> [_ w2846]
          tunnel: w2828 -> [_ w2851]
          tunnel: w2827 -> [_ w2850]
          tunnel: w2824 -> [_ w2849]
          tunnel: [w2836 w2848] -> w2823
          tunnel: w2822 -> [w2836 w2847]
          tunnel: [w2836 w2844] -> w2820
          tunnel: w2819 -> [_ w2843]
          tunnel: w2818 -> [_ w2842]
          frame False {
            n644 = call "TableHandle.vi"("All"=w2839, "error in (no error)"=w2840, "DataIn"=TRUE) -> ("error out"=w2841:errorcluster, "Stop?"=w2838:bool)  [unwired: 3 in, 4 out]
          }
          frame True {
            n645 = for "For循环" {
              N: w2850 -> [_]
              tunnel: w2855 -> [w2867]
              tunnel: [w2878] -> w2854
              tunnel: w2853 -> [w2875]
              tunnel: [w2876] -> w2852
              tunnel: w2851 -> [w2874]
              tunnel: w2846 -> [w2858]
              tunnel: w2849 -> [w2872]
              shift-right: [w2870] -> w2848
              shift-left: w2847 -> [w2871]
              tunnel: w2845 -> [w2865]
              tunnel: [w2858] -> w2844
              tunnel: w2843 -> [_]
              tunnel: w2842 -> [_]
              i -> [w2868]
              stop <- w2877 stop-if-true
              n646 = Decimal String To Number(string=w2874, default (0L)=u32 0 ("默认(0 I32)")) -> (number=w2866:u32)  [unwired: 1 in, 1 out]
              n647 = case shown="\"Slot2\"" w2865 {
                tunnel: [w2891 w2892] -> w2864
                frame "Slot1", Default {
                  n648 = global read "GlobalValue.vi" "Slot1COM"() -> (w2891:refnum<visa-resource-name>)
                }
                frame "Slot2" {
                  n649 = global read "GlobalValue.vi" "Slot2COM"() -> (w2892:refnum<visa-resource-name>)
                }
              }
              n650 = case shown="1, 默认" w2868 {
                tunnel: w2867 -> [w2893 w2896]
                tunnel: [w2893 w2895] -> w2861
                tunnel: w2866 -> [_ w2894]
                frame 0 {
                }
                frame 1, Default {
                  n651 = call "WaitTimes.vi"("WaitTimes"=w2894, "error in (no error)"=w2896) -> ("error out"=w2895:errorcluster)  [unwired: 9 in]
                }
              }
              n652 = String To Path(string=w2858) -> (path=w2860:path)
              n653 = call <vilib>:"Check if File or Folder Exists.vi"("error in (no error)"=w2861, "path"=w2860) -> ("error out"=w2857:errorcluster, "file or folder exists?"=w2859:bool)  [unwired: 7 in, 1 out]
              n654 = case shown="真" w2859 {
                tunnel: w2864 -> [_ w2890]
                tunnel: [FALSE ("Result") w2889] -> w2863
                tunnel: [w2883 w2888] -> w2862
                tunnel: w2858 -> [w2880 w2887]
                tunnel: w2857 -> [w2882 w2886]
                tunnel: "TBC文件未找到！\n" ("消息") -> [w2881 _]
                frame False {
                  n655 = Concatenate Strings(w2881, w2880) -> (w2879:string)
                  n656 = call <vilib>:"Clear Errors.vi"("error in (no error)"=w2882) -> ("error out"=w2883:errorcluster)  [unwired: 6 in]
                  n657 = One Button Dialog(message=w2879) -> ()  [unwired: 1 in, 1 out]
                }
                frame True {
                  n658 = call <vilib>:"Clear Errors.vi"("error in (no error)"=w2886) -> ("error out"=w2885:errorcluster)  [unwired: 6 in]
                  n659 = call "Download1 TBD file.vi"("error in (no error)"=w2885, "TBC File link"=w2887, "VISA资源名称"=w2890) -> ("错误输出"=w2888:errorcluster, "Result"=w2889:bool)  [unwired: 6 in, 1 out]
                }
              }
              n660 = Concatenate Strings(w2871) -> (w2870:string)
              n661 = String Length(string=w2870) -> (length=w2869:i32)
              n662 = call "TableHandle.vi"("All"=w2875, "error in (no error)"=w2862, "DataIn"=w2863) -> ("error out"=w2878:errorcluster, "Stop?"=w2876:bool, "StopForLoop"=w2877:bool)  [unwired: 4 in, 2 out]
              n663 = property class="Str"(reference=w2872, "Text.Text"=w2870, "Text.Scroll Position"=w2869) -> ()  [unwired: 1 in, 2 out]
            }
          }
        }
      }
      frame "THD" {
        n664 = case shown="真" w2909 {
          tunnel: w2912 -> [w2916 w2926]
          tunnel: w2911 -> [w2917 w2928]
          tunnel: [w2918 w2927] -> w2910
          tunnel: [w2915 w2925] -> w2908
          tunnel: w2907 -> [_ w2924]
          tunnel: w2906 -> [_ w2923]
          tunnel: w2905 -> [_ w2922]
          tunnel: w2904 -> [_ w2921]
          tunnel: w2903 -> [w2913 w2920]
          tunnel: [w2913 w2920] -> w2902
          tunnel: w2899 -> [_ w2919]
          frame False {
            n665 = call "TableHandle.vi"("All"=w2916, "error in (no error)"=w2917, "DataIn"=TRUE) -> ("error out"=w2918:errorcluster, "Stop?"=w2915:bool)  [unwired: 3 in, 4 out]
          }
          frame True {
            n666 = for "For循环" {
              N: w2921 -> [_]
              tunnel: w2928 -> [w2935]
              tunnel: [w2942] -> w2927
              tunnel: w2926 -> [w2933]
              tunnel: [w2940] -> w2925
              tunnel: w2924 -> [w2931]
              tunnel: w2922 -> [_]
              tunnel: w2923 -> [_]
              tunnel: w2920 -> [w2929]
              tunnel: w2919 -> [w2932]
              i -> [w2936]
              stop <- w2941 stop-if-true
              n667 = case shown="0" w2936 {
                tunnel: w2935 -> [w2944 w2955]
                tunnel: [w2944 w2954] -> w2934
                tunnel: w2932 -> [_ w2953]
                tunnel: w2931 -> [_ w2949]
                tunnel: [w2943 w2950] -> w2930
                tunnel: w2929 -> [w2943 _]
                frame 0 {
                }
                frame 1, Default {
                  n668 = call "GlobalVariable.vi"("Name"="CH", "Slot"=w2949) -> ("String"=w2948:string)  [unwired: 10 in, 3 out]
                  n669 = call "GlobalVariable.vi"("Name"="Para", "Slot"=w2949) -> ("String"=w2947:string)  [unwired: 10 in, 3 out]
                  n670 = Build Array(w2948) -> (w2952:string[])
                  n671 = call "AIs-Freq.vi"("Slot"=w2949, "error in"=w2955, "Mode"=w2947, "CHs"=w2952) -> ("error out"=w2954:errorcluster, "波形图"=w2951:waveform(dbl)[])  [unwired: 5 in, 1 out]
                  n672 = property class="WFGraph (严格)"(reference=w2953, "Value"=w2951, "XScale.Minimum"=0.0 ("X标尺.范围:最小值"), "XScale.Maximum"=0.01 ("X标尺.范围:最大值")) -> ()  [unwired: 1 in, 2 out]
                  n673 = Index Array(array=w2951) -> (element=w2950:waveform(dbl))  [unwired: 1 in]
                }
              }
              n674 = call-poly <vilib>:"SVT THD+N.vi"("scaled signal [EU]"=w2930, "error in (no error)"=w2934, "desired units"=T6 {"THD+N units"=enum."%", "detected fundamental amplitude units"=enum."EU rms"}) -> ("THD+N"=w2937:dbl, "error out"=w2939:errorcluster)  [unwired: 11 in, 4 out]
              n675 = call "TableHandle.vi"("All"=w2933, "error in (no error)"=w2939, "DataIn"=w2937) -> ("error out"=w2942:errorcluster, "Stop?"=w2940:bool, "StopForLoop"=w2941:bool)  [unwired: 4 in, 2 out]
            }
          }
        }
      }
      frame "USBCMD" {
        n676 = case shown="真" w2971 {
          tunnel: w2974 -> [w2979 w2992]
          tunnel: w2973 -> [w2980 w2994]
          tunnel: [w2981 w2993] -> w2972
          tunnel: [w2978 w2991] -> w2970
          tunnel: w2969 -> [_ w2984]
          tunnel: w2968 -> [_ w2985]
          tunnel: w2967 -> [_ w2990]
          tunnel: w2966 -> [_ w2989]
          tunnel: w2963 -> [_ w2988]
          tunnel: [w2976 w2987] -> w2962
          tunnel: w2961 -> [w2976 w2986]
          tunnel: [w2975 w2983] -> w2960
          tunnel: w2959 -> [w2975 w2982]
          frame False {
            n677 = call "TableHandle.vi"("All"=w2979, "error in (no error)"=w2980, "DataIn"=TRUE) -> ("error out"=w2981:errorcluster, "Stop?"=w2978:bool)  [unwired: 3 in, 4 out]
          }
          frame True {
            n678 = for "For循环" {
              N: w2989 -> [_]
              tunnel: w2994 -> [w3009]
              tunnel: [w3022] -> w2993
              tunnel: w2992 -> [w3019]
              tunnel: [w3020] -> w2991
              tunnel: w2990 -> [w3017]
              tunnel: w2985 -> [w3001]
              tunnel: w2988 -> [w3015]
              shift-right: [w3013] -> w2987
              shift-left: w2986 -> [w3014]
              tunnel: w2984 -> [w2996]
              tunnel: [w3003] -> w2983
              tunnel: w2982 -> [w3002]
              i -> [w3010]
              stop <- w3021 stop-if-true
              n679 = case shown="\"Slot1\", 默认" w2996 {
                tunnel: [w3049 w3052] -> w3000
                tunnel: [w3050 w3051] -> w3004
                frame "Slot1", Default {
                  n680 = global read "GlobalValue.vi" "Slot1USBCOM"() -> (w3049:refnum<visa-resource-name>)
                  n681 = global read "GlobalValue.vi" "Slot1USB"() -> (w3050:string)
                }
                frame "Slot2" {
                  n682 = global read "GlobalValue.vi" "Slot2USBCOM"() -> (w3052:refnum<visa-resource-name>)
                  n683 = global read "GlobalValue.vi" "Slot2USB"() -> (w3051:string)
                }
              }
              n684 = Decimal String To Number(string=w3017, default (0L)=u32 0 ("默认(0 I32)")) -> (number=w3007:u32)  [unwired: 1 in, 1 out]
              n685 = case shown="1, 默认" w3010 {
                tunnel: w3009 -> [w3053 w3056]
                tunnel: [w3053 w3055] -> w3008
                tunnel: w3007 -> [_ w3054]
                frame 0 {
                }
                frame 1, Default {
                  n686 = call "WaitTimes.vi"("WaitTimes"=w3054, "error in (no error)"=w3056) -> ("error out"=w3055:errorcluster)  [unwired: 9 in]
                }
              }
              n687 = Empty String/Path?(string/path=w3000) -> (empty?=w3006:bool)
              n688 = case shown="真" w3006 {
                tunnel: [w3046 w3048] -> w3005
                tunnel: w3004 -> [_ w3047]
                tunnel: w3000 -> [w3046 _]
                frame False {
                }
                frame True {
                  n689 = call "SearchUSB.vi"("USB"=w3047) -> ("USBPort"=w3048:refnum<visa-resource-name>)  [unwired: 9 in, 1 out]
                }
              }
              n690 = call "SIMCOMCommunicationTool.vi"("Slot"=w2996, "Debug"=FALSE, "MEID"=w3002, "error in"=w3008, "DelayTime"=w3007, "通信协议名称"=w3001, "VISA资源名称"=w3005) -> ("error out"=w3018:errorcluster, "ReturnData"=w2997:string, "反馈结果"=w2999:bool, "字符串数值"=w2995:bool, "CMD"=w2998:string)
              n691 = Concatenate Strings(w3014, w2998) -> (w3013:string)
              n692 = String Length(string=w3013) -> (length=w3012:i32)
              n693 = case shown="\"假\", 默认" w3001 {
                tunnel: [w3036 w3037 w3042] -> w3003
                tunnel: w2997 -> [_ w3038 w3042]
                tunnel: w3002 -> [w3036 w3037 _]
                tunnel: w2996 -> [_ w3039 w3043]
                frame "假", Default {
                }
                frame "查询ESN" {
                  n694 = case shown="\"Slot2\"" w3039 {
                    tunnel: w3038 -> [w3040 w3041]
                    frame "Slot1", Default {
                      n695 = global write "GlobalValue.vi" "Slot1ESN"(w3040) -> ()
                    }
                    frame "Slot2" {
                      n696 = global write "GlobalValue.vi" "Slot2ESN"(w3041) -> ()
                    }
                  }
                }
                frame "查询MEID" {
                  n697 = case shown="\"Slot1\", 默认" w3043 {
                    tunnel: w3042 -> [w3044 w3045]
                    frame "Slot1", Default {
                      n698 = global write "GlobalValue.vi" "Slot1MEID"(w3044) -> ()
                    }
                    frame "Slot2" {
                      n699 = global write "GlobalValue.vi" "Slot2MEID"(w3045) -> ()
                    }
                  }
                }
              }
              n700 = case shown="假" w2999 {
                tunnel: [w3028 w3035] -> w3022
                tunnel: [w3026 w3034] -> w3021
                tunnel: [w3025 w3033] -> w3020
                tunnel: w3019 -> [w3029 w3032]
                tunnel: w3018 -> [w3027 w3031]
                tunnel: w2999 -> [_ w3030]
                tunnel: w2997 -> [w3024 _]
                tunnel: w2995 -> [w3023 _]
                frame False {
                  n701 = call "TableHandle.vi"("All"=w3029, "error in (no error)"=w3027, "字符串数值"=w3023, "DataIn"=w3024) -> ("error out"=w3028:errorcluster, "Stop?"=w3025:bool, "StopForLoop"=w3026:bool)  [unwired: 3 in, 2 out]
                }
                frame True {
                  n702 = call "TableHandle.vi"("All"=w3032, "error in (no error)"=w3031, "DataIn"=w3030) -> ("error out"=w3035:errorcluster, "Stop?"=w3033:bool, "StopForLoop"=w3034:bool)  [unwired: 4 in, 2 out]
                }
              }
              n703 = property class="Str"(reference=w3015, "Text.Text"=w3013, "Text.Scroll Position"=w3012) -> ()  [unwired: 1 in, 2 out]
            }
          }
        }
      }
      frame "USBCMD_CF" {
        n704 = case shown="真" w3071 {
          tunnel: w3074 -> [w3079 w3093]
          tunnel: w3073 -> [w3080 w3095]
          tunnel: [w3081 w3094] -> w3072
          tunnel: [w3078 w3092] -> w3070
          tunnel: w3069 -> [_ w3085]
          tunnel: w3068 -> [_ w3086]
          tunnel: w3067 -> [_ w3091]
          tunnel: w3066 -> [_ w3090]
          tunnel: w3063 -> [_ w3089]
          tunnel: [w3076 w3088] -> w3062
          tunnel: w3061 -> [w3076 w3087]
          tunnel: [w3075 w3084] -> w3060
          tunnel: w3059 -> [w3075 w3083]
          tunnel: w3057 -> [_ w3082]
          frame False {
            n705 = call "TableHandle.vi"("All"=w3079, "error in (no error)"=w3080, "DataIn"=TRUE) -> ("error out"=w3081:errorcluster, "Stop?"=w3078:bool)  [unwired: 3 in, 4 out]
          }
          frame True {
            n706 = for "For循环" {
              N: w3090 -> [_]
              tunnel: w3095 -> [w3111]
              tunnel: [w3124] -> w3094
              tunnel: w3093 -> [w3121]
              tunnel: [w3122] -> w3092
              tunnel: w3091 -> [w3119]
              tunnel: w3086 -> [w3096]
              tunnel: w3089 -> [w3117]
              shift-right: [w3115] -> w3088
              shift-left: w3087 -> [w3116]
              tunnel: w3085 -> [w3099]
              tunnel: [w3105] -> w3084
              tunnel: w3083 -> [w3104]
              tunnel: w3082 -> [w3097]
              i -> [w3112]
              stop <- w3123 stop-if-true
              # "如果前面不能获取端口，此处直接让它FAIL"
              n707 = Decimal String To Number(string=w3119, default (0L)=u32 0 ("默认(0 I32)")) -> (number=w3109:u32)  [unwired: 1 in, 1 out]
              n708 = case shown="\"Slot1\", 默认" w3099 {
                tunnel: [w3165 w3168] -> w3103
                tunnel: [w3166 w3167] -> w3106
                frame "Slot1", Default {
                  n709 = global read "GlobalValue.vi" "Slot1USBCOM DY"() -> (w3165:refnum<visa-resource-name>)
                  n710 = global read "GlobalValue.vi" "Slot1USB"() -> (w3166:string)
                }
                frame "Slot2" {
                  n711 = global read "GlobalValue.vi" "Slot2USBCOM DY"() -> (w3168:refnum<visa-resource-name>)
                  n712 = global read "GlobalValue.vi" "Slot2USB"() -> (w3167:string)
                }
              }
              n713 = case shown="1, 默认" w3112 {
                tunnel: w3111 -> [w3169 w3172]
                tunnel: [w3169 w3171] -> w3110
                tunnel: w3109 -> [_ w3170]
                frame 0 {
                }
                frame 1, Default {
                  n714 = call "WaitTimes.vi"("WaitTimes"=w3170, "error in (no error)"=w3172) -> ("error out"=w3171:errorcluster)  [unwired: 9 in]
                }
              }
              n715 = Empty String/Path?(string/path=w3103) -> (empty?=w3108:bool)
              n716 = case shown="真" w3108 {
                tunnel: [w3163 w3164] -> w3107
                tunnel: w3106 -> [_ _]
                tunnel: w3103 -> [w3163 w3164]
                frame False {
                }
                frame True {
                }
              }
              n717 = call "SIMCOMCommunicationTool_CF.vi"("VISA资源名称"=w3107, "MSComm"=w3097, "MEID"=w3104, "通信协议名称"=w3096, "DelayTime"=w3109, "error in"=w3110, "Debug"=FALSE, "Slot"=w3099) -> ("CMD"=w3101:string, "字符串数值"=w3098:bool, "反馈结果"=w3102:bool, "ReturnData"=w3100:string, "error out"=w3120:errorcluster)  [unwired: 3 in]
              n718 = Concatenate Strings(w3116, w3101) -> (w3115:string)
              n719 = String Length(string=w3115) -> (length=w3114:i32)
              n720 = case shown="\"查询ESN\"" w3096 {
                tunnel: [w3153 w3154 w3159] -> w3105
                tunnel: w3100 -> [_ w3155 w3159]
                tunnel: w3104 -> [w3153 w3154 _]
                tunnel: w3099 -> [_ w3156 w3160]
                frame "假", Default {
                }
                frame "查询ESN" {
                  n721 = case shown="\"Slot2\"" w3156 {
                    tunnel: w3155 -> [w3157 w3158]
                    frame "Slot1", Default {
                      n722 = global write "GlobalValue.vi" "Slot1ESN"(w3157) -> ()
                    }
                    frame "Slot2" {
                      n723 = global write "GlobalValue.vi" "Slot2ESN"(w3158) -> ()
                    }
                  }
                }
                frame "查询MEID" {
                  n724 = case shown="\"Slot1\", 默认" w3160 {
                    tunnel: w3159 -> [w3161 w3162]
                    frame "Slot1", Default {
                      n725 = global write "GlobalValue.vi" "Slot1MEID"(w3161) -> ()
                    }
                    frame "Slot2" {
                      n726 = global write "GlobalValue.vi" "Slot2MEID"(w3162) -> ()
                    }
                  }
                }
              }
              n727 = case shown="\"H330CSQ\"" w3096 {
                tunnel: [w3132 w3147] -> w3124
                tunnel: [w3131 w3149] -> w3123
                tunnel: [w3130 w3148] -> w3122
                tunnel: w3121 -> [w3129 w3152]
                tunnel: w3120 -> [w3128 w3146]
                tunnel: w3102 -> [w3127 _]
                tunnel: w3100 -> [w3126 w3150]
                tunnel: w3098 -> [w3125 _]
                frame "假", Default {
                  n728 = case shown="真" w3127 {
                    tunnel: [w3138 w3145] -> w3132
                    tunnel: [w3136 w3144] -> w3131
                    tunnel: [w3135 w3143] -> w3130
                    tunnel: w3129 -> [w3139 w3142]
                    tunnel: w3128 -> [w3137 w3141]
                    tunnel: w3127 -> [_ w3140]
                    tunnel: w3126 -> [w3134 _]
                    tunnel: w3125 -> [w3133 _]
                    frame False {
                      n729 = call "TableHandle.vi"("All"=w3139, "error in (no error)"=w3137, "字符串数值"=w3133, "DataIn"=w3134) -> ("error out"=w3138:errorcluster, "Stop?"=w3135:bool, "StopForLoop"=w3136:bool)  [unwired: 3 in, 2 out]
                    }
                    frame True {
                      n730 = call "TableHandle.vi"("All"=w3142, "error in (no error)"=w3141, "DataIn"=w3140) -> ("error out"=w3145:errorcluster, "Stop?"=w3143:bool, "StopForLoop"=w3144:bool)  [unwired: 4 in, 2 out]
                    }
                  }
                }
                frame "H330CSQ" {
                  n731 = call "TableHandle.vi"("All"=w3152, "error in (no error)"=w3146, "字符串数值"=TRUE, "DataIn"=w3150) -> ("error out"=w3147:errorcluster, "Stop?"=w3148:bool, "StopForLoop"=w3149:bool)  [unwired: 3 in, 2 out]
                }
              }
              n732 = property class="Str"(reference=w3117, "Text.Text"=w3115, "Text.Scroll Position"=w3114) -> ()  [unwired: 1 in, 2 out]
            }
          }
        }
      }
      frame "USBCMD_CF_VB" {
        n733 = case shown="真" w3187 {
          tunnel: w3190 -> [w3195 w3209]
          tunnel: w3189 -> [w3196 w3211]
          tunnel: [w3197 w3210] -> w3188
          tunnel: [w3194 w3208] -> w3186
          tunnel: w3185 -> [_ w3201]
          tunnel: w3184 -> [_ w3202]
          tunnel: w3183 -> [_ w3207]
          tunnel: w3182 -> [_ w3206]
          tunnel: w3179 -> [_ w3205]
          tunnel: [w3192 w3204] -> w3178
          tunnel: w3177 -> [w3192 w3203]
          tunnel: [w3191 w3200] -> w3176
          tunnel: w3175 -> [w3191 w3199]
          tunnel: w3173 -> [_ w3198]
          frame False {
            n734 = call "TableHandle.vi"("All"=w3195, "error in (no error)"=w3196, "DataIn"=TRUE) -> ("error out"=w3197:errorcluster, "Stop?"=w3194:bool)  [unwired: 3 in, 4 out]
          }
          frame True {
            n735 = for "For循环" {
              N: w3206 -> [_]
              tunnel: w3211 -> [w3227]
              tunnel: [w3240] -> w3210
              tunnel: w3209 -> [w3237]
              tunnel: [w3238] -> w3208
              tunnel: w3207 -> [w3235]
              tunnel: w3202 -> [w3219]
              tunnel: w3205 -> [w3233]
              shift-right: [w3231] -> w3204
              shift-left: w3203 -> [w3232]
              tunnel: w3201 -> [w3214]
              tunnel: [w3221] -> w3200
              tunnel: w3199 -> [w3220]
              tunnel: w3198 -> [w3212]
              i -> [w3228]
              stop <- w3239 stop-if-true
              n736 = case shown="\"Slot1\", 默认" w3214 {
                tunnel: [w3267 w3270] -> w3218
                tunnel: [w3268 w3269] -> w3222
                frame "Slot1", Default {
                  n737 = global read "GlobalValue.vi" "Slot1USBCOM"() -> (w3267:refnum<visa-resource-name>)
                  n738 = global read "GlobalValue.vi" "Slot1USB"() -> (w3268:string)
                }
                frame "Slot2" {
                  n739 = global read "GlobalValue.vi" "Slot2USBCOM"() -> (w3270:refnum<visa-resource-name>)
                  n740 = global read "GlobalValue.vi" "Slot2USB"() -> (w3269:string)
                }
              }
              n741 = Decimal String To Number(string=w3235, default (0L)=u32 0 ("默认(0 I32)")) -> (number=w3225:u32)  [unwired: 1 in, 1 out]
              n742 = case shown="1, 默认" w3228 {
                tunnel: w3227 -> [w3271 w3274]
                tunnel: [w3271 w3273] -> w3226
                tunnel: w3225 -> [_ w3272]
                frame 0 {
                }
                frame 1, Default {
                  n743 = call "WaitTimes.vi"("WaitTimes"=w3272, "error in (no error)"=w3274) -> ("error out"=w3273:errorcluster)  [unwired: 9 in]
                }
              }
              n744 = Empty String/Path?(string/path=w3218) -> (empty?=w3224:bool)
              n745 = case shown="真" w3224 {
                tunnel: [w3264 w3266] -> w3223
                tunnel: w3222 -> [_ w3265]
                tunnel: w3218 -> [w3264 _]
                frame False {
                }
                frame True {
                  n746 = call "SearchUSB_CF.vi"("USB"=w3265) -> ("USBPort"=w3266:refnum<visa-resource-name>)  [unwired: 9 in, 1 out]
                }
              }
              n747 = call "SIMCOMCommunicationTool_CF_vb.vi"("VISA资源名称"=w3223, "MSComm"=w3212, "MEID"=w3220, "通信协议名称"=w3219, "DelayTime"=w3225, "error in"=w3226, "Debug"=FALSE, "Slot"=w3214) -> ("CMD"=w3216:string, "字符串数值"=w3213:bool, "反馈结果"=w3217:bool, "ReturnData"=w3215:string, "error out"=w3236:errorcluster)  [unwired: 3 in]
              n748 = Concatenate Strings(w3232, w3216) -> (w3231:string)
              n749 = String Length(string=w3231) -> (length=w3230:i32)
              n750 = case shown="\"查询ESN\"" w3219 {
                tunnel: [w3254 w3255 w3260] -> w3221
                tunnel: w3215 -> [_ w3256 w3260]
                tunnel: w3220 -> [w3254 w3255 _]
                tunnel: w3214 -> [_ w3257 w3261]
                frame "假", Default {
                }
                frame "查询ESN" {
                  n751 = case shown="\"Slot1\", 默认" w3257 {
                    tunnel: w3256 -> [w3258 w3259]
                    frame "Slot1", Default {
                      n752 = global write "GlobalValue.vi" "Slot1ESN"(w3258) -> ()
                    }
                    frame "Slot2" {
                      n753 = global write "GlobalValue.vi" "Slot2ESN"(w3259) -> ()
                    }
                  }
                }
                frame "查询MEID" {
                  n754 = case shown="\"Slot1\", 默认" w3261 {
                    tunnel: w3260 -> [w3262 w3263]
                    frame "Slot1", Default {
                      n755 = global write "GlobalValue.vi" "Slot1MEID"(w3262) -> ()
                    }
                    frame "Slot2" {
                      n756 = global write "GlobalValue.vi" "Slot2MEID"(w3263) -> ()
                    }
                  }
                }
              }
              n757 = case shown="假" w3217 {
                tunnel: [w3246 w3253] -> w3240
                tunnel: [w3244 w3252] -> w3239
                tunnel: [w3243 w3251] -> w3238
                tunnel: w3237 -> [w3247 w3250]
                tunnel: w3236 -> [w3245 w3249]
                tunnel: w3217 -> [_ w3248]
                tunnel: w3215 -> [w3242 _]
                tunnel: w3213 -> [w3241 _]
                frame False {
                  n758 = call "TableHandle.vi"("All"=w3247, "error in (no error)"=w3245, "字符串数值"=w3241, "DataIn"=w3242) -> ("error out"=w3246:errorcluster, "Stop?"=w3243:bool, "StopForLoop"=w3244:bool)  [unwired: 3 in, 2 out]
                }
                frame True {
                  n759 = call "TableHandle.vi"("All"=w3250, "error in (no error)"=w3249, "DataIn"=w3248) -> ("error out"=w3253:errorcluster, "Stop?"=w3251:bool, "StopForLoop"=w3252:bool)  [unwired: 4 in, 2 out]
                }
              }
              n760 = property class="Str"(reference=w3233, "Text.Text"=w3231, "Text.Scroll Position"=w3230) -> ()  [unwired: 1 in, 2 out]
            }
          }
        }
      }
      frame "UpdateData" {
        n761 = case shown="真" w3285 {
          tunnel: w3288 -> [w3291 w3299]
          tunnel: w3287 -> [w3292 w3301]
          tunnel: [w3293 w3300] -> w3286
          tunnel: [w3290 w3298] -> w3284
          tunnel: w3283 -> [_ w3297]
          tunnel: w3282 -> [_ w3296]
          tunnel: w3281 -> [_ w3295]
          tunnel: w3280 -> [_ w3294]
          frame False {
            n762 = call "TableHandle.vi"("All"=w3291, "error in (no error)"=w3292, "DataIn"=TRUE) -> ("error out"=w3293:errorcluster, "Stop?"=w3290:bool)  [unwired: 3 in, 4 out]
          }
          frame True {
            n763 = for "For循环" {
              N: w3294 -> [_]
              tunnel: w3301 -> [w3304]
              tunnel: [w3326] -> w3300
              tunnel: w3299 -> [w3323]
              tunnel: [w3324] -> w3298
              tunnel: w3297 -> [w3317]
              tunnel: w3295 -> [_]
              tunnel: w3296 -> [_]
              stop <- w3325 stop-if-true
              n764 = Format Date/Time String(time format string (%c)="%Y/%m/%d %H:%M:%S " ("时间格式字符串(%c)")) -> (date/time string=w3309:string)  [unwired: 2 in]
              n765 = call "ccidinfo-r.vi"("Data Type"=PDINFO."TUID", "Slot"=w3317) -> ("Data"=w3312:string)
              n766 = call "ccidinfo-r.vi"("Data Type"=PDINFO."HW Ver", "Slot"=w3317) -> ("Data"=w3311:string)
              n767 = call "ccidinfo-r.vi"("Data Type"=PDINFO."Fw Ver", "Slot"=w3317) -> ("Data"=w3310:string)
              n768 = call "ccidinfo-r.vi"("Data Type"=PDINFO."SN", "Slot"=w3317) -> ("Data"=w3308:string)
              n769 = call "ccidinfo-r.vi"("Data Type"=PDINFO."CCID", "Slot"=w3317) -> ("Data"=w3306:string)
              n770 = call "ccidinfo-r.vi"("Data Type"=PDINFO."CertifID", "Slot"=w3317) -> ("Data"=w3307:string)
              n771 = Build Array("TBOX", "7900020-CC102", w3312, w3311, w3310, w3309, w3308, w3307, w3306) -> (w3305:string[])
              n772 = call "Writer data.vi"("error in"=w3304, "数据输入"=w3305, "Slot"=w3317) -> ("error out"=w3303:errorcluster, "Pass?"=w3302:bool)  [unwired: 6 in, 1 out]
              n773 = call "TableHandle.vi"("All"=w3323, "error in (no error)"=w3303, "DataIn"=w3302) -> ("error out"=w3326:errorcluster, "Stop?"=w3324:bool, "StopForLoop"=w3325:bool)  [unwired: 4 in, 2 out]
            }
          }
        }
      }
      frame "WDataToDB" {
        # "1、型号区分数据入库新库或旧库\n2、TestName区分新库入库的步骤\n3、通道与参数配合使用输入各步骤入库参数\n4、读TUID、Certid不正确终止测试\n5、Reserved3保存的是MAC地址"
        n774 = case shown="真" w3332 {
          tunnel: w3342 -> [_ w3365]
          tunnel: w3341 -> [_ w3364]
          tunnel: [w3347 w3363] -> w3340
          tunnel: [w3349 w3362] -> w3339
          tunnel: w3337 -> [w3351 w3361]
          tunnel: w3336 -> [_ w3360]
          tunnel: w3335 -> [_ w3355]
          tunnel: w3334 -> [_ w3359]
          tunnel: w3333 -> [_ w3358]
          tunnel: w3331 -> [w3348 _]
          tunnel: w3330 -> [_ w3357]
          tunnel: w3327 -> [w3346 w3356]
          tunnel: [w3346 w3354] -> w3329
          tunnel: w3328 -> [_ w3353]
          tunnel: w3327 -> [_ w3352]
          frame False {
            n775 = call "TableHandle.vi"("All"=w3351, "error in (no error)"=w3348, "DataIn"=TRUE ("字符串数值")) -> ("error out"=w3347:errorcluster, "Stop?"=w3349:bool)  [unwired: 4 in, 3 out]
          }
          frame True {
            n776 = for {
              N: w3353 -> [_]
              tunnel: w3365 -> [w3392]
              tunnel: w3364 -> [w3366]
              tunnel: [w3391] -> w3363
              tunnel: [w3390] -> w3362
              tunnel: w3361 -> [w3388]
              tunnel: w3360 -> [w3384]
              tunnel: w3359 -> [w3382]
              tunnel: w3358 -> [w3381]
              tunnel: w3357 -> [w3379]
              tunnel: w3356 -> [_]
              tunnel: w3355 -> [w3378]
              shift-right: [w3375] -> w3354
              shift-left: w3352 -> [w3372]
              stop <- w3373 stop-if-true
              w3368 = "\n"
              n777 = property class="Ring (严格)"(reference=w3384) -> ("RingText.Text"=w3383:string)  [unwired: 1 in, 2 out]
              n778 = case shown="\"Slot2\"" w3366 {
                tunnel: [w3393 w3394] -> w3387
                frame "Slot1", Default {
                  n779 = global read "GlobalValue.vi" "SN1 Result"() -> (w3393:bool)
                }
                frame "Slot2" {
                  n780 = global read "GlobalValue.vi" "SN2 Result"() -> (w3394:bool)
                }
              }
              n781 = property class="Str"(reference=w3381) -> ("Value"=w3380:string)  [unwired: 1 in, 2 out]
              n782 = case shown="\"1805\", \"1830\", \"1831\", \"1832\", 默认" w3383 {
                selector: w3383 -> [_ w3430]
                tunnel: w3392 -> [w3403 w3441]
                tunnel: w3366 -> [w3402 w3440]
                tunnel: w3381 -> [w3401 w3439]
                tunnel: [w3400 w3438] -> w3376
                tunnel: [w3399 w3437] -> w3389
                tunnel: w3388 -> [w3398 w3436]
                tunnel: w3387 -> [w3397 w3435]
                tunnel: [w3396 w3434] -> w3386
                tunnel: w3384 -> [w3395 w3433]
                tunnel: w3378 -> [_ w3432]
                tunnel: w3382 -> [_ w3431]
                tunnel: w3380 -> [_ w3429]
                tunnel: [_ w3428] -> w3371
                tunnel: [_ w3427] -> w3370
                tunnel: [_ w3426] -> w3369
                tunnel: [_ w3425] -> w3367
                frame "1602", "1704", "1716", "1802", "1858" {
                  n783 = case shown="真" w3397 {
                    tunnel: w3403 -> [_ w3416]
                    tunnel: w3402 -> [_ w3410]
                    tunnel: w3395 -> [_ w3415]
                    tunnel: w3401 -> [_ w3414]
                    tunnel: ["SN FAIL" ("ResultA") w3412] -> w3400
                    tunnel: [w3406 w3413] -> w3399
                    tunnel: w3398 -> [w3406 w3413]
                    tunnel: [errorcluster {"status"=FALSE, "code"=0, "source"=""} ("错误输出") w3408] -> w3396
                    frame False {
                    }
                    frame True {
                      n784 = flat-sequence {
                        tunnel: w3416 -> [w3423]
                        tunnel: w3415 -> [w3422]
                        tunnel: w3414 -> [w3421]
                        tunnel: [w3420] -> w3412
                        tunnel: w3410 -> [w3417]
                        tunnel: [w3419] -> w3409
                        tunnel: [w3418] -> w3408
                        tunnel: [w3417] -> w3407
                        frame #0 {
                          n785 = xnode "错误下拉列表"() -> ("错误输出"=w3418:errorcluster)
                          n786 = call "WriteDataToDB.vi"("通信协议名称"=w3423, "SN"=w3421, "产品型号"=w3422, "Slot"=w3417) -> ("ResultA"=w3420:string, "FSNA"=w3419:string)  [unwired: 6 in]
                        }
                      }
                      n787 = call "ccidinfo-w.vi"("Data"=w3409, "Data Type"=PDINFO."DevID", "Slot"=w3407) -> ()  [unwired: 1 in]
                    }
                  }
                }
                frame "1805", "1830", "1831", "1832", Default {
                  n788 = case shown="真" w3435 {
                    tunnel: w3441 -> [_ w3454]
                    tunnel: w3440 -> [_ w3450]
                    tunnel: w3433 -> [_ _]
                    tunnel: w3439 -> [_ _]
                    tunnel: ["SN FAIL" ("ResultA") w3453] -> w3438
                    tunnel: [w3444 w3456] -> w3437
                    tunnel: w3436 -> [w3444 w3456]
                    tunnel: [errorcluster {"status"=FALSE, "code"=0, "source"=""} ("错误输出") _] -> w3434
                    tunnel: w3432 -> [_ w3455]
                    tunnel: w3431 -> [_ w3452]
                    tunnel: w3430 -> [_ w3451]
                    tunnel: w3429 -> [_ w3449]
                    tunnel: [_ w3448] -> w3428
                    tunnel: [_ w3447] -> w3427
                    tunnel: [_ w3446] -> w3426
                    tunnel: [_ w3445] -> w3425
                    frame False {
                    }
                    frame True {
                      n789 = case shown="\"比较IMSI号\"" w3455 {
                        tunnel: w3454 -> [_ w3465 _ _ _ _]
                        tunnel: [_ w3462 w3471 w3491 w3507 w3528] -> w3453
                        tunnel: w3452 -> [_ w3460 _ _ _ _]
                        tunnel: w3451 -> [_ _ w3480 w3495 w3516 w3537]
                        tunnel: w3450 -> [_ _ w3474 w3487 w3513 w3534]
                        tunnel: w3449 -> [_ _ w3476 w3494 _ _]
                        tunnel: [_ _ _ _ w3504 w3525] -> w3448
                        tunnel: [_ _ _ _ "" ""] -> w3447
                        tunnel: [_ _ _ _ w3500 w3521] -> w3446
                        tunnel: [_ _ _ _ w3497 w3518] -> w3445
                        frame "假", Default {
                        }
                        frame "TUID和证书编号入库" {
                          n790 = Match Pattern(string=w3460, regular expression=";") -> (before substring=w3458:string, after substring=w3457:string)  [unwired: 1 in, 2 out]
                          n791 = call "PCTuidToDB.vi"("TuidName"=w3457, "CertName"=w3458, "PathStr"=w3465) -> ("OK？"=w3464:bool)  [unwired: 7 in, 1 out]
                          n792 = Select(t="OK", s=w3464, f="NG") -> (s? t:f=w3462:string)
                        }
                        frame "CCID与SN入库" {
                          n793 = call <vilib>:"Trim Whitespace.vi"("string"=w3476) -> ("trimmed string"=w3470:string)  [unwired: 1 in]
                          n794 = To Upper Case(1:w3470) -> (0:w3469:string)
                          n795 = call "ccidinfo-r.vi"("Data Type"=PDINFO."CCID", "Slot"=w3474) -> ("Data"=w3478:string)
                          n796 = call "ccidinfo-r.vi"("Data Type"=PDINFO."Imei", "Slot"=w3474) -> ("Data"=w3475:string)
                          n797 = call "ccidinfo-r.vi"("Data Type"=PDINFO."AuthCode", "Slot"=w3474) -> ("Data"=w3472:string)
                          n798 = call <vilib>:"Trim Whitespace.vi"("string"=w3478) -> ("trimmed string"=w3468:string)  [unwired: 1 in]
                          n799 = call <vilib>:"Trim Whitespace.vi"("string"=w3475) -> ("trimmed string"=w3467:string)  [unwired: 1 in]
                          n800 = call <vilib>:"Trim Whitespace.vi"("string"=w3472) -> ("trimmed string"=w3466:string)  [unwired: 1 in]
                          n801 = call "WriteTestingDB.vi"("AuthCode"=w3466, "PartN"=w3480, "Imei"=w3467, "ICCID"=w3468, "SN"=w3469) -> ("ReportStrA"=w3481:string)  [unwired: 5 in, 1 out]
                          n802 = To Upper Case(1:w3481) -> (0:w3471:string)
                        }
                        frame "库中读TUID及证书编号" {
                          n803 = call "ccidinfo-r.vi"("Data Type"=PDINFO."CCID", "Slot"=w3487) -> ("Data"=w3493:string)
                          n804 = call <vilib>:"Trim Whitespace.vi"("string"=w3493) -> ("trimmed string"=w3484:string)  [unwired: 1 in]
                          n805 = call "ReadTuidCertid.vi"("ICCID"=w3484, "SN"=w3494, "PartN"=w3495) -> ("Certid"=w3485:string, "TUID"=w3488:string, "ReportStrA"=w3492:string)  [unwired: 5 in, 1 out]
                          n806 = call <vilib>:"Trim Whitespace.vi"("string"=w3485) -> ("trimmed string"=w3482:string)  [unwired: 1 in]
                          n807 = call <vilib>:"Trim Whitespace.vi"("string"=w3488) -> ("trimmed string"=w3483:string)  [unwired: 1 in]
                          n808 = To Upper Case(1:w3492) -> (0:w3491:string)
                          n809 = call "ccidinfo-w.vi"("Data"=w3483, "Data Type"=PDINFO."TUID", "Slot"=w3487) -> ()  [unwired: 1 in]
                          n810 = call "ccidinfo-w.vi"("Data"=w3482, "Data Type"=PDINFO."CertifID", "Slot"=w3487) -> ()  [unwired: 1 in]
                        }
                        frame "比较MAC地址" {
                          w3506 = "FAIL" ("DevT")
                          n811 = call "GetMAC.vi"("error in"=errorcluster {"status"=FALSE, "code"=0, "source"=""} ("错误常量"), "PartNum"=w3516, "DevT"="TBOX") -> ("error out"=w3505:errorcluster, "MAC"=w3503:string[])  [unwired: 7 in]
                          n812 = call "ccidinfo-r.vi"("Data Type"=PDINFO."Reserved3", "Slot"=w3513) -> ("Data"=w3511:string)
                          n813 = call <vilib>:"Trim Whitespace.vi"("string"=w3511) -> ("trimmed string"=w3501:string)  [unwired: 1 in]
                          n814 = Search 1D Array(1D array=w3503, element=w3501) -> (index of element=w3498:i32)  [unwired: 1 in]
                          n815 = Concatenate Strings("MAC:" ("DevT"), w3501) -> (w3500:string)
                          n816 = Not Equal?(x=w3498, y=-1) -> (x != y?=w3499:bool)
                          n817 = Select(t=w3506, s=w3499, f="PASS" ("DevT")) -> (s? t:f=w3508:string)
                          n818 = Unbundle By Name(w3505) -> ("source"=w3504:string)
                          n819 = Number To Decimal String(number=w3498) -> (decimal integer string=w3497:string)  [unwired: 1 in]
                          n820 = Select(t=w3506, s=w3505, f=w3508) -> (s? t:f=w3507:string)
                        }
                        frame "比较IMSI号" {
                          w3527 = "FAIL" ("DevT")
                          n821 = call "GetIMEI.vi"("error in"=errorcluster {"status"=FALSE, "code"=0, "source"=""} ("错误常量"), "PartNum"=w3537, "DevT"="TBOX") -> ("error out"=w3526:errorcluster, "IMSI"=w3524:string[])  [unwired: 7 in]
                          n822 = call "ccidinfo-r.vi"("Data Type"=PDINFO."Imei", "Slot"=w3534) -> ("Data"=w3532:string)
                          n823 = call <vilib>:"Trim Whitespace.vi"("string"=w3532) -> ("trimmed string"=w3522:string)  [unwired: 1 in]
                          n824 = Search 1D Array(1D array=w3524, element=w3522) -> (index of element=w3519:i32)  [unwired: 1 in]
                          n825 = Concatenate Strings("IMSI:" ("DevT"), w3522) -> (w3521:string)
                          n826 = Not Equal?(x=w3519, y=-1) -> (x != y?=w3520:bool)
                          n827 = Select(t=w3527, s=w3520, f="PASS" ("DevT")) -> (s? t:f=w3529:string)
                          n828 = Unbundle By Name(w3526) -> ("source"=w3525:string)
                          n829 = Number To Decimal String(number=w3519) -> (decimal integer string=w3518:string)  [unwired: 1 in]
                          n830 = Select(t=w3527, s=w3526, f=w3529) -> (s? t:f=w3528:string)
                        }
                      }
                    }
                  }
                }
              }
              n831 = Concatenate Strings(w3372, w3378, ": ", w3376, w3368, w3371, w3368, w3370, w3368, w3369, w3368, w3367) -> (w3375:string)
              n832 = String Length(string=w3375) -> (length=w3374:i32)
              n833 = call "TableHandle.vi"("All"=w3389, "error in (no error)"=w3386, "字符串数值"=FALSE, "DataIn"=w3376) -> ("error out"=w3391:errorcluster, "Stop?"=w3390:bool, "StopForLoop"=w3373:bool)  [unwired: 3 in, 2 out]
              n834 = property class="Str"(reference=w3379, "Text.Text"=w3375, "Text.Scroll Position"=w3374) -> ()  [unwired: 1 in, 2 out]
            }
          }
        }
      }
      frame "WIFI_DOS" {
        n835 = case shown="真" w3553 {
          tunnel: w3556 -> [w3560 w3574]
          tunnel: w3555 -> [w3561 w3576]
          tunnel: [w3562 w3575] -> w3554
          tunnel: [w3559 w3573] -> w3552
          tunnel: w3551 -> [_ w3572]
          tunnel: w3550 -> [_ w3571]
          tunnel: w3549 -> [_ w3570]
          tunnel: w3548 -> [_ w3569]
          tunnel: w3543 -> [w3557 w3568]
          tunnel: w3542 -> [_ w3567]
          tunnel: [w3557 w3566] -> w3541
          tunnel: w3540 -> [_ w3565]
          tunnel: w3539 -> [_ w3564]
          tunnel: w3538 -> [_ w3563]
          frame False {
            n836 = call "TableHandle.vi"("All"=w3560, "error in (no error)"=w3561, "DataIn"=TRUE) -> ("error out"=w3562:errorcluster, "Stop?"=w3559:bool)  [unwired: 3 in, 4 out]
          }
          frame True {
            n837 = for "For循环" {
              N: w3569 -> [_]
              tunnel: w3576 -> [w3630]
              tunnel: [w3634] -> w3575
              tunnel: w3574 -> [w3631]
              tunnel: [w3632] -> w3573
              tunnel: w3572 -> [w3584]
              tunnel: w3570 -> [w3604]
              tunnel: w3571 -> [w3608]
              shift-right: [w3616] -> w3566
              shift-left: w3568 -> [w3619]
              tunnel: w3567 -> [w3618]
              tunnel: w3565 -> [w3599]
              tunnel: w3564 -> [w3583]
              tunnel: w3563 -> [w3582]
              i -> [w3615]
              stop <- w3633 stop-if-true
              w3612 = "\n"
              n838 = property class="Ring (严格)"(reference=w3599) -> ("RingText.Text"=w3598:string)  [unwired: 1 in, 2 out]
              n839 = Match Pattern(string=w3604, regular expression=";") -> (before substring=w3603:string, after substring=w3602:string)  [unwired: 1 in, 2 out]
              n840 = case shown="\"Slot1\", 默认" w3584 {
                tunnel: [w3653 w3654] -> w3595
                frame "Slot1", Default {
                  n841 = global read "GlobalValue.vi" "Slot1USBCOM"() -> (w3653:refnum<visa-resource-name>)
                }
                frame "Slot2" {
                  n842 = global read "GlobalValue.vi" "Slot2USBCOM"() -> (w3654:refnum<visa-resource-name>)
                }
              }
              n843 = Match Pattern(string=w3608, regular expression=";") -> (before substring=w3606:string, after substring=w3590:string)  [unwired: 1 in, 2 out]
              n844 = Fract/Exp String To Number(string=w3603) -> (number=w3628:dbl)  [unwired: 3 in, 1 out]
              n845 = Multiply(x=w3628, y=1000.0) -> (x*y=w3627:dbl)
              n846 = Decimal String To Number(string=w3602) -> (number=w3601:i32)  [unwired: 2 in, 1 out]
              n847 = To Unsigned Long Integer(number=w3627) -> (unsigned 32bit integer=w3622:u32)
              n848 = case shown="1, 默认" w3615 {
                tunnel: w3630 -> [w3655 w3658]
                tunnel: w3622 -> [_ w3657]
                tunnel: [w3655 w3656] -> w3596
                frame 0 {
                }
                frame 1, Default {
                  n849 = call "WaitTimes.vi"("WaitTimes"=w3657, "error in (no error)"=w3658) -> ("error out"=w3656:errorcluster)  [unwired: 9 in]
                }
              }
              n850 = Match Pattern(string=w3590, regular expression=";") -> (after substring=w3588:string)  [unwired: 1 in, 3 out]
              n851 = Equal?(x=w3588, y="0") -> (x = y?=w3586:bool)
              n852 = call "ccidinfo-r.vi"("Data Type"=PDINFO."WiFiName", "Slot"=w3584) -> ("Data"=w3610:string)
              n853 = call "ccidinfo-r.vi"("Data Type"=PDINFO."WiFiPassword", "Slot"=w3584) -> ("Data"=w3609:string)
              n854 = call "RegisterCheck.vi"("error in"=w3596, "CMD2"="AT+CGREG?", "CMD1"="AT+CREG?", "COMIn"=w3595) -> ("error out"=w3592:errorcluster, "反馈"=w3591:string, "Result"=w3580:bool)  [unwired: 5 in]
              n855 = Or(x=w3580, y=w3586) -> (x .or. y?=w3585:bool)
              n856 = case shown="真" w3585 {
                selector: w3585 -> [w3639 _]
                tunnel: [w3639 w3652] -> w3621
                tunnel: [w3638 w3651] -> w3620
                tunnel: [w3637 w3640] -> w3611
                tunnel: w3610 -> [_ w3650]
                tunnel: w3609 -> [_ w3649]
                tunnel: w3606 -> [_ w3648]
                tunnel: w3590 -> [_ w3647]
                tunnel: w3601 -> [_ w3646]
                tunnel: 0.5 ("Delay Time (s)") -> [_ w3645]
                tunnel: w3598 -> [_ w3644]
                tunnel: w3592 -> [w3638 w3643]
                tunnel: w3591 -> [w3637 w3642]
                frame False {
                }
                frame True {
                  n857 = call "WiFi.vi"("New WIFI Name"=w3650, "DelayTime (s)"=w3645, "配置连接次数"=w3646, "Delay"=w3648, "password"=w3649, "error in"=w3643, "ping次数"=w3647, "ModelNumber"=w3644) -> ("Acess"=w3652:bool, "TotalOut"=w3641:string, "error out"=w3651:errorcluster)  [unwired: 5 in]
                  n858 = Concatenate Strings(w3642, w3641) -> (w3640:string)
                }
              }
              n859 = case shown="\"Slot2\"" w3584 {
                tunnel: w3583 -> [w3635 _]
                tunnel: w3582 -> [_ w3636]
                tunnel: [w3635 w3636] -> w3581
                frame "Slot1", Default {
                }
                frame "Slot2" {
                }
              }
              n860 = Concatenate Strings(w3619, "WIFI名:", w3610, w3612, "WIFI密码:", w3609, w3612, w3611) -> (w3616:string)
              n861 = Select(t=LEDState."真" ("State"), s=w3580, f=LEDState."假" ("State")) -> (s? t:f=w3577:T7)
              n862 = String Length(string=w3616) -> (length=w3617:i32)
              n863 = property class="Str"(reference=w3618, "Value"=w3616, "Text.Scroll Position"=w3617) -> ()  [unwired: 1 in, 2 out]
              n864 = Select(t="PASS", s=w3621, f="FAIL") -> (s? t:f=w3626:string)
              n865 = call "三态LED.vi"("State"=w3577, "Ctl引用句柄"=w3581) -> ()  [unwired: 4 in, 2 out]
              n866 = call "TableHandle.vi"("All"=w3631, "error in (no error)"=w3620, "DataIn"=w3626) -> ("error out"=w3634:errorcluster, "Stop?"=w3632:bool, "StopForLoop"=w3633:bool)  [unwired: 4 in, 2 out]
            }
          }
        }
      }
      frame "Wait" {
      }
      frame "Wifi_Ping" {
        n867 = case shown="真" w3678 {
          tunnel: w3681 -> [w3685 w3696]
          tunnel: w3680 -> [w3686 w3698]
          tunnel: [w3687 w3697] -> w3679
          tunnel: [w3684 w3695] -> w3677
          tunnel: w3676 -> [_ w3694]
          tunnel: w3675 -> [_ w3693]
          tunnel: w3674 -> [_ w3692]
          tunnel: w3673 -> [_ w3691]
          tunnel: w3668 -> [w3682 w3690]
          tunnel: w3667 -> [_ w3689]
          tunnel: [w3682 w3688] -> w3666
          frame False {
            n868 = call "TableHandle.vi"("All"=w3685, "error in (no error)"=w3686, "DataIn"=TRUE) -> ("error out"=w3687:errorcluster, "Stop?"=w3684:bool)  [unwired: 3 in, 4 out]
          }
          frame True {
            n869 = for "For循环" {
              N: w3691 -> [_]
              tunnel: w3698 -> [w3725]
              tunnel: [w3729] -> w3697
              tunnel: w3696 -> [w3726]
              tunnel: [w3727] -> w3695
              tunnel: w3694 -> [w3715]
              tunnel: w3692 -> [w3723]
              tunnel: w3693 -> [w3712]
              shift-right: [w3706] -> w3688
              shift-left: w3690 -> [w3709]
              tunnel: w3689 -> [w3708]
              i -> [w3705]
              stop <- w3728 stop-if-true
              w3700 = "\n"
              n870 = Fract/Exp String To Number(string=w3723) -> (number=w3722:dbl)  [unwired: 3 in, 1 out]
              n871 = Multiply(x=w3722, y=1000.0) -> (x*y=w3721:dbl)
              n872 = To Unsigned Long Integer(number=w3721) -> (unsigned 32bit integer=w3714:u32)
              n873 = case shown="1, 默认" w3705 {
                tunnel: w3725 -> [w3730 w3733]
                tunnel: w3714 -> [_ w3732]
                tunnel: [w3730 w3731] -> w3713
                frame 0 {
                }
                frame 1, Default {
                  n874 = call "WaitTimes.vi"("WaitTimes"=w3732, "error in (no error)"=w3733) -> ("error out"=w3731:errorcluster)  [unwired: 9 in]
                }
              }
              n875 = call "ccidinfo-r.vi"("Data Type"=PDINFO."WiFiPassword", "Slot"=w3715) -> ("Data"=w3701:string)
              n876 = call "ccidinfo-r.vi"("Data Type"=PDINFO."WiFiName", "Slot"=w3715) -> ("Data"=w3703:string)
              n877 = call "WifiConnect.vi"("连接延时"=w3714, "error in"=w3713, "cmd"=w3712, "Password"=w3701, "WifiName"=w3703) -> ("error out"=w3710:errorcluster, "Out"=w3699:string, "Result？"=w3711:bool)  [unwired: 3 in, 1 out]
              n878 = Concatenate Strings(w3709, "WIFI名:", w3703, w3700, "WIFI密码:", w3701, w3700, w3699) -> (w3706:string)
              n879 = String Length(string=w3706) -> (length=w3707:i32)
              n880 = property class="Str"(reference=w3708, "Value"=w3706, "Text.Scroll Position"=w3707) -> ()  [unwired: 1 in, 2 out]
              n881 = Select(t="PASS", s=w3711, f="FAIL") -> (s? t:f=w3720:string)
              n882 = call "TableHandle.vi"("All"=w3726, "error in (no error)"=w3710, "DataIn"=w3720) -> ("error out"=w3729:errorcluster, "Stop?"=w3727:bool, "StopForLoop"=w3728:bool)  [unwired: 4 in, 2 out]
            }
          }
        }
      }
      frame "幅度DB" {
        n883 = case shown="真" w3745 {
          tunnel: w3748 -> [w3752 w3761]
          tunnel: w3747 -> [w3753 w3763]
          tunnel: [w3754 w3762] -> w3746
          tunnel: [w3751 w3760] -> w3744
          tunnel: w3743 -> [_ w3759]
          tunnel: w3742 -> [_ w3758]
          tunnel: w3741 -> [_ w3757]
          tunnel: w3740 -> [_ w3756]
          tunnel: w3739 -> [w3749 w3755]
          tunnel: [w3749 w3755] -> w3738
          frame False {
            n884 = call "TableHandle.vi"("All"=w3752, "error in (no error)"=w3753, "DataIn"=TRUE) -> ("error out"=w3754:errorcluster, "Stop?"=w3751:bool)  [unwired: 3 in, 4 out]
          }
          frame True {
            n885 = for "For循环" {
              N: w3756 -> [_]
              tunnel: w3763 -> [w3767]
              tunnel: [w3772] -> w3762
              tunnel: w3761 -> [w3769]
              tunnel: [w3770] -> w3760
              tunnel: w3759 -> [_]
              tunnel: w3757 -> [_]
              tunnel: w3758 -> [_]
              tunnel: w3755 -> [w3768]
              stop <- w3771 stop-if-true
              n886 = call-poly <vilib>:"Basic Averaged DC-RMS.vi"("error in (no error)"=w3767, "signal in"=w3768) -> ("error out"=w3766:errorcluster, "RMS value"=w3765:dbl)  [unwired: 6 in, 2 out]
              n887 = expression code="20*log(x)"(w3765) -> (w3764:dbl)
              n888 = call "TableHandle.vi"("All"=w3769, "error in (no error)"=w3766, "DataIn"=w3764) -> ("error out"=w3772:errorcluster, "Stop?"=w3770:bool, "StopForLoop"=w3771:bool)  [unwired: 4 in, 2 out]
            }
          }
        }
      }
      frame "空", Default {
        # "此步骤不能删除"
        n889 = case shown="\"Slot4\"" w3776 {
          tunnel: ["Slot1 " ("字符串") "Slot2 " ("字符串") "Slot3 " ("字符串") "Slot4 " ("字符串")] -> w3775
          frame "Slot1", Default {
          }
          frame "Slot2" {
          }
          frame "Slot3" {
          }
          frame "Slot4" {
          }
        }
        n890 = Concatenate Strings(w3775, "Cann't find the \"" ("source"), w3781, "\" item." ("字符串")) -> (w3780:string)
        n891 = Bundle By Name(cluster=errorcluster {"status"=TRUE, "code"=5000, "source"=""} ("error in 1 (no error)"), "source"=w3780) -> (w3785:errorcluster)
      }
    }
  }
  "error out" <- w9
